vi "Maintenance4ChBK.vi"() -> ()   [LabVIEW 2020]
doc: "Maintanence VI for FLS imaging system.\n[Covers: REQ9]\n[Covers: REQ10]"
uses:
  SubVI/DigitizerConfiguration/FLImDAQ.ctl
  <instrlib>/niScope/Controls/niScope trigger source.ctl
  SubVI/LabJack/LJ Pin Setting.ctl
  <vilib>/addons/control/pid/autopid.llb/PID autotuning parameters.ctl
  LaguerreDeconLib/DeconEngineClass/LaguerreDeconEngineClass.lvclass/LaguerreDeconEngineClass.ctl
  <vilib>/Utility/error.llb/DialogType.ctl
  <vilib>/event_ctls.llb/usereventprio.ctl
  <vilib>/Utility/miscctls.llb/LVRowAndColumnTypeDef.ctl
  <vilib>/Utility/miscctls.llb/LVMinMaxIncTypeDef.ctl
  SubVI/APD/APDClass.lvclass
  SubVI/APD/GainData.ctl
  SubVI/APD/iRFData.ctl
  <vilib>/Analysis/baseanly.llb/Mean (DBL).vi
  SubVI/GlobalVariables.vi
  <vilib>/addons/control/pid/autopid.llb/PID Online Autotuning (Step Closed Loop).vi
  <vilib>/addons/control/pid/pid.llb/PID Advanced (DBL).vi
  <instrlib>/niScope/Acquire/Fetch/niScope Multi Fetch Binary 16.vi
  <vilib>/Instr/_visa.llb/VISA Configure Serial Port (Instr).vi
  <userlib>/_OpenG.lib/file/file.llb/openg_file.lvlib
  <userlib>/_OpenG.lib/time/time.llb/openg_time.lvlib
  <vilib>/Analysis/NI_AALBase.lvlib
  LaguerreDeconLib/DeconEngineClass/LaguerreDeconEngineClass.lvclass
  <vilib>/Utility/miscctls.llb/LVPointTypeDef.ctl
  <vilib>/addons/control/pid/NI_PID_autopid.lvlib
  <vilib>/addons/control/pid/NI_PID_pid.lvlib
panel:
  in  "Duty Cycle (%)":u32=25
  in  "AB Rep Rate":u16 caption="Rep Rate" max=1000 step=1 format="%.0dHz"
  in  "Current":dbl=1.0 min=1.0 max=63.0 step=1.0 format="%#.1fA"
  out "GainIndicator":dbl caption="Gain"
  out "Noise\n(std of DC)":dbl format="%0.6f"
  in  "BG flag?":bool
  out "DC":dbl format="%0.2f"
  out "Amplitude":dbl
  in  "Gain High":dbl max=4.5
  in  "Gain low":dbl=3.0
  in  "Step":dbl=0.1
  in  "Num WF to acquire":u64=18446744073709551615
  in  "Channel":enum32{"Ch1", "Ch2", "Ch3", "Ch4"}(radio)
  in  "Task":enum32{"iRFAndGain", "Alignment"}(radio)
  in  "Aiming beam toggle":bool caption="445nm 100Hz"
  in  "Laser Rep Rate":u16=120 caption="Rep Rate" min=5 max=4000 step=1 format="%.0dHz"
  in  "355nm Laser toggle":bool caption="355nm 460Hz"
  out "appended path":path
  out "Current State":string
  out "WF max value":dbl
  out "Disclamer":picture
  out "Calibration #":i8
  out "BG #":i8
  in  "TCP Connect":bool
  out "Help":string
  in  "Auto gain":bool=TRUE
  out "Run #":i8
  in  "StopButton":bool caption="Stop"
  out "System Status:":bool
  in  "StartButton":bool caption="Start"
  in  "Ctrl V":dbl=0.05 min=0.0 max=5.5 step=0.009999999776482582 format="%#.3f"
  out "System Hardware Connection Status":T1
  out "Waveform (no average)":dbl[](graph)
  in  "Tab Control":T2(tab)
  out "Ch1 Max CtrlV":dbl
  out "Ch1 iRF Graph":dbl[][](graph)
  out "Ch1 Gain":cluster{"CtrlV":dbl[], "Gain":dbl[]}(graph)
  out "Serial Number Ch1":string caption="Serial Number"
  out "DateTimeCh1":string caption="DateTime"
  out "Ch2 Gain":cluster{"CtrlV":dbl[], "Gain":dbl[]}(graph)
  out "Ch2 iRF Graph":dbl[][](graph)
  out "Ch2 Max CtrlV":dbl
  out "Serial Number Ch2":string caption="Serial Number"
  out "DateTimeCh2":string caption="DateTime"
  out "Ch3 iRF Graph":dbl[][](graph)
  out "Ch3 Gain":cluster{"CtrlV":dbl[], "Gain":dbl[]}(graph)
  out "Serial Number Ch3":string caption="Serial Number"
  out "Ch3 Max CtrlV":dbl
  out "DateTimeCh3":string caption="DateTime"
  out "Ch4 iRF Graph":dbl[][](graph)
  out "Ch4 Gain":cluster{"CtrlV":dbl[], "Gain":dbl[]}(graph)
  out "Serial Number Ch4":string caption="Serial Number"
  out "Ch4 Max CtrlV":dbl
  out "DateTimeCh4":string caption="DateTime"
  out "display loop timing(ms)":u32
  out "Aquisition loop timing(ms)":u32
  out "DisplayLoop":i32
  out "processing loop":i32
  out "processing loop timing(ms)":dbl
  out "laser EM lamp V":dbl format="%0.6f"
  out "aquisition loop Error Out":errorcluster
  out "Aq Loop?":bool
  out "processing Error Out":errorcluster
  out "Triggering:Trigger Delay":dbl
  out "Foot Pedal":bool
  out "LJ Pinout":T3={"Ch1 Bias"="DAC0", "Ch2 Bias"="DAC1", "Ch3 Bias"="DAC2", "Ch4 Bias"="DAC0", "355 PWM"="FIO0", "AimingBeam PWM"="FIO2", "Laser Ready"="FIO3", "Interlock"="FIO1", "Laser Start/Stop"="FIO1", "Red LED"="FIO1", "Green LED"="DIO3", "Foot Pedal"="DIO15"}
  out "FLImDAQ":T4={"Digitizer 1"="", "Digitizer 2"="", "Channel"=enum."Channel 0", "trigger source"="VAL_EXTERNAL", "trigger level"=0.5, "trigger delay"=1.35e-07, "min sample rate"=12500000000.0, "min record length"=2500, "vertical range"=1.0, "vertical offset"=-0.25, "Waveform to Avg"=2000} caption="FLIm DAQ Configuration" {"trigger delay" format="%^#.4e"; "trigger level" min=0.0 max=3.5 step=0.5 format="%.2f"; "vertical offset" format="%.4f"; "vertical range" format="%.2f"; "min sample rate" format="%#.2p"}
  out "Dig1 Temp":dbl
  out "Dig2 Temp":dbl
  in  "Sys Reconfig":bool
  out "Fetch Record #":i32
  out "Record Backlog":i32
  out "Fetch:Records Done":i32
  out "dt (s)":dbl format="%#_6p"
  out "Fetch:Records Done 2":i32
  in  "SaveData?":bool
  out "data Size":i32[](array[numeric])
  out "numWFInQ":i32
  in  "Clear WF Chart History":bool
  out "Waveform Chart":dbl(graph)
  in  "SaveiRFData":bool
  out "iRFDataTable":string[][](table)
  in  "SetIRFCtrlV":bool
  in  "ClearIRFData":bool
  in  "AcquireIRF":bool
  out "iRFInstSting":string="To aquire gain data, please start data aquisition! \nPlace blue (Ch1&2) or Green(Ch3) Chroma slide as close as possible to the fiber port! \nPlease remove channel 3 bandpass filter as well!"
  out "iRFSigInRange":bool caption="Signal  In Range?"
  out "Current iRF":dbl[](graph)
  out "iRFCtrlV":dbl[](array[numeric])
  in  "SaveGainData":bool
  out "GainInstSting":string="To aquire gain data, please start data aquisition! \nPlace blue (Ch1&2) or Green(Ch3) Chroma slide as close as possible to the fiber port! \nPlease remove channel 3 bandpass filter as well!"
  in  "ClearGainData":bool
  out "Gain":dbl[](array[numeric])
  in  "ComputeGain":bool
  out "Int Corr AUC":dbl[](array[numeric])
  out "AUC Std":dbl[](array[numeric])
  out "GainSigInRange":bool caption="Signal  In Range?"
  in  "AcquireGain":bool
  out "GainDataTable":string[][](table)
  out "Intensity Factor":dbl[](array[numeric])
  out "AUC":dbl[](array[numeric])
  out "Ctrl V":dbl[](array[numeric])
  out "XY Graph":cluster{"Ctrl V":dbl[], dbl[]}(graph)
  in  "Ch4 PID gains":T6={"proportional gain (Kc)"=0.5, "integral time (Ti, min)"=0.0003, "derivative time (Td, min)"=1e-05} {"derivative time (Td, min)" format="%.6f"; "integral time (Ti, min)" format="%.6f"; "proportional gain (Kc)" format="%.6f"}
  in  "Save PID":bool
  out "Targer and Max":cluster{"V target(1.0)":dbl, dbl}(graph)
  out "Completed?":bool
  out "Gain(Log10)":dbl(graph)
  in  "Gain(Log)":dbl=1.0
  in  "Ch1 PID gains":T6={"proportional gain (Kc)"=0.5, "integral time (Ti, min)"=0.0003, "derivative time (Td, min)"=1e-05} {"derivative time (Td, min)" format="%.6f"; "integral time (Ti, min)" format="%.6f"; "proportional gain (Kc)" format="%.6f"}
  in  "autotune? (F)":bool
  in  "PID dt (s)":dbl=-1.0
  out "dt out (s)":dbl format="%.3f"
  in  "V target(1.0)":dbl=1.0 format="%#_2f"
  in  "Accept?":bool
  out "tuned PID gains":T6={"proportional gain (Kc)"=1.0, "integral time (Ti, min)"=0.01, "derivative time (Td, min)"=0.0} {"derivative time (Td, min)" format="%_6f"; "integral time (Ti, min)" format="%.6f"; "proportional gain (Kc)" format="%.6f"}
  in  "autotuning parameters":T7={"type of controller"=2, "relay cycles"=100, "relay amplitude"=0.25, "control specifications"=1, "PV noise level"=0.01} {"PV noise level" format="%.5f"; "control specifications" items=["normal", "fast", "slow"]; "relay amplitude" format="%.2f"; "type of controller" items=["P", "PI", "PID"]}
  in  "Ch2 PID gains":T6={"proportional gain (Kc)"=0.5, "integral time (Ti, min)"=0.0003, "derivative time (Td, min)"=1e-05} {"derivative time (Td, min)" format="%.6f"; "integral time (Ti, min)" format="%.6f"; "proportional gain (Kc)" format="%.6f"}
  in  "Ch3 PID gains":T6={"proportional gain (Kc)"=0.5, "integral time (Ti, min)"=0.0003, "derivative time (Td, min)"=1e-05} {"derivative time (Td, min)" format="%.6f"; "integral time (Ti, min)" format="%.6f"; "proportional gain (Kc)" format="%.6f"}
  in  "gamma":dbl=1.0 format="%.2f"
  in  "alpha":dbl=nan format="%.2f"
  in  "Quit":bool
  # "440nm Laser Setting"
  # "355nm Laser Setting"
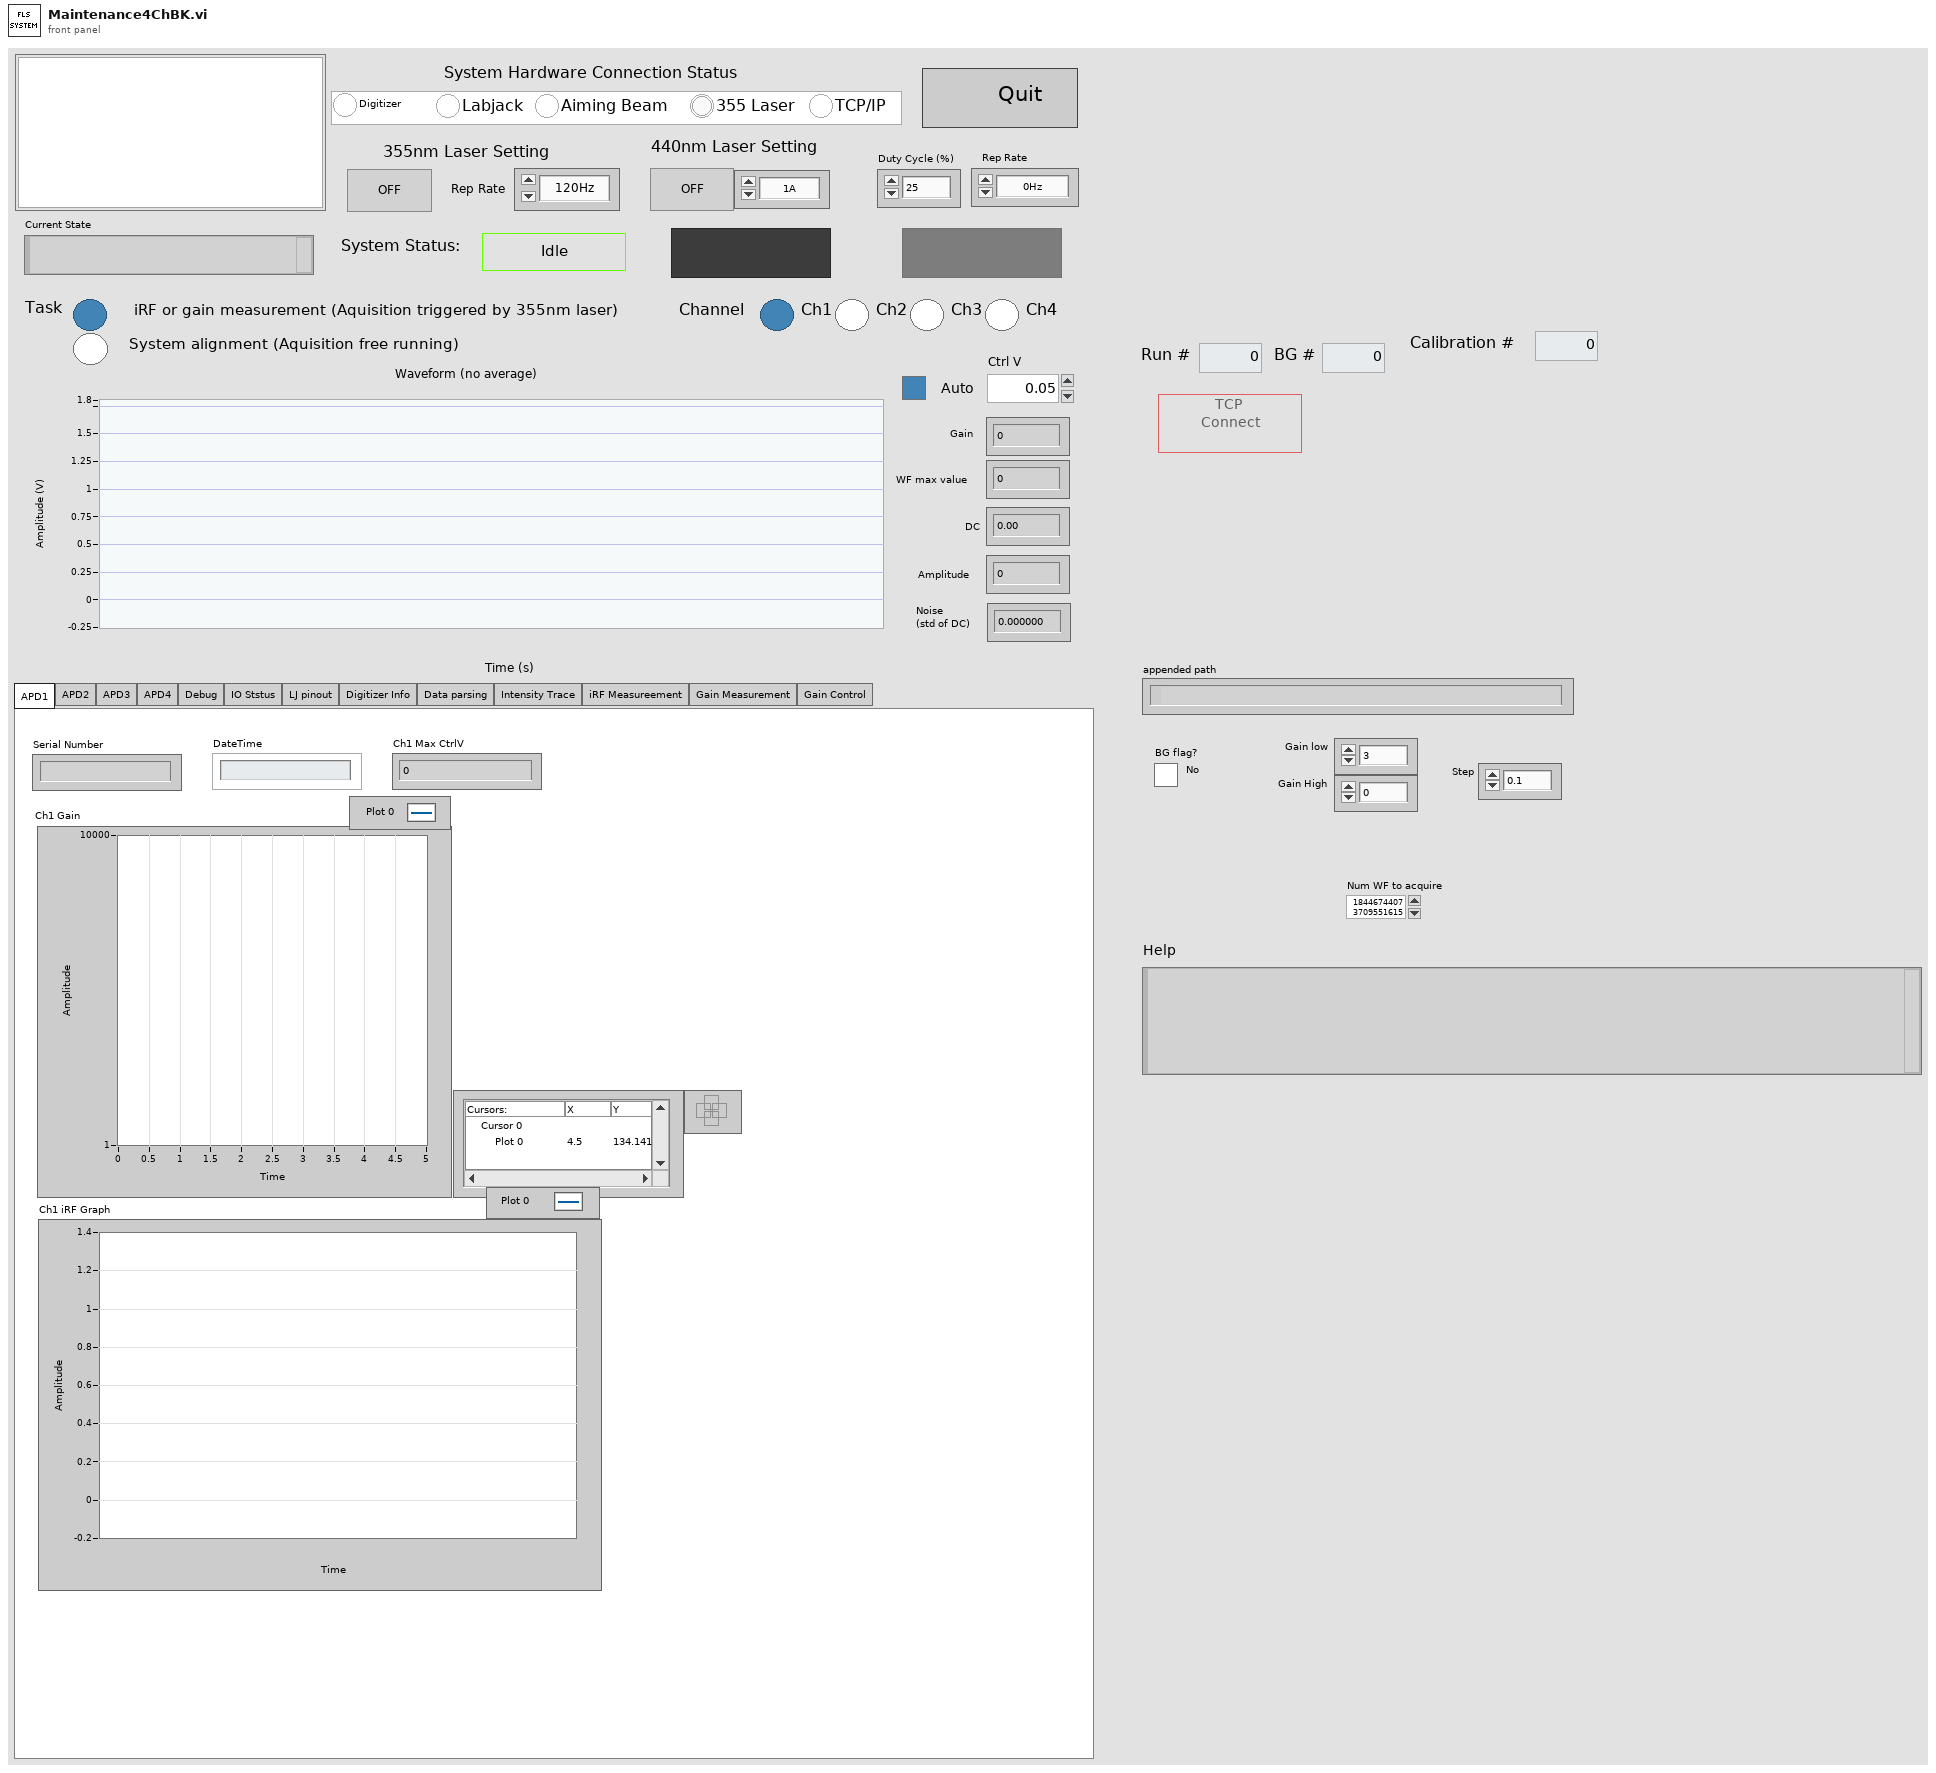
[diagram p1: front panel]
types:
  T1 = cluster{"Digitizer":bool, "Labjack":bool, "Aiming Beam":bool, "355 Laser":bool, "TCP/IP":bool}
  T2 = enum32{"APD1", "APD2", "APD3", "APD4", "Debug", "IO Ststus", "LJ pinout", "Digitizer Info", "Data parsing", "Intensity Trace", "iRF Measureement", "Gain Measurement", "Gain Control"}
  T3 = typedef "LJ Pin Setting.ctl" = cluster{"Ch1 Bias":string, "Ch2 Bias":string, "Ch3 Bias":string, "Ch4 Bias":string, "355 PWM":string, "AimingBeam PWM":string, "Laser Ready":string, "Interlock":string, "Laser Start/Stop":string, "Red LED":string, "Green LED":string, "Foot Pedal":string}
  T4 = typedef "FLImDAQ.ctl" = cluster{"Digitizer 1":refnum<k15>, "Digitizer 2":refnum<k15>, "Channel":enum16{"Channel 0", "Channel 1", "Channel 0&1"}, "trigger source":T5, "trigger level":dbl, "trigger delay":dbl, "min sample rate":dbl, "min record length":i32, "vertical range":dbl, "vertical offset":dbl, "Waveform to Avg":i16}
  T5 = typedef "niScope trigger source.ctl" = string
  T6 = cluster{"proportional gain (Kc)":dbl, "integral time (Ti, min)":dbl, "derivative time (Td, min)":dbl}
  T7 = typedef "PID autotuning parameters.ctl" = cluster{"type of controller":u16, "relay cycles":i32, "relay amplitude":dbl, "control specifications":u16, "PV noise level":dbl}
  T8 = cluster{"CtrlV":dbl, "WFs":dbl[][], "WFavg":dbl[]}
  T9 = enum16{"open", "replace", "create", "open or create", "replace or create", "replace or create with confirmation"}
  T10 = typedef "LVPointTypeDef.ctl" = cluster{"Horizontal":i16, "Vertical":i16}
  T11 = enum8{"Enabled", "Disabled", "Disabled and Grayed Out"}
  T12 = cluster{"CtrlV":dbl, "PeakV":dbl, "PeakV Std":dbl, "IntFactor":dbl, "IntCorrPeakV":dbl}
  T13 = enum16{"open", "open or create", "create or replace", "create", "open (read-only)"}
  T14 = enum32{"Invalid", "Standard", "Closed", "Hidden", "Minimized", "Maximized"}
  T15 = enum32{"invalid app kind", "Development System", "Run Time System", "Student Edition", "Embedded LabVIEW", "Evaluation", "Custom"}
  T16 = typedef "usereventprio.ctl" = enum32{"high priority", "normal priority"}
  T17 = enum32{"APD1", "APD2", "APD3", "Debug", "IO Ststus", "LJ pinout", "Digitizer Info", "Data parsing"}
  T18 = enum32{"Bad", "Idle", "Run top level", "Running"}
  T19 = typedef "LVRowAndColumnTypeDef.ctl" = cluster{"Row":i32, "Column":i32}
  T20 = typedef "LVMinMaxIncTypeDef.ctl" = cluster{"Minimum":dbl, "Maximum":dbl, "Increment":dbl}
  T21 = cluster{"Aiming Beam COM Port":refnum<visa-resource-name>, "Min Current":dbl, "Max Current":dbl, "Default Current":dbl, "Frequency(Hz)":i32}
  T22 = cluster{"Core":cluster{"Current VI Reference":refnum<vi>, "Close Panel on Exit?":bool}, "SysConfigCluster":cluster{"Ch1Enable?":bool, "Ch2Enable?":bool, "Ch3Enable?":bool, "Ch1AutoGain?":bool, "Ch2AutoGain?":bool, "Ch3AutoGain?":bool, "AimingBeamEnable?":bool}, "System Status":cluster{"Digitizer":bool, "Labjack":bool, "Aiming Beam":bool, "355 Laser":bool, "TCP/IP":bool}, "IDs":cluster{"RunID":i8, "BG ID":i8, "Cali ID":i8}, "DefaultPath":path, "Pathes":cluster{"DataPath":path, "BG Path":path, "iRFPath":path, "CaliPath":path}, "FLImDAQ":cluster{"resource name":refnum<k15>, "resource name 2":refnum<k15>, "Channel":enum16{"Channel 0", "Channel 1", "Channel 0&1"}, "trigger source":T5, "trigger level":dbl, "trigger delay":dbl, "min sample rate":dbl, "min record length":i32, "vertical range":dbl, "vertical offset":dbl, "Waveform to Avg":i32}, "SysRunning?":bool, "AB Cluster":cluster{"Aiming Beam COM Port":refnum<visa-resource-name>, "Min Current":dbl, "Max Current":dbl, "Default Current":dbl, "Frequency(Hz)":i32}, "LJ Pinout":T3, "355 PWM setting":cluster{"DIO_EF_CLOCK1_DIVISOR":i16, "DIO_EF_CLOCK1_ROLL_VALUE":i32, "DIO#_EF_INDEX":i16, "DIO#_EF_OPTIONS":i16, "DIO#_EF_CONFIG_A":i32}, "AB PWM setting":cluster{"DIO_EF_CLOCK1_DIVISOR":i16, "DIO_EF_CLOCK1_ROLL_VALUE":i32, "DIO#_EF_INDEX":i16, "DIO#_EF_OPTIONS":i16, "DIO#_EF_CONFIG_A":i32}, "Last Trigger":u32, "niTClk sessions":refnum<k20>[], "Laser start tic":u32, "TCP attempt count":i32, "iRFAllGain":dbl[][], "SlowTimer":u32, "FastTimer":u32, "TempPath":path, "LED vi reference":refnum<vi>, "APDSerials":cluster{"Ch1Serial":string, "Ch2Serial":string, "Ch3Serial":string, "Ch4Serial":string}, "LedViRefOpen":bool, "GainBGRaw":dbl[][], "GainDataTemp":cluster{"CtrlV":dbl, "AUC":dbl, "AUC Std":dbl, "IntFactor":dbl, "IntCorrAUC":dbl}, "iRFIdx":i32}
  T23 = cluster{"CtrlV":dbl, "AUC":dbl, "AUC Std":dbl, "IntFactor":dbl, "IntCorrAUC":dbl}
  T24 = cluster{"Ch1Serial":string, "Ch2Serial":string, "Ch3Serial":string, "Ch4Serial":string}
  T25 = cluster{"DataPath":path, "BG Path":path, "iRFPath":path, "CaliPath":path}
  T26 = cluster{"DIO_EF_CLOCK1_DIVISOR":i16, "DIO_EF_CLOCK1_ROLL_VALUE":i32, "DIO#_EF_INDEX":i16, "DIO#_EF_OPTIONS":i16, "DIO#_EF_CONFIG_A":i32}
  T27 = cluster{"resource name":refnum<k15>, "resource name 2":refnum<k15>, "Channel":enum16{"Channel 0", "Channel 1", "Channel 0&1"}, "trigger source":T5, "trigger level":dbl, "trigger delay":dbl, "min sample rate":dbl, "min record length":i32, "vertical range":dbl, "vertical offset":dbl, "Waveform to Avg":i32}
  T28 = cluster{"Ch1Enable?":bool, "Ch2Enable?":bool, "Ch3Enable?":bool, "Ch1AutoGain?":bool, "Ch2AutoGain?":bool, "Ch3AutoGain?":bool, "AimingBeamEnable?":bool}
  T29 = cluster{"Current VI Reference":refnum<vi>, "Close Panel on Exit?":bool}
  T30 = cluster{"iRF":dbl[], "iRF":dbl[], "iRF":dbl[], "iRF":dbl[]}
  T31 = typedef "DialogType.ctl" = u16
  T32 = typedef "LJ PWM Setting.ctl" = cluster{"DIO_EF_CLOCK1_DIVISOR":i16, "DIO_EF_CLOCK1_ROLL_VALUE":i32, "DIO#_EF_INDEX":i16, "DIO#_EF_OPTIONS":i16, "DIO#_EF_CONFIG_A":i32}
  T33 = typedef "AimingBeam.ctl" = cluster{"Aiming Beam COM Port":refnum<visa-resource-name>, "Min Current":dbl, "Max Current":dbl, "Default Current":dbl, "Frequency(Hz)":u32}
  T34 = typedef "LVBoundsTypeDef.ctl" = cluster{"Width":u32, "Height":u32}
  T35 = typedef "imagedata.ctl" = cluster{"image type":i32, "image depth":i32, "image":u8[], "mask":u8[], "colors":u32[], "Rectangle":cluster{"left":i16, "top":i16, "right":i16, "bottom":i16}}
  T36 = typedef "LVCursorListTypeDef.ctl" = cluster{"Name":string, "Color":u32, "Style":u8, "Point Style":u8, "Name Visible":bool, "Allow Drag":bool, "Cursor Mode":u32, "Plot":i32, "Index":i32, "Position":cluster{"X":dbl, "Y":dbl}, "X Scale":u32, "Y Scale":u32, "Watch Plots":i32[], "Watch All Plots":bool, "Plot Area":i32, "Label Offset":cluster{"X":dbl, "Y":dbl}}[]
  T37 = cluster{"Name":string, "Color":u32, "Style":u8, "Point Style":u8, "Name Visible":bool, "Allow Drag":bool, "Cursor Mode":u32, "Plot":i32, "Index":i32, "Position":cluster{"X":dbl, "Y":dbl}, "X Scale":u32, "Y Scale":u32, "Watch Plots":i32[], "Watch All Plots":bool, "Plot Area":i32, "Label Offset":cluster{"X":dbl, "Y":dbl}}
  T38 = cluster{"Name":string, "Color":u32, "Style":u8, "Point Style":u8, "Name Visible":bool, "Allow Drag":bool, "Cursor Mode":u32, "Plot":i32, "Index":i32, "Position":cluster{"X":dbl, "Y":dbl}, "X Scale":u32, "Y Scale":u32, "Watch Plots":i32[], "Watch All Plots":bool, "Plot Area":i32, "Label Offset":cluster{"X":dbl, "Y":dbl}}[]
  T39 = cluster{"Ch1APDSerial#":string, "Ch2APDSerial#":string, "Ch3APDSerial#":string, "Ch4APDSerial#":string}
  T40 = typedef "GainData.ctl" = cluster{"CtrlV":dbl[], "NumOfWFs":i32, "WF length":i32, "Gain":dbl[], "GainRaw":dbl[][], "GainBGRaw":dbl[][]}
  T41 = typedef "iRFData.ctl" = cluster{"dt":dbl, "NumOfWFs":i32, "WFLength":i32, "iRFCtrlV":dbl[], "iRFWFsAvg":dbl[][], "iRFRaw":dbl[][]}
  T42 = cluster{"CtrlV":dbl, "WFs":dbl[][], "WFavg":dbl[]}[]
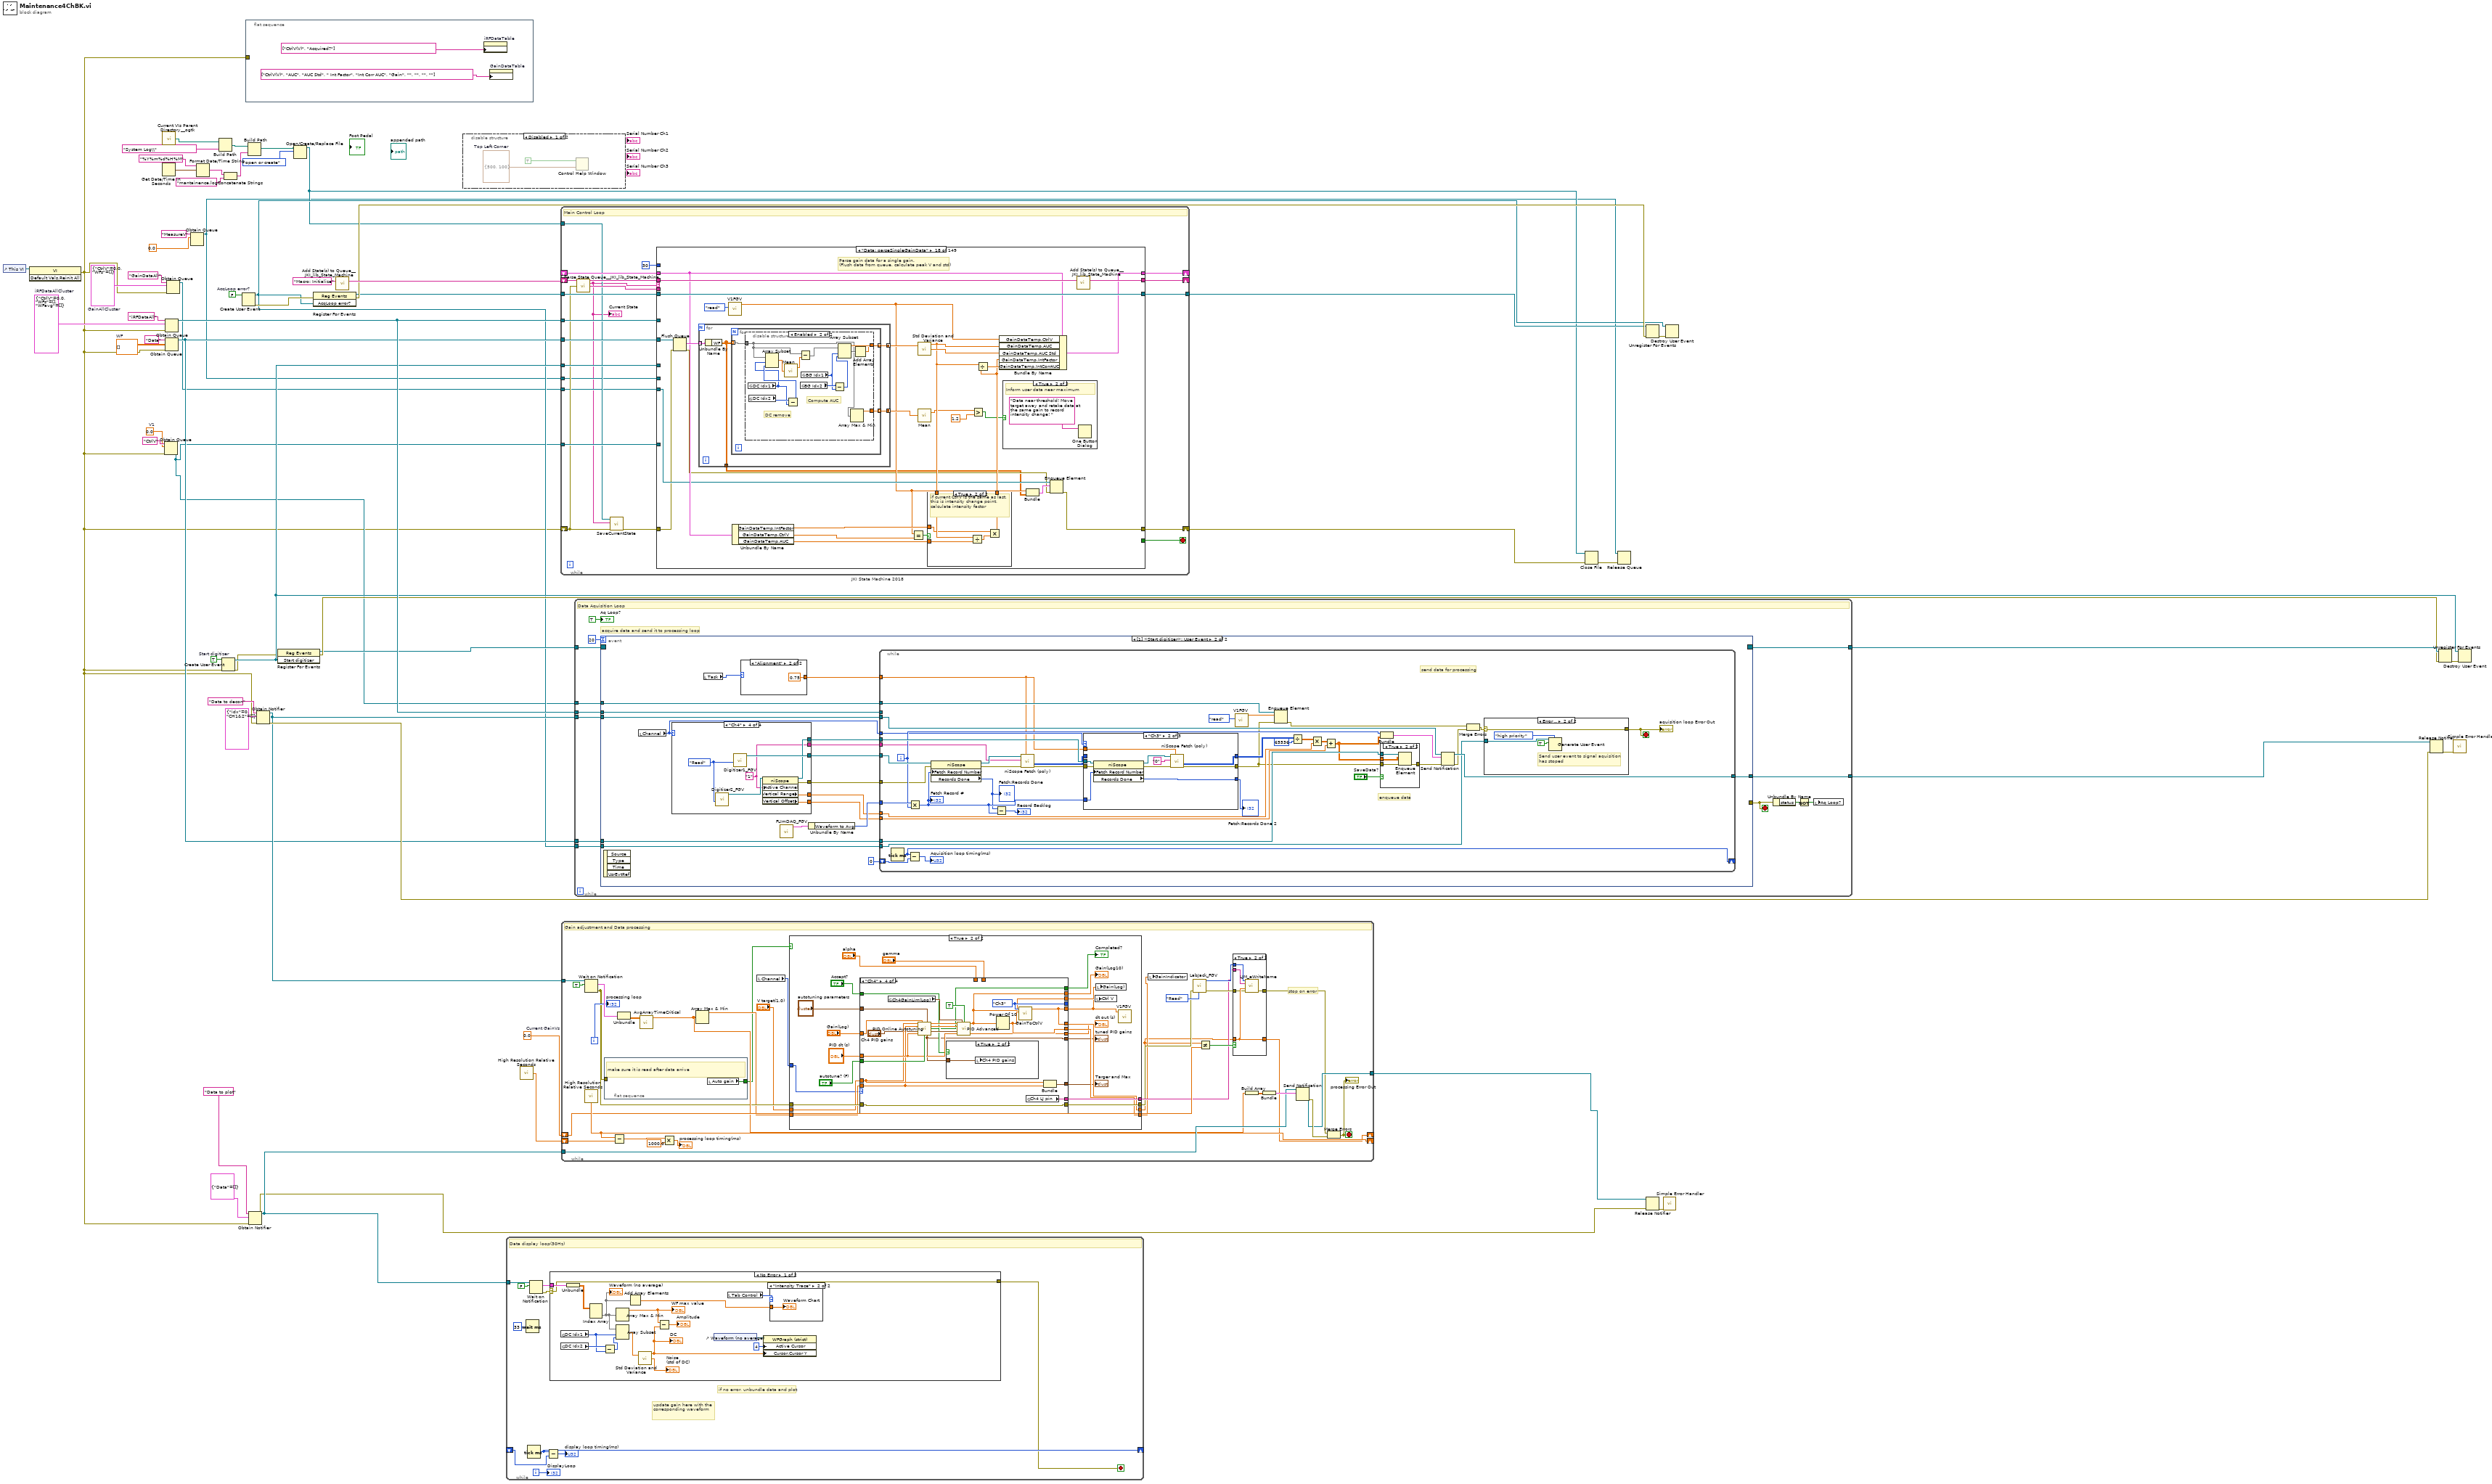
[diagram p0: block diagram]
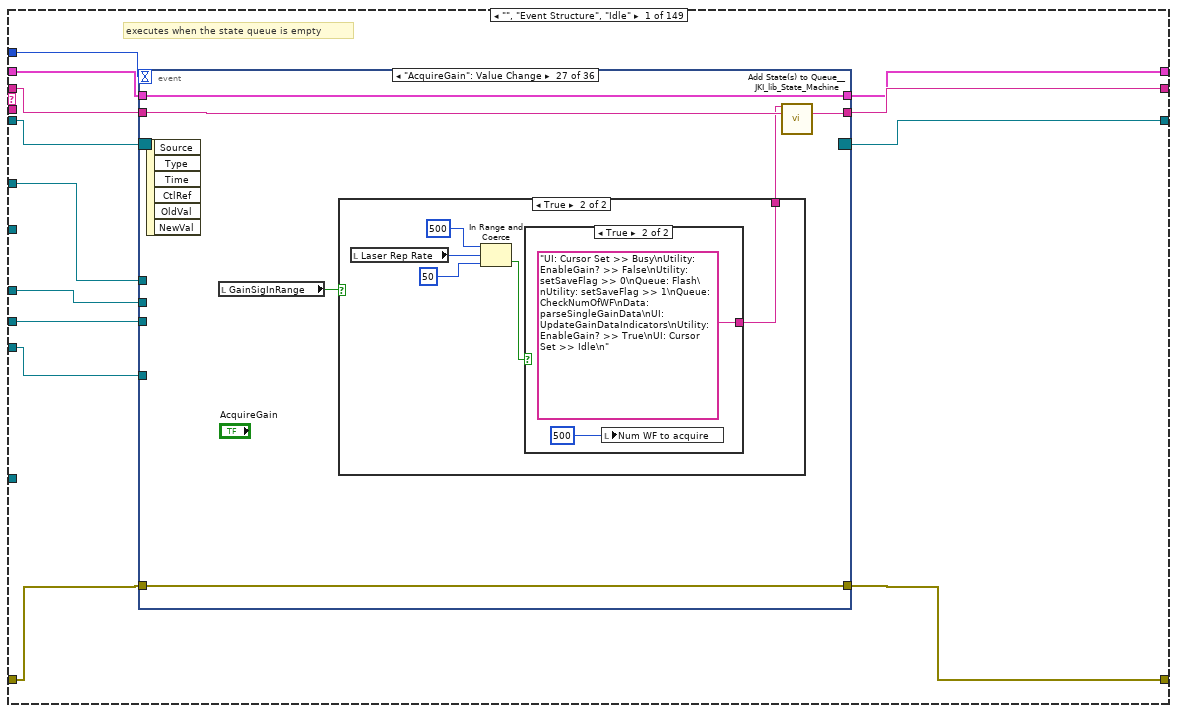
[diagram p3: hidden frame]
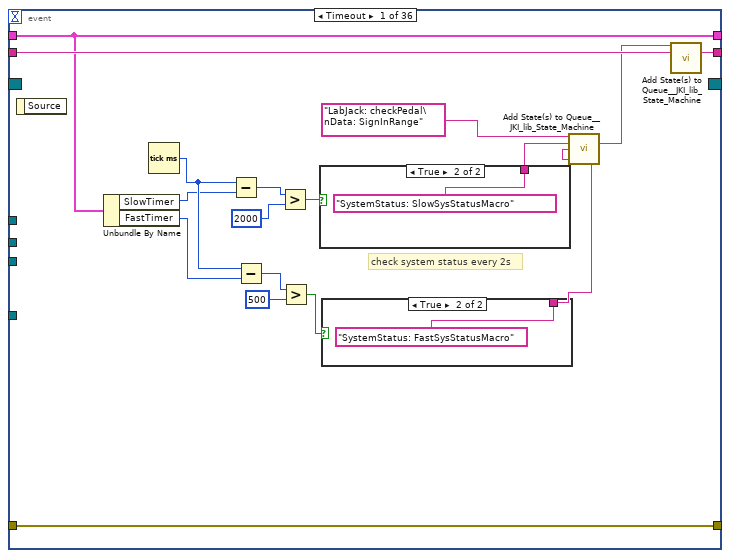
[diagram p4: hidden frame]
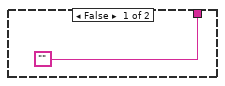
[diagram p5: hidden frame]
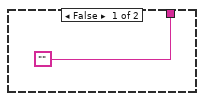
[diagram p6: hidden frame]
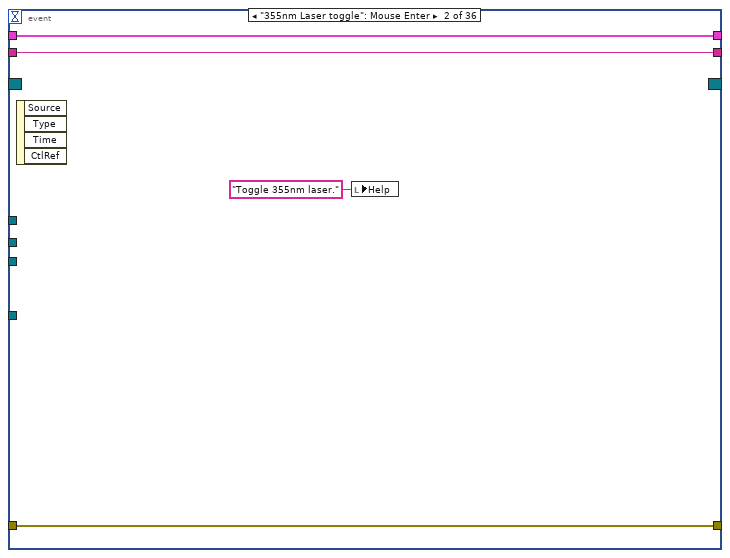
[diagram p7: hidden frame]
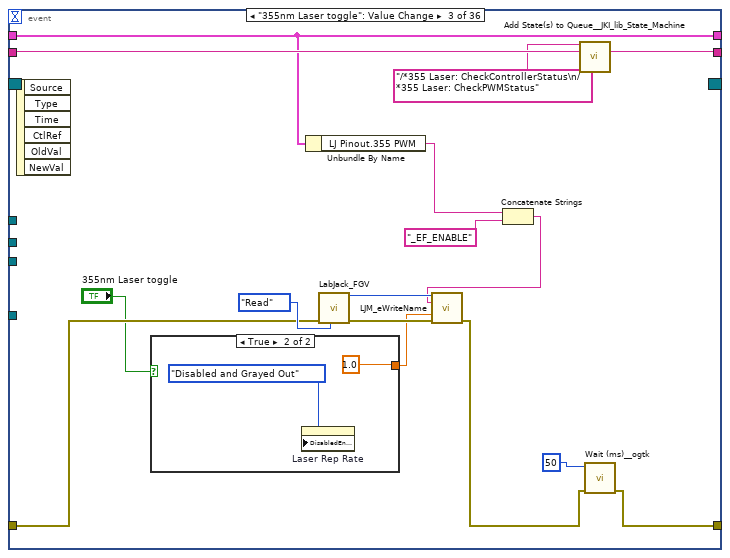
[diagram p8: hidden frame]
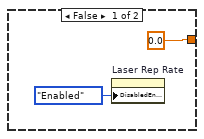
[diagram p9: hidden frame]
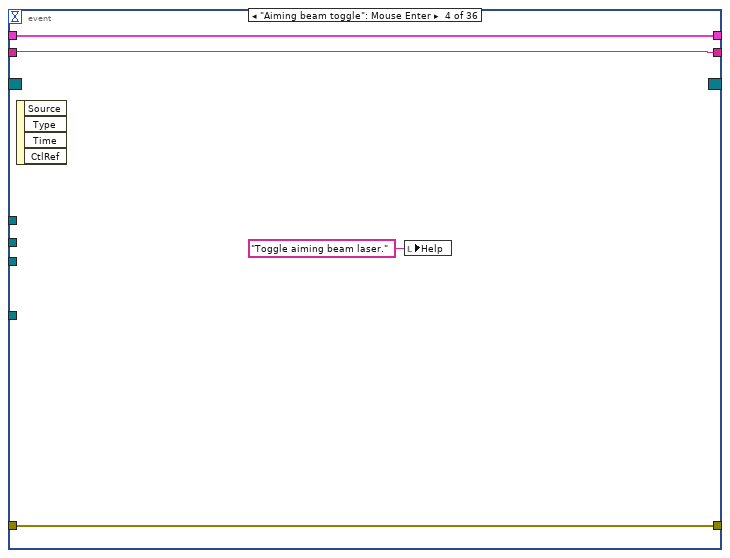
[diagram p10: hidden frame]
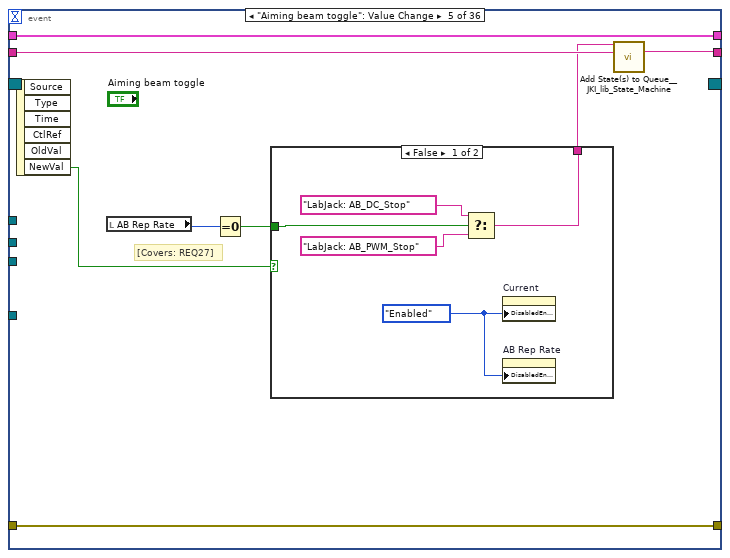
[diagram p11: hidden frame]
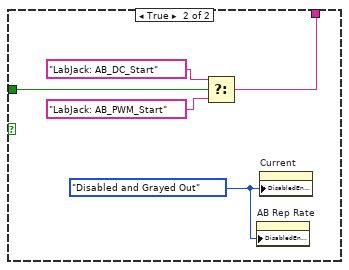
[diagram p12: hidden frame]
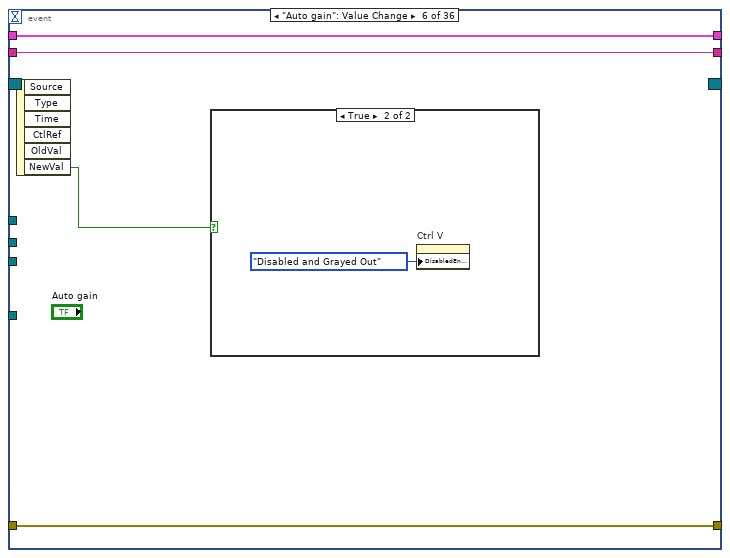
[diagram p13: hidden frame]
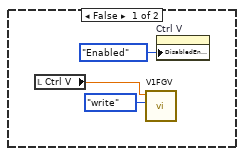
[diagram p14: hidden frame]
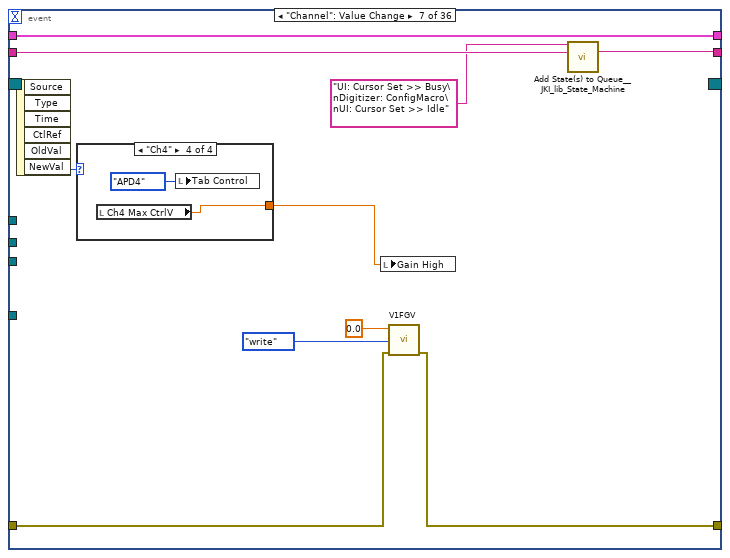
[diagram p15: hidden frame]
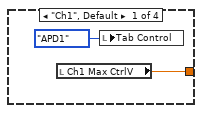
[diagram p16: hidden frame]
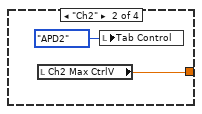
[diagram p17: hidden frame]
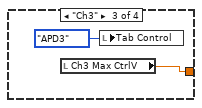
[diagram p18: hidden frame]
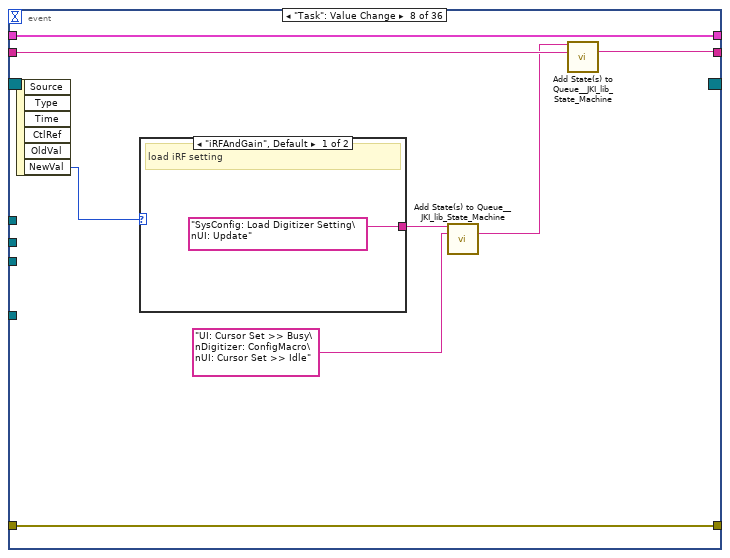
[diagram p19: hidden frame]
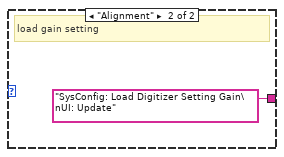
[diagram p20: hidden frame]
diagram:
  w3 = cluster{"CtrlV":dbl, "WFs":dbl[][]} {"CtrlV"=0.0, "WFs"=[]}  # GainAllCluster
  w5 = T8 {"CtrlV"=0.0, "WFs"=[], "WFavg"=[]}  # iRFDataAllCluster
  w22 = 0.0  # V1
  w26 = 0.0  # Current GainVs
  w43 = FALSE  # AcqLoop error?
  w53 = TRUE  # Start digitizer
  w56 = dbl[][] []  # WF
  n1 = control-ref of="This VI"() -> (w58:refnum<vi>)
  n2 = invoke on="Invoke Node" class="VI" method="Default Vals.Reinit All"(reference=w58) -> (error out=w1:errorcluster)  [unwired: 2 in, 2 out]
  n3 = call <userlib>:"Current VIs Parent Directory__ogtk.vi"() -> ("Parent Directory (+ Relative)"=w21:path)  [unwired: 5 in]
  n4 = Get Date/Time In Seconds() -> (seconds since 1Jan1904=w19:timestamp)
  n5 = Obtain Queue(name (unnamed)="CtrlV", element data type=w22, error in (no error)=w1) -> (queue out=w24:refnum<queue>)  [unwired: 2 in, 2 out]
  n6 = Obtain Queue(name (unnamed)="Data", element data type=w56, error in (no error)=w1) -> (queue out=w32:refnum<queue>)  [unwired: 2 in, 2 out]
  n7 = Obtain Queue(name (unnamed)="iRFDataAll", element data type=w5, error in (no error)=w1) -> (queue out=w54:refnum<queue>)  [unwired: 2 in, 2 out]
  n8 = Obtain Queue(name (unnamed)="GainDataAll", element data type=w3, error in (no error)=w1) -> (queue out=w2:refnum<queue>)  [unwired: 2 in, 2 out]
  n9 = Obtain Queue(name (unnamed)="MeasureV", element data type=0.0) -> (queue out=w6:refnum<queue>)  [unwired: 3 in, 2 out]
  n10 = Format Date/Time String(time format string (%c)="%Y%m%d%H%M", seconds (now)=w19) -> (date/time string=w16:string)  [unwired: 1 in]
  n11 = Build Path(base path=w21, name or relative path="System Log\\") -> (appended path=w12:path)
  n12 = Create User Event(user event datatype=w53, error in=w1) -> (user event=w42:refnum<user-event>, error out=w28:errorcluster)
  n13 = Concatenate Strings(w16, "mantainence.log" ("string")) -> (w14:string)
  n14 = Create User Event(user event datatype=w43) -> (user event=w27:refnum<user-event>, error out=w29:errorcluster)  [unwired: 1 in]
  n15 = flat-sequence {
    tunnel: w1 -> [_]
    frame #0 {
      n16 = property on="iRFDataTable" class="Tbl (strict)"("Column Headers[]"=string[] ["CtrlV(V)", "Acquired?"] ("Column Header Strings[]")) -> ()  [unwired: 2 in, 2 out]
      n17 = property on="GainDataTable" class="Tbl (strict)"("Column Headers[]"=string[] ["CtrlV(V)", "AUC", "AUC Std", " Int Factor", "Int Corr AUC", "Gain", "", "", "", ""] ("Column Header Strings[]")) -> ()  [unwired: 2 in, 2 out]
    }
  }
  n18 = Build Path(base path=w12, name or relative path=w14) -> (appended path=w17:path)
  n19 = Obtain Notifier(name (unnamed)="Data to plot", notification data type=cluster{"Data":dbl[][]} {"Data"=[]}, error in (no error)=w1) -> (notifier out=w36:refnum<notifier>, error out=w33:errorcluster)  [unwired: 1 in, 1 out]
  n20 = Obtain Notifier(name (unnamed)="Data to decon", notification data type=cluster{"idx":i32, "CH1&2":dbl[][]} {"idx"=0, "CH1&2"=[]}, error in (no error)=w1) -> (notifier out=w39:refnum<notifier>, error out=w47:errorcluster)  [unwired: 1 in, 1 out]
  n21 = register-events(error in=w28, w42) -> (reference out=w44:refnum<event-registration>, error out=w50:errorcluster)  [unwired: 1 in]
  n22 = Open/Create/Replace File(file path (use dialog)=w17, operation (0:open)=T9."open or create") -> (refnum out=w10:refnum<file>)  [unwired: 4 in, 2 out]
  n23 = register-events(error in=w29, w27) -> (reference out=w31:refnum<event-registration>, error out=w40:errorcluster)  [unwired: 1 in]
  n24 = call <vilib>:"Add State(s) to Queue__JKI_lib_State_Machine.vi"("State(s) in (\"\")"="Macro: Initialize") -> ("States Out"=w60:string)  [unwired: 14 in]
  n25 = disable-structure "Diagram Disable Structure" shown="Disabled" {
    frame Disabled {
      w63 = T10 {"Horizontal"=500, "Vertical"=100}  # Top Left Corner
      n26 = Control Help Window(0:w63, 1:TRUE ("Show")) -> ()
    }
    frame Enabled {
    }
  }
  n27 = while {
    tunnel: w36 -> [w74]
    shift-right: [w68] -> _
    shift-left: _ -> [w72]
    i -> [w66]
    stop <- w65 stop-if-true
    # "if no error, unbundle data and plot"
    # "update gain here with the corresponding waveform"
    # "Data display loop(30Hz)"
    n28 = Wait (ms)(milliseconds to wait=u32 33) -> ()  [unwired: 1 out]
    n29 = Tick Count (ms)() -> (millisecond timer value=w68:u32)
    n30 = Wait on Notification(notifier=w74, ignore previous (F)=FALSE) -> (notification=w69:cluster{"Data":dbl[][]}, error out=w67:errorcluster)  [unwired: 2 in, 2 out]
    n31 = Subtract(x=w68, y=w72) -> (x-y=→"display loop timing(ms)":u32)
    n32 = case shown="No Error" w67 {
      selector: w67 -> [w83 w92]
      tunnel: w69 -> [w90 _]
      tunnel: [w83 w92] -> w65
      frame No Error {
        n33 = global read "GlobalVariables.vi" "DC Idx1"() -> (w76:i32)
        n34 = global read "GlobalVariables.vi" "DC Idx2"() -> (w77:i32)
        n35 = Unbundle(w90) -> ("Data"=w87:dbl[][])
        n36 = Index Array(array=w87) -> (element=w86:dbl[])  [unwired: 2 in]
        "Waveform (no average)" <- w86
        n37 = Subtract(x=w77, y=w76) -> (x-y=w75:i32)
        n38 = Array Max & Min(array=w86) -> (max value=w89:dbl)  [unwired: 3 out]
        "WF max value" <- w89
        n39 = Array Subset(array=w86, index=w76, length=w75) -> (w82:dbl[])
        n40 = Add Array Elements(numeric array=w86) -> (sum=w85:dbl)
        n41 = call <vilib>:"Std Deviation and Variance.vi"("X"=w82) -> ("mean"=w78:dbl, "standard deviation"=→"Noise\n(std of DC)":dbl)  [unwired: 1 in, 1 out]
        "DC" <- w78
        n42 = Subtract(x=w89, y=w78) -> (x-y=→"Amplitude":dbl)
        n43 = control-ref of="Waveform (no average)"() -> (w80:refnum<vi>)
        n44 = local read "Tab Control"() -> (w84:T2)
        n45 = property class="WFGraph (strict)"(reference=w80, "Active Cursor"=u32 4, "Cursor.Cursor Y"=w78) -> ()  [unwired: 1 in, 2 out]
        n46 = case shown="\"Intensity Trace\"" w84 {
          tunnel: w85 -> [_ w91]
          frame "APD1", Default {
          }
          frame "Intensity Trace" {
            "Waveform Chart" <- w91
          }
        }
      }
      frame Error {
      }
    }
    "DisplayLoop" <- w66
  }
  n47 = call <vilib>:"High Resolution Relative Seconds.vi"() -> ("relative seconds"=w23:dbl)
  n48 = while "JKI State Machine 2018" {
    shift-right: [w109] -> _
    shift-left: _ -> [w108]
    shift-right: [w99] -> w11
    shift-left: w1 -> [w98]
    shift-right: [w110] -> _
    shift-left: w60 -> [w111]
    tunnel: w54 -> [w106]
    tunnel: w32 -> [w105]
    tunnel: w42 -> [w104]
    tunnel: w31 -> [w103]
    tunnel: [w102] -> w30
    tunnel: w24 -> [w100]
    tunnel: w10 -> [w96]
    tunnel: w6 -> [w95]
    tunnel: w2 -> [w94]
    stop <- w101 stop-if-true
    # "Main Control Loop"
    n49 = call <vilib>:"Parse State Queue__JKI_lib_State_Machine.vi"("State Queue"=w111, "Error In (no error)"=w98) -> ("Remaining States"=w113:string, "Current State"=w93:string, "Arguments"=w112:string)  [unwired: 11 in]
    "Current State" <- w93
    n50 = call "SaveCurrentState.vi"("error in (no error)"=w98, "Current State"=w93, "Byte Stream File in"=w96) -> ("error out"=w97:errorcluster)  [unwired: 8 in]
    n51 = case shown="\"Data: parseSingleGainData\"" w93 {
      selector: w93 -> [_ _ _ _ _ _ _ _ _ _ _ _ _ _ _ _ _ _ _ _ _ _ w832 _ _ _ _ _ _ _ _ _ _ _ _ _ _ _ _ _ _ _ _ _ _ _ _ _ _ _ _ _ _ _ _ _ _ _ _ _ _ _ _ _ _ _ _ _ _ _ _ _ _ _ _ _ _ _ _ _ _ _ _ _ _ _ _ _ _ _ _ _ _ _ _ _ _ _ _ _ _ _ _ _ _ _ _ _ _ _ _ _ _ _ _ _ _ _ _ _ _ _ _ _ _ _ _ _ _ _ _ _ _ _ _ _ _ _ _ _ _ _ _ _ _ _ _ _ _]
      tunnel: w113 -> [w126 w461 w470 w476 w483 w492 w503 w512 w537 w552 w583 w589 w614 w635 w652 w664 w695 w728 w783 w818 w825 w830 w836 w861 w869 w893 w898 w910 w919 w936 w944 w960 w984 w989 w999 w1024 w1052 w1075 w1119 w1171 w1202 w1225 w1250 w1282 w1305 w1354 w1369 w1385 w1390 w1401 w1412 w1428 w1466 w1483 w1497 w1531 w1542 w1548 w1559 w1571 w1602 w1634 w1647 w1660 w1674 w1688 w1693 w1705 w1717 w1730 w1743 w1759 w1787 w1802 w1807 w1816 w1854 w1867 w1875 w1883 w1897 w1902 w1908 w1925 w1942 w1959 w1979 w2004 w2012 w2017 w2025 w2033 w2038 w2047 w2086 w2126 w2131 w2154 w2167 w2185 w2191 w2202 w2215 w2233 w2240 w2252 w2317 w2328 w2341 w2366 w2389 w2395 w2401 w2416 w2461 w2469 w2475 w2480 w2486 w2494 w2503 w2513 w2519 w2525 w2530 w2536 w2549 w2583 w2592 w2604 w2630 w2656 w2678 w2684 w2709 w2734 w2759 w2784 w2801 w2864 w2922 w2941 w2951 w2974 w2979 w3001 w3010 w3019 w3024]
      tunnel: w112 -> [_ _ _ _ _ _ _ _ _ _ _ _ _ _ _ _ _ _ _ _ _ _ _ _ _ _ _ _ _ _ w943 _ _ _ _ _ _ _ _ _ _ _ _ _ _ _ _ _ _ _ _ _ _ _ _ _ _ _ _ w1569 _ _ _ _ _ _ _ _ _ _ _ _ _ _ _ _ _ _ _ _ _ _ _ _ _ _ _ _ _ _ _ _ _ _ _ _ _ w2145 _ _ _ _ _ _ w2235 w2247 _ _ _ _ w2385 _ _ _ _ _ _ _ w2481 _ w2495 w2508 _ _ _ _ _ _ _ _ _ _ _ _ _ _ _ _ _ _ _ _ _ w2965 _ _ _ _ _]
      tunnel: w108 -> [w124 w458 w466 w473 w479 w486 w500 w510 w521 w549 _ w586 w608 w626 w649 w655 w692 w722 w765 w792 w819 w827 w834 w844 w866 w891 w895 w900 w912 w921 w937 w956 w976 w986 w996 w1021 w1036 w1059 w1084 w1136 w1187 w1209 w1232 w1264 w1302 w1341 w1367 w1371 w1387 w1394 w1405 w1417 w1454 w1470 w1487 w1507 w1540 w1545 w1549 w1561 w1579 w1612 w1636 w1649 w1663 w1676 w1690 w1702 w1714 w1725 w1737 w1754 w1775 w1790 w1804 w1812 w1852 w1864 w1872 w1881 w1895 w1899 w1906 w1909 w1926 w1944 w1960 w1985 w2008 w2014 w2018 w2026 w2035 w2044 w2081 w2107 w2138 w2151 w2165 w2182 w2188 w2195 w2207 w2229 w2238 w2245 w2314 w2319 w2333 w2358 w2386 w2392 w2398 w2402 w2448 w2466 w2472 w2477 w2483 w2491 w2500 w2510 w2516 w2522 w2527 w2533 w2547 w2581 w2589 w2602 w2615 w2642 w2676 w2681 w2706 w2732 w2757 w2782 w2795 w2858 w2920 w2938 w2949 w2966 w2976 w2980 w3007 w3017 w3021]
      tunnel: [w123 w459 w468 w474 w481 w490 w501 w504 w535 w550 w581 w587 w604 w620 w650 w659 w693 w703 w771 w798 w822 w828 w838 w859 errorcluster {"status"=FALSE, "code"=0, "source"=""} ("error out") w890 w896 w905 w917 w928 w941 w955 w978 w987 w997 w1019 w1044 w1067 w1110 w1162 w1194 w1217 w1243 w1275 w1297 w1343 w1357 w1375 w1388 w1391 w1402 w1422 w1455 w1477 w1490 w1511 w1534 w1546 w1557 w1563 w1584 w1616 w1639 w1652 w1664 w1680 w1691 w1695 w1707 w1726 w1738 w1748 w1777 w1792 w1805 w1809 w1847 w1865 w1873 w1878 w1892 w1900 w1903 w1914 w1931 w1954 w1974 w1999 w2005 w2015 w2023 w2031 w2036 w2045 w2084 w2124 w2139 w2152 w2164 w2183 w2189 w2200 w2213 w2231 w2236 w2249 w2315 w2325 w2337 w2361 w2387 w2393 w2399 w2407 w2453 w2467 w2473 w2478 w2484 w2492 w2501 w2511 w2517 w2523 w2528 w2534 w2542 w2578 w2590 w2599 w2614 w2641 w2662 w2682 w2696 w2710 w2736 w2760 w2796 w2860 w2914 w2939 w2945 w2968 w2977 w2981 w3008 w3015 w3022] -> w99
      tunnel: w97 -> [w122 w459 w468 w474 w481 w490 w501 w504 w535 w550 w581 w587 w609 w630 w650 w661 w693 w702 w770 w807 w823 w828 w837 w859 w862 w890 w896 w906 w916 w927 w940 w957 w977 w987 w997 w1018 w1046 w1069 w1113 w1165 w1196 w1219 w1244 w1276 w1296 w1342 w1358 w1377 w1388 w1397 w1408 w1421 w1456 w1478 w1495 w1515 w1533 w1546 w1555 w1566 w1583 w1604 w1638 w1651 w1668 w1679 w1691 w1694 w1706 w1727 w1740 w1755 w1776 w1793 w1805 w1808 w1845 w1865 w1873 w1876 w1886 w1900 w1903 w1920 w1937 w1953 w1973 w1998 w2006 w2015 w2023 w2031 w2036 w2045 w2084 w2124 w2139 w2152 w2164 w2183 w2189 w2200 w2213 w2231 w2237 w2250 w2315 w2325 w2335 w2364 w2387 w2393 w2399 w2411 w2452 w2467 w2473 w2478 w2484 w2492 w2501 w2511 w2517 w2523 w2528 w2534 w2540 w2577 w2590 w2595 w2611 w2638 w2660 w2682 w2685 w2711 w2735 w2776 w2798 w2859 w2916 w2939 w2944 w2969 w2977 w2982 w3008 w3014 w3022]
      tunnel: [w125 w460 w469 w475 w482 w491 w502 w511 w536 w551 w582 w588 w613 w634 w651 w663 w694 w727 w782 w817 w824 w829 w835 w860 w868 w892 w897 w909 w918 w935 w944 w959 w983 w988 w998 w1023 w1051 w1074 w1118 w1170 w1201 w1224 w1249 w1281 w1304 w1353 w1368 w1384 w1389 w1400 w1411 w1427 w1465 w1482 w1496 w1530 w1541 w1547 w1558 w1570 w1601 w1633 w1646 w1659 w1673 w1687 w1692 w1704 w1716 w1729 w1742 w1758 w1786 w1801 w1806 w1815 w1853 w1866 w1874 w1882 w1896 w1901 w1907 w1924 w1941 w1958 w1978 w2003 w2011 w2016 w2024 w2032 w2037 w2046 w2085 w2125 w2140 w2153 w2166 w2184 w2190 w2201 w2214 w2232 w2239 w2251 w2316 w2327 w2340 w2365 w2388 w2394 w2400 w2415 w2460 w2468 w2474 w2479 w2485 w2493 w2502 w2512 w2518 w2524 w2529 w2535 w2548 w2582 w2591 w2603 w2629 w2655 w2677 w2683 w2708 w2733 w2758 w2783 w2800 w2863 w2921 w2940 w2950 w2973 w2978 w3000 w3009 w3018 w3023] -> w110
      tunnel: [_ _ _ _ _ _ _ _ _ _ _ _ _ _ _ _ _ _ _ _ _ _ _ _ _ TRUE _ _ _ _ _ _ _ _ _ _ _ _ _ _ _ _ _ _ _ _ _ _ _ _ _ _ _ _ _ _ _ _ _ _ _ _ _ _ _ _ _ _ _ _ _ _ _ _ _ _ _ _ _ _ _ _ _ _ _ _ _ _ _ _ _ _ _ _ _ _ _ _ _ _ _ _ _ _ _ _ _ _ _ _ _ _ _ _ _ _ _ _ _ _ _ _ _ _ _ _ _ _ _ _ _ _ _ _ _ _ _ _ _ _ _ _ _ _ _ _ _ _ _] -> w101
      tunnel: [w121 w458 w466 w473 w479 w486 w500 w510 w521 w549 w559 w586 w608 w626 w649 w656 w692 w721 w766 w792 w819 w827 w834 w843 w866 w891 w895 w901 w911 w921 w937 w956 w976 w986 w996 w1021 w1035 w1058 w1083 w1135 w1186 w1208 w1237 w1269 w1302 w1341 w1367 w1370 w1387 w1394 w1405 w1418 w1454 w1470 w1488 w1507 w1540 w1545 w1550 w1561 w1579 w1612 w1636 w1649 w1663 w1676 w1690 w1702 w1714 w1723 w1737 w1754 w1775 w1790 w1804 w1812 w1852 w1864 w1872 w1881 w1895 w1899 w1906 w1910 w1927 w1945 w1961 w1986 w2009 w2014 w2019 w2027 w2035 w2044 w2081 w2107 w2138 w2151 w2165 w2182 w2188 w2196 w2208 w2229 w2238 w2245 w2314 w2319 w2334 w2359 w2386 w2392 w2398 w2403 w2448 w2466 w2472 w2477 w2483 w2491 w2500 w2510 w2516 w2522 w2527 w2533 w2547 w2581 w2589 w2602 w2616 w2643 w2676 w2681 w2706 w2732 w2757 w2782 w2795 w2858 w2920 w2938 w2949 w2966 w2976 w2980 w3007 w3017 w3021] -> w109
      tunnel: 30 ("Timeout") -> [w120 _ _ _ _ _ _ _ _ _ _ _ _ _ _ _ _ _ _ _ _ _ _ _ _ _ _ _ _ _ _ _ _ _ _ _ _ _ _ _ _ _ _ _ _ _ _ _ _ _ _ _ _ _ _ _ _ _ _ _ _ _ _ _ _ _ _ _ _ _ _ _ _ _ _ _ _ _ _ _ _ _ _ _ _ _ _ _ _ _ _ _ _ _ _ _ _ _ _ _ _ _ _ _ _ _ _ _ _ _ _ _ _ _ _ _ _ _ _ _ _ _ _ _ _ _ _ _ _ _ _ _ _ _ _ _ _ _ _ _ _ _ _ _ _ _ _ _ _]
      tunnel: w106 -> [w114 _ _ _ _ _ _ _ _ _ _ _ _ w623 _ _ _ _ w774 _ _ _ _ _ _ _ _ _ _ _ _ _ _ _ _ _ _ _ _ _ _ _ _ _ _ _ _ _ _ _ _ _ _ _ _ _ _ _ _ _ _ _ _ _ _ _ _ _ _ _ _ _ _ _ _ _ w1848 _ _ _ w1891 _ _ _ _ _ _ _ _ _ _ _ _ _ _ _ _ _ _ _ _ _ _ _ _ _ _ _ _ _ _ _ _ _ _ _ _ _ _ _ _ _ _ _ _ _ _ _ _ _ _ _ _ _ _ _ _ _ _ w2861 _ _ _ _ _ _ _ _ _]
      tunnel: w105 -> [_ _ _ _ _ _ _ _ _ _ _ _ w611 w632 _ _ _ w724 w780 _ _ _ _ _ _ _ _ _ _ _ _ _ _ _ _ _ _ _ _ _ _ _ _ _ _ _ _ _ _ _ _ _ _ _ _ _ _ _ _ _ _ _ _ _ _ _ _ _ _ _ _ _ _ _ _ _ _ w1859 _ w1879 w1890 _ _ _ _ _ _ _ _ _ _ _ _ _ _ _ _ _ _ _ _ _ _ _ _ _ _ _ _ _ _ _ _ _ _ _ _ _ _ _ _ _ _ _ _ _ _ _ _ _ _ _ _ _ _ _ _ _ _ _ _ _ _ _ _ _ _ _ _]
      tunnel: w104 -> [w119 _ _ _ _ _ _ _ _ _ _ _ _ _ _ _ _ _ _ _ _ _ _ _ _ _ _ _ _ _ _ _ _ _ _ _ _ _ _ _ _ _ _ _ w1299 _ _ _ _ _ _ _ _ _ _ _ _ _ _ _ _ _ _ _ _ _ _ _ _ _ _ _ _ _ _ _ _ _ _ _ _ _ _ _ _ _ _ _ _ _ _ _ _ _ _ _ _ _ _ _ _ _ _ _ _ _ _ _ _ _ _ _ _ _ _ _ _ _ _ _ _ _ _ _ _ _ _ _ _ _ _ _ _ _ _ _ _ _ _ _ _ _ _ _ _ _ _ _ _]
      tunnel: w103 -> [w118 w457 w467 w472 w480 w489 w499 w509 w530 w548 w569 w585 w612 w633 w648 w662 w691 w726 w781 w816 w821 w826 w831 w848 w865 w889 w894 w902 w914 w926 w939 w958 w982 w985 w995 w1014 w1042 w1065 w1090 w1142 w1192 w1215 w1241 w1273 w1303 w1352 w1366 w1372 w1386 w1399 w1410 w1426 w1464 w1481 w1489 w1529 w1532 w1544 w1553 w1562 w1580 w1613 w1637 w1650 w1667 w1678 w1689 w1703 w1715 w1728 w1741 w1757 w1785 w1791 w1803 w1814 w1851 w1863 w1871 w1880 w1889 w1898 w1905 w1912 w1929 w1948 w1964 w1990 w2010 w2013 w2021 w2029 w2034 w2043 w2083 w2123 w2137 w2150 w2163 w2181 w2187 w2199 w2211 w2230 w2234 w2246 w2313 w2326 w2338 w2362 w2382 w2390 w2396 w2410 w2459 w2464 w2470 w2476 w2482 w2490 w2499 w2509 w2515 w2521 w2526 w2532 w2546 w2580 w2588 w2601 w2628 w2654 w2675 w2680 w2707 w2731 w2756 w2781 w2799 w2862 w2919 w2937 w2948 w2972 w2975 w2999 w3006 w3016 w3020]
      tunnel: [w116 w457 w467 w472 w480 w489 w499 w509 w530 w548 w569 w585 w612 w633 w648 w662 w691 w726 w781 w816 w821 w826 w831 w848 w865 w889 w894 w902 w914 w926 w939 w958 w982 w985 w995 w1014 w1042 w1065 w1090 w1142 w1192 w1215 w1241 w1273 w1303 w1352 w1366 w1372 w1386 w1399 w1410 w1426 w1464 w1481 w1489 w1529 w1532 w1544 w1553 w1562 w1580 w1613 w1637 w1650 w1667 w1678 w1689 w1703 w1715 w1728 w1741 w1757 w1785 w1791 w1803 w1814 w1851 w1863 w1871 w1880 w1889 w1898 w1905 w1912 w1929 w1948 w1964 w1990 w2010 w2013 w2021 w2029 w2034 w2043 w2083 w2123 w2137 w2150 w2163 w2181 w2187 w2199 w2211 w2230 w2234 w2246 w2313 w2326 w2338 w2362 w2382 w2390 w2396 w2410 w2459 w2464 w2470 w2476 w2482 w2490 w2499 w2509 w2515 w2521 w2526 w2532 w2546 w2580 w2588 w2601 w2628 w2654 w2675 w2680 w2707 w2731 w2756 w2781 w2799 w2862 w2919 w2937 w2948 w2972 w2975 w2999 w3006 w3016 w3020] -> w102
      tunnel: w100 -> [_ _ _ _ _ _ _ _ _ _ _ _ _ _ _ _ _ _ _ _ _ _ _ _ _ _ _ _ _ _ _ _ _ _ _ _ _ _ _ _ _ _ _ _ _ _ _ _ _ _ _ _ _ _ _ _ _ _ _ _ _ _ _ _ _ _ _ _ _ _ _ _ _ _ _ _ _ _ _ _ w1888 _ _ _ _ _ _ _ _ _ _ _ _ _ _ _ _ _ _ _ _ _ _ _ _ _ _ _ _ _ _ _ _ _ _ _ _ _ _ _ _ _ _ _ _ _ _ _ _ _ _ _ _ _ _ _ _ _ _ _ _ _ _ _ _ _ _ _ _]
      tunnel: w95 -> [w117 _ _ _ _ _ _ _ _ _ _ _ _ _ _ _ _ _ _ _ _ _ _ _ _ _ _ _ _ _ _ _ _ _ _ _ _ _ _ _ _ _ _ _ _ _ _ _ _ _ _ _ _ _ _ _ _ _ _ _ _ _ _ _ _ _ _ _ _ _ _ _ _ _ _ w1813 w1850 _ _ _ _ _ _ _ _ _ _ _ _ _ _ _ _ _ _ _ _ _ _ _ _ _ _ _ _ _ _ _ _ _ _ _ _ _ _ _ _ _ _ _ _ _ _ _ _ _ _ _ _ _ _ _ _ _ _ _ _ _ _ _ _ _ w2946 _ _ _ _ _ _]
      tunnel: w94 -> [w115 _ _ _ _ _ _ _ _ _ _ _ w601 _ _ w660 _ w707 _ _ _ _ _ _ _ _ _ _ _ _ _ _ _ _ _ _ _ _ _ _ _ _ _ _ _ _ _ _ _ _ _ _ _ _ _ _ _ _ _ _ _ _ _ _ _ _ _ _ _ _ _ _ _ _ _ _ w1844 _ _ _ w1885 _ _ _ _ _ _ _ _ _ _ _ _ _ _ _ _ _ _ _ _ _ _ _ _ _ _ _ _ _ _ _ _ _ _ _ _ _ _ _ _ _ _ _ _ _ _ _ _ _ _ _ _ _ _ _ _ _ w2797 _ _ _ _ _ _ _ _ _ _]
      frame "", "Event Structure", "Idle" {
        # "executes when the state queue is empty"
        n52 = event shown="[26] \"AcquireGain\": Value Change" {
          selector: w118 -> [_ _ _ _ _ _ _ _ _ _ _ _ _ _ _ _ _ _ _ _ _ _ _ _ _ _ _ _ _ _ _ _ _ _ _ _]
          dyn-events: [_ _ _ _ _ _ _ _ _ _ _ _ _ _ _ _ _ _ _ _ _ _ _ _ _ _ _ _ _ _ _ _ _ _ _ _] -> w116
          timeout: w120 -> [_ _ _ _ _ _ _ _ _ _ _ _ _ _ _ _ _ _ _ _ _ _ _ _ _ _ _ _ _ _ _ _ _ _ _ _]
          tunnel: w126 -> [w142 w151 w160 w172 w180 w197 w210 w227 w234 w241 w254 w265 w270 w276 w292 w296 w300 w305 w309 w314 w327 w333 w338 w342 w346 w357 w364 w382 w399 w404 w411 w416 w424 w433 w447 w456]
          tunnel: [w143 w151 w159 w172 w179 w197 w209 w226 w234 w240 w254 w265 w269 w277 w291 w296 w301 w305 w310 w314 w328 w332 w338 w342 w345 w358 w363 w381 w399 w405 w410 w415 w424 w433 w447 w455] -> w125
          tunnel: w124 -> [w129 w149 w153 w174 w182 w196 w211 w225 w233 w237 w253 w264 w266 w278 w290 w294 w298 w303 w307 w312 w316 w334 w336 w340 w347 w356 w366 w383 w397 w406 w412 w417 w419 w428 w445 w453]
          tunnel: [w131 w150 w156 w175 w183 w195 w202 w224 w230 w243 w250 w260 w268 w271 w286 w295 w299 w304 w308 w313 w324 w335 w337 w341 w348 w359 w367 w384 w398 w401 w413 w418 w423 w426 w446 w454] -> w123
          tunnel: w122 -> [w131 w150 w161 w175 w183 w195 w203 w224 w231 w242 w249 w259 w268 w272 w287 w295 w299 w304 w308 w313 w326 w335 w337 w341 w348 w359 w367 w384 w398 w400 w413 w418 w423 w425 w446 w454]
          tunnel: [w129 w149 w153 w174 w182 w196 w211 w225 w233 w236 w253 w264 w266 w278 w290 w294 w298 w303 w307 w312 w315 w334 w336 w340 w347 w356 w366 w383 w397 w407 w412 w417 w419 w429 w445 w453] -> w121
          tunnel: w119 -> [_ _ _ _ _ _ _ _ _ _ _ _ _ _ _ _ _ _ _ _ _ _ _ _ _ _ _ _ _ _ _ _ _ _ _ _]
          tunnel: w117 -> [_ _ _ _ _ _ _ _ _ _ _ _ _ _ _ _ _ _ _ _ _ _ _ _ _ _ _ _ _ _ _ _ _ _ _ _]
          tunnel: w115 -> [_ _ _ _ _ _ _ _ _ _ _ _ _ _ _ _ _ _ _ _ _ _ _ _ _ _ _ _ _ _ _ _ _ w427 _ _]
          tunnel: w114 -> [_ _ _ _ _ _ _ _ _ _ _ _ _ _ _ _ _ _ _ _ _ _ _ _ _ _ _ _ _ w402 _ _ _ _ _ _]
          event Timeout {
            # "check system status every 2s"
            n53 = event-data() -> ()  [unwired: 1 in, 1 out]
            n54 = Unbundle By Name(w129) -> ("SlowTimer"=w127:u32, "FastTimer"=w128:u32)
            n55 = Tick Count (ms)() -> (millisecond timer value=w132:u32)
            n56 = Subtract(x=w132, y=w127) -> (x-y=w137:u32)
            n57 = Subtract(x=w132, y=w128) -> (x-y=w133:u32)
            n58 = Greater?(x=w137, y=u32 2000) -> (0:w138:bool)
            n59 = Greater?(x=w133, y=u32 500) -> (0:w135:bool)
            n60 = case shown="True" w138 {
              tunnel: ["" ("Empty String Constant") "SystemStatus: SlowSysStatusMacro" ("State(s) in Front (\"\")")] -> w139
              frame False {
              }
              frame True {
              }
            }
            n61 = case shown="True" w135 {
              tunnel: ["" ("Empty String Constant") "SystemStatus: FastSysStatusMacro" ("State(s) in Front (\"\")")] -> w134
              frame False {
              }
              frame True {
              }
            }
            n62 = call <vilib>:"Add State(s) to Queue__JKI_lib_State_Machine.vi"("State(s) in Front (\"\")"="LabJack: checkPedal\nData: SignInRange" ("State(s) in Front (\"\")"), "State(s) in (\"\")"=w139, "State(s) at Back (\"\")"=w134) -> ("States Out"=w130:string)  [unwired: 12 in]
            n63 = call <vilib>:"Add State(s) to Queue__JKI_lib_State_Machine.vi"("State(s) in Front (\"\")"=w130, "State(s) in (\"\")"=w142) -> ("States Out"=w143:string)  [unwired: 13 in]
          }
          event "355nm Laser toggle": Mouse Enter {
            n64 = event-data() -> ()  [unwired: 1 in, 4 out]
            n65 = local write "Help"("Toggle 355nm laser." ("Help")) -> ()
          }
          event "355nm Laser toggle": Value Change {
            n66 = event-data() -> ()  [unwired: 1 in, 6 out]
            n67 = case shown="True" "355nm Laser toggle" {
              tunnel: [0.0 ("Value") 1.0 ("Value")] -> w163
              frame False {
                n68 = property on="Laser Rep Rate" class="DigNum (strict)"("DisabledEnum"=T11."Enabled" ("Disabled")) -> ()  [unwired: 2 in, 2 out]
              }
              frame True {
                n69 = property on="Laser Rep Rate" class="DigNum (strict)"("DisabledEnum"=T11."Disabled and Grayed Out" ("Disabled")) -> ()  [unwired: 2 in, 2 out]
              }
            }
            n70 = Unbundle By Name(w153) -> ("LJ Pinout.355 PWM"=w152:string)
            n71 = call "LabJack_FGV.vi"("Operation(Read)"=enum16{"Write", "Read"}."Read" ("Operation"), "error in (no error)"=w161) -> ("error out"=w165:errorcluster, "Read data"=w166:i32)  [unwired: 8 in]
            n72 = Concatenate Strings(w152, "_EF_ENABLE" ("string")) -> (w162:string)
            n73 = call "LJM_eWriteName.vi"("Handle In"=w166, "Name"=w162, "Value"=w163, "error in"=w165) -> ("error out"=w157:errorcluster)  [unwired: 10 in, 1 out]
            n74 = call <vilib>:"Add State(s) to Queue__JKI_lib_State_Machine.vi"("State(s) in Front (\"\")"="/*355 Laser: CheckControllerStatus\n/*355 Laser: CheckPWMStatus" ("State(s) in Front (\"\")"), "State(s) in (\"\")"=w160) -> ("States Out"=w159:string)  [unwired: 13 in]
            n75 = call <userlib>:"Wait (ms)__ogtk.vi"("error in (no error)"=w157, "milliseconds to wait"=u32 50) -> ("error out"=w156:errorcluster)  [unwired: 8 in, 1 out]
          }
          event "Aiming beam toggle": Mouse Enter {
            n76 = event-data() -> ()  [unwired: 1 in, 4 out]
            n77 = local write "Help"("Toggle aiming beam laser." ("Help")) -> ()
          }
          event "Aiming beam toggle": Value Change {
            # "[Covers: REQ27]"
            n78 = event-data() -> ("NewVal"=w181:bool)  [unwired: 1 in, 5 out]
            n79 = local read "AB Rep Rate"() -> (w177:u16)
            n80 = Equal To 0?(x=w177) -> (x = 0?=w176:bool)
            n81 = case shown="False" w181 {
              tunnel: [w184 w191] -> w178
              tunnel: w176 -> [w187 w189]
              frame False {
                w188 = T11."Enabled" ("Disabled")
                n82 = Select(t="LabJack: AB_DC_Stop" ("State(s) in Front (\"\")"), s=w187, f="LabJack: AB_PWM_Stop" ("State(s) in Front (\"\")")) -> (s? t:f=w184:string)
                n83 = property on="Current" class="DigNum (strict)"("DisabledEnum"=w188) -> ()  [unwired: 2 in, 2 out]
                n84 = property on="AB Rep Rate" class="DigNum (strict)"("DisabledEnum"=w188) -> ()  [unwired: 2 in, 2 out]
              }
              frame True {
                w193 = T11."Disabled and Grayed Out" ("Disabled")
                n85 = Select(t="LabJack: AB_DC_Start" ("State(s) in Front (\"\")"), s=w189, f="LabJack: AB_PWM_Start" ("State(s) in Front (\"\")")) -> (s? t:f=w191:string)
                n86 = property on="AB Rep Rate" class="DigNum (strict)"("DisabledEnum"=w193) -> ()  [unwired: 2 in, 2 out]
                n87 = property on="Current" class="DigNum (strict)"("DisabledEnum"=w193) -> ()  [unwired: 2 in, 2 out]
              }
            }
            n88 = call <vilib>:"Add State(s) to Queue__JKI_lib_State_Machine.vi"("State(s) in Front (\"\")"=w178, "State(s) in (\"\")"=w180) -> ("States Out"=w179:string)  [unwired: 13 in]
          }
          event "Auto gain": Value Change {
            n89 = event-data() -> ("NewVal"=w194:bool)  [unwired: 1 in, 5 out]
            n90 = case shown="True" w194 {
              frame False {
                n91 = local read "Ctrl V"() -> (w198:dbl)
                n92 = call "V1FGV.vi"("action (write)"=enum16{"write", "read"}."write" ("action"), "V1 in"=w198) -> ()  [unwired: 8 in, 2 out]
                n93 = property on="Ctrl V" class="DigNum (strict)"("DisabledEnum"=T11."Enabled" ("Disabled")) -> ()  [unwired: 2 in, 2 out]
              }
              frame True {
                n94 = property on="Ctrl V" class="DigNum (strict)"("DisabledEnum"=T11."Disabled and Grayed Out" ("Disabled")) -> ()  [unwired: 2 in, 2 out]
              }
            }
          }
          event "Channel": Value Change {
            n95 = event-data() -> ("NewVal"=w207:enum32{"Ch1", "Ch2", "Ch3", "Ch4"})  [unwired: 1 in, 5 out]
            n96 = case shown="\"Ch4\"" w207 {
              tunnel: [w213 w215 w217 w218] -> w206
              frame "Ch1", Default {
                n97 = local read "Ch1 Max CtrlV"() -> (w213:dbl)
                n98 = local write "Tab Control"(T2."APD1" ("Tab Control")) -> ()
              }
              frame "Ch2" {
                n99 = local read "Ch2 Max CtrlV"() -> (w215:dbl)
                n100 = local write "Tab Control"(T2."APD2" ("Tab Control")) -> ()
              }
              frame "Ch3" {
                n101 = local read "Ch3 Max CtrlV"() -> (w217:dbl)
                n102 = local write "Tab Control"(T2."APD3" ("Tab Control")) -> ()
              }
              frame "Ch4" {
                n103 = local read "Ch4 Max CtrlV"() -> (w218:dbl)
                n104 = local write "Tab Control"(T2."APD4" ("Tab Control")) -> ()
              }
            }
            n105 = local write "Gain High"(w206) -> ()
            n106 = call "V1FGV.vi"("Error In"=w203, "action (write)"=enum16{"write", "read"}."write" ("action"), "V1 in"=0.0) -> ("Error Out"=w202:errorcluster)  [unwired: 7 in, 1 out]
            n107 = call <vilib>:"Add State(s) to Queue__JKI_lib_State_Machine.vi"("State(s) in Front (\"\")"="UI: Cursor Set >> Busy\nDigitizer: ConfigMacro\nUI: Cursor Set >> Idle" ("State(s) in Front (\"\")"), "State(s) in (\"\")"=w210) -> ("States Out"=w209:string)  [unwired: 13 in]
          }
          event "Task": Value Change {
            n108 = event-data() -> ("NewVal"=w223:enum32{"iRFAndGain", "Alignment"})  [unwired: 1 in, 5 out]
            n109 = case shown="\"iRFAndGain\", Default" w223 {
              tunnel: ["SysConfig: Load Digitizer Setting\nUI: Update" ("State(s) in Front (\"\")") "SysConfig: Load Digitizer Setting Gain\nUI: Update" ("State(s) in Front (\"\")")] -> w222
              frame "iRFAndGain", Default {
                # "load iRF setting"
              }
              frame "Alignment" {
                # "load gain setting"
              }
            }
            n110 = call <vilib>:"Add State(s) to Queue__JKI_lib_State_Machine.vi"("State(s) in Front (\"\")"=w222, "State(s) in (\"\")"="UI: Cursor Set >> Busy\nDigitizer: ConfigMacro\nUI: Cursor Set >> Idle" ("State(s) in Front (\"\")")) -> ("States Out"=w220:string)  [unwired: 13 in]
            n111 = call <vilib>:"Add State(s) to Queue__JKI_lib_State_Machine.vi"("State(s) in Front (\"\")"=w220, "State(s) in (\"\")"=w227) -> ("States Out"=w226:string)  [unwired: 13 in]
          }
          event "Waveform (no average)": Cursor Move {
            n112 = event-data() -> ()  [unwired: 1 in, 9 out]
            n113 = control-ref of="Waveform (no average)"() -> (w232:refnum<vi>)
            n114 = call "UpdateCurserIdx(SubVI).vi"("error in (no error)"=w231, "WaveformGraph in"=w232) -> ("error out"=w230:errorcluster)  [unwired: 9 in]
          }
          event "Current": Value Change {
            n115 = event-data() -> ()  [unwired: 1 in, 6 out]
            n116 = Unbundle By Name(w237) -> ("AB Cluster"=w238:T21)
            n117 = Bundle By Name(cluster=w238, "Default Current"="Current") -> (w235:T21)
            n118 = Bundle By Name(cluster=w237, "AB Cluster"=w235) -> (w236:T22)
            n119 = call "writeAimingBeamSetting.vi"("error in"=w242, "Aiming Beam Cluster"=w235) -> ("error out"=w243:errorcluster)  [unwired: 9 in]
            n120 = call <vilib>:"Add State(s) to Queue__JKI_lib_State_Machine.vi"("State(s) in Front (\"\")"="SysConfig: Load AB setting\nAimingBeam: Set Current" ("State(s) in Front (\"\")"), "State(s) in (\"\")"=w241) -> ("States Out"=w240:string)  [unwired: 13 in]
          }
          event "Ctrl V": Value Change; "Ctrl V": Key Down {
            n121 = event-data() -> ()  [unwired: 1 in, 4 out]
            n122 = local read "Channel"() -> (w251:enum32{"Ch1", "Ch2", "Ch3", "Ch4"})
            n123 = case shown="\"Ch4\"" w251 {
              tunnel: [enum16{"Ch1", "Ch2", "Ch3", "Ch4"}."Ch1" ("Channel") enum16{"Ch1", "Ch2", "Ch3", "Ch4"}."Ch2" ("Channel") enum16{"Ch1", "Ch2", "Ch3", "Ch4"}."Ch3" ("Channel") enum16{"Ch1", "Ch2", "Ch3", "Ch4"}."Ch4" ("Channel")] -> w245
              frame "Ch1", Default {
              }
              frame "Ch2" {
              }
              frame "Ch3" {
              }
              frame "Ch4" {
              }
            }
            n124 = call "CtrlVtoGain.vi"("error in (no error)"=w249, "CtrlV(V)"="Ctrl V", "Channel"=w245) -> ("error out"=w250:errorcluster, "Gain"=→"GainIndicator":dbl)  [unwired: 7 in]
            n125 = formula code="float32 y=0.05;\nif (x>0&&x<3.8)\ny=0.1;\nif (x>=3.8&&x<4.4)\ny=0.02;\nif (x>=4.4)\ny=0.01;"("x"="Ctrl V") -> ("y"=w246:sgl)
            n126 = call "V1FGV.vi"("action (write)"=enum16{"write", "read"}."write" ("action"), "V1 in"="Ctrl V") -> ()  [unwired: 8 in, 2 out]
            n127 = property on="Ctrl V" class="DigNum (strict)"("Increment"=w246) -> ()  [unwired: 2 in, 2 out]
          }
          event "Save PID": Value Change {
            n128 = event-data() -> ()  [unwired: 1 in, 6 out]
            n129 = local read "Ch1 PID gains"() -> (w263:T6)
            n130 = local read "Ch2 PID gains"() -> (w262:T6)
            n131 = local read "Ch3 PID gains"() -> (w261:T6)
            n132 = call "writePIDSetting.vi"("Error In"=w259, "Ch3 PID gains"=w261, "Ch2 PID gains"=w262, "Ch1 PID gains"=w263) -> ("Error Out"=w260:errorcluster)  [unwired: 7 in]
          }
          event "Quit": Value Change {
            # "Exit Button Value Change (pressed) Event\n(when pressed.  quite)"
            n133 = event-data() -> ()  [unwired: 1 in, 1 out]
            n134 = call <vilib>:"Add State(s) to Queue__JKI_lib_State_Machine.vi"("State(s) in Front (\"\")"="LED: Off\nMacro: Exit", "State(s) in (\"\")"=w270) -> ("States Out"=w269:string)  [unwired: 13 in]
          }
          event "Laser Rep Rate": Value Change {
            n135 = event-data() -> ()  [unwired: 1 in, 6 out]
            n136 = call "LJ_calculate_PWM_parameters.vi"("Error In"=w272, "Laser Rep Rate (Hz)"="Laser Rep Rate", "Laser"=enum16{"355nm", "AimingBeam"}."355nm") -> ("Error Out"=w271:errorcluster)  [unwired: 7 in, 1 out]
            n137 = call <vilib>:"Add State(s) to Queue__JKI_lib_State_Machine.vi"("State(s) in Front (\"\")"="SysConfig: Load 355 PWM\nLabJack: 355_PWM_Config" ("State(s) in Front (\"\")"), "State(s) in (\"\")"=w276) -> ("States Out"=w277:string)  [unwired: 13 in]
          }
          event "AB Rep Rate", "Duty Cycle (%)": Value Change {
            n138 = event-data() -> ()  [unwired: 1 in, 6 out]
            n139 = Unbundle By Name(w290) -> ("AB Cluster"=w289:T21)
            n140 = Bundle By Name(cluster=w289, "Frequency(Hz)"="AB Rep Rate") -> (w288:T21)
            n141 = call "writeAimingBeamSetting.vi"("error in"=w287, "Aiming Beam Cluster"=w288) -> ("error out"=w286:errorcluster)  [unwired: 9 in]
            n142 = Equal To 0?(x="AB Rep Rate") -> (x = 0?=w284:bool)
            n143 = Select(t="", s=w284, f="AimingBeam: ComputePWM\nSysConfig: Load AB PWM\nLabJack: AB_PWM_Config" ("State(s) in Front (\"\")")) -> (s? t:f=w280:string)
            n144 = call <vilib>:"Add State(s) to Queue__JKI_lib_State_Machine.vi"("State(s) in Front (\"\")"="SysConfig: Load AB setting" ("State(s) in Front (\"\")"), "State(s) in (\"\")"=w280) -> ("States Out"=w279:string)  [unwired: 13 in]
            n145 = call <vilib>:"Add State(s) to Queue__JKI_lib_State_Machine.vi"("State(s) in Front (\"\")"=w279, "State(s) in (\"\")"=w292) -> ("States Out"=w291:string)  [unwired: 13 in]
          }
          event "StartButton": Mouse Enter {
            n146 = event-data() -> ()  [unwired: 1 in, 4 out]
            n147 = local write "Help"("Press to start aquisition." ("Help")) -> ()
          }
          event "StartButton": Value Change {
            # "Initialize both digitizer aquisition and\n send user event to trigger aquisition loop"
            n148 = event-data() -> ()  [unwired: 1 in, 6 out]
            n149 = call <vilib>:"Add State(s) to Queue__JKI_lib_State_Machine.vi"("State(s) in Front (\"\")"="Macro: StartRun" ("State(s) in Front (\"\")"), "State(s) in (\"\")"=w300) -> ("States Out"=w301:string)  [unwired: 13 in]
          }
          event "StopButton": Mouse Enter {
            n150 = event-data() -> ()  [unwired: 1 in, 4 out]
            n151 = local write "Help"("Press to stop data aquisition." ("Help")) -> ()
          }
          event "StopButton": Value Change {
            n152 = event-data() -> ()  [unwired: 1 in, 6 out]
            n153 = call <vilib>:"Add State(s) to Queue__JKI_lib_State_Machine.vi"("State(s) in Front (\"\")"="Macro: StopRun" ("State(s) in Front (\"\")"), "State(s) in (\"\")"=w309) -> ("States Out"=w310:string)  [unwired: 13 in]
          }
          event "Sys Reconfig": Mouse Enter {
            n154 = event-data() -> ()  [unwired: 1 in, 4 out]
            n155 = local write "Help"("Click to reconfig digitizer settings." ("Help")) -> ()
          }
          event "Sys Reconfig": Value Change {
            # "everytime the user change data aquisition setting, need to reinitilize decon engine and realign iRF.\ncheck whether data length has changed, if changed, reinitialize Decon engine\nreset BG ready, need a new BG"
            # "update DAQ FGV"
            n156 = event-data() -> ()  [unwired: 1 in, 6 out]
            n157 = call "SystemConfigEditorV6.vi"("error in"=w326) -> ("error out"=w325:errorcluster, "FLImDAQ out"=w322:T4)  [unwired: 1 in]
            n158 = Unbundle By Name(w316) -> ("FLImDAQ.min record length"=w317:i32)
            n159 = Unbundle By Name(w322) -> ("min record length"=w323:i32)
            n160 = call "FLImDAQ_FGV.vi"("error in (no error)"=w325, "Operation (Read)"=enum16{"Write", "Read"}."Write" ("Operation"), "Write data"=w322) -> ("error out"=w324:errorcluster, "Read data"=w321:T4)  [unwired: 7 in]
            n161 = Equal?(x=w317, y=w323) -> (x = y?=w320:bool)
            n162 = case shown="False" w320 {
              tunnel: ["UI: Cursor Set >> Busy\nDigitizer: ConfigMacro\n/*UI: CaliAndiRFNotReady\n/*UI iRF not ready\nUI: Update\nUI: Cursor Set >> Idle" "UI: Cursor Set >> Busy\nDigitizer: ConfigCh3iRF\nUI: Update\nUI: Cursor Set >> Idle"] -> w319
              frame False {
              }
              frame True {
              }
            }
            n163 = Bundle By Name(cluster=w316, "FLImDAQ"=w321) -> (w315:T22)
            n164 = call <vilib>:"Add State(s) to Queue__JKI_lib_State_Machine.vi"("State(s) in Front (\"\")"=w319, "State(s) in (\"\")"=w327) -> ("States Out"=w328:string)  [unwired: 13 in]
          }
          event "Clear WF Chart History": Value Change {
            n165 = event-data() -> ()  [unwired: 1 in, 6 out]
            n166 = call <vilib>:"Add State(s) to Queue__JKI_lib_State_Machine.vi"("State(s) in Front (\"\")"="Graph: ClearHistory" ("State(s) in Front (\"\")"), "State(s) in (\"\")"=w333) -> ("States Out"=w332:string)  [unwired: 13 in]
          }
          event "System Hardware Connection Status", "StartButton", "StopButton", "355nm Laser toggle", "Aiming beam toggle", "Sys Reconfig": Mouse Leave {
            n167 = event-data() -> ()  [unwired: 1 in, 4 out]
            n168 = invoke on="Help" class="Str" method="Reinit To Default"() -> ()  [unwired: 3 in, 3 out]
          }
          event "System Hardware Connection Status.Digitizer": Mouse Enter {
            n169 = event-data() -> ()  [unwired: 1 in, 4 out]
            n170 = local write "Help"("Status of hardware connections. TCP/IP is optional." ("Help")) -> ()
          }
          event "TCP Connect": Value Change {
            n171 = event-data() -> ("NewVal"=w343:bool)  [unwired: 1 in, 5 out]
            n172 = case shown="False" w343 {
              tunnel: ["UI: Update" ("State(s) in Front (\"\")") "UI: Update" ("State(s) in Front (\"\")")] -> w344
              frame False {
              }
              frame True {
              }
            }
            n173 = call <vilib>:"Add State(s) to Queue__JKI_lib_State_Machine.vi"("State(s) in Front (\"\")"=w344, "State(s) in (\"\")"=w346) -> ("States Out"=w345:string)  [unwired: 13 in]
          }
          event User Event {
            # "if aquisition loop is error out. Stop digitizer, flash queue, update front panel indicator, stop both laser and parse and save data"
            n174 = event-data() -> ()  [unwired: 1 in, 5 out]
            n175 = case shown="True" FALSE {
              tunnel: ["" ("Empty String Constant") "Data: parseRunDataMacro" ("State(s) in Front (\"\")")] -> w354
              frame False {
                # "if flag is 0, do not save data"
              }
              frame True {
                # "if save data flag is true enqueue data"
              }
            }
            n176 = call <vilib>:"Add State(s) to Queue__JKI_lib_State_Machine.vi"("State(s) in Front (\"\")"="Digitizer: Abort\nLabJack: ZeroV" ("State(s) in Front (\"\")"), "State(s) in (\"\")"=w354, "State(s) at Back (\"\")"="LED: BreathOff\nMacro: SysReadyForAqui\nUI: Update" ("State(s) in Front (\"\")")) -> ("States Out"=w355:string)  [unwired: 12 in]
            n177 = call <vilib>:"Add State(s) to Queue__JKI_lib_State_Machine.vi"("State(s) in Front (\"\")"=w355, "State(s) in (\"\")"=w357) -> ("States Out"=w358:string)  [unwired: 13 in]
          }
          event "AcquireGain": Value Change {
            n178 = event-data() -> ()  [unwired: 1 in, 6 out]
            n179 = local read "GainSigInRange"() -> (w365:bool)
            n180 = case shown="True" w365 {
              tunnel: ["" ("State(s) in Front (\"\")") w370] -> w362
              frame False {
                n181 = One Button Dialog(message="Please make sure peak voltage is with in 0.3V to 1.4V and try again!") -> ()  [unwired: 1 in, 1 out]
              }
              frame True {
                n182 = local read "Laser Rep Rate"() -> (w374:u16)
                n183 = In Range and Coerce(upper limit=u16 500, x=w374, lower limit=u16 50) -> (In Range?=w371:bool)  [unwired: 1 out]
                n184 = case shown="True" w371 {
                  tunnel: ["" ("State(s) in Front (\"\")") "UI: Cursor Set >> Busy\nUtility: EnableGain? >> False\nUtility: setSaveFlag >> 0\nQueue: Flash\nUtility: setSaveFlag >> 1\nQueue: CheckNumOfWF\nData: parseSingleGainData\nUI: UpdateGainDataIndicators\nUtility: EnableGain? >> True\nUI: Cursor Set >> Idle\n" ("State(s) in Front (\"\")")] -> w370
                  frame False {
                    n185 = One Button Dialog(message="Please set 355nm laser rep rate between 20 and 250Hz ") -> ()  [unwired: 1 in, 1 out]
                  }
                  frame True {
                    n186 = local write "Num WF to acquire"(500) -> ()
                  }
                }
              }
            }
            n187 = call <vilib>:"Add State(s) to Queue__JKI_lib_State_Machine.vi"("State(s) in Front (\"\")"=w362, "State(s) in (\"\")"=w364) -> ("States Out"=w363:string)  [unwired: 13 in]
          }
          event "AcquireIRF": Value Change {
            n188 = event-data() -> ()  [unwired: 1 in, 6 out]
            n189 = local read "iRFSigInRange"() -> (w379:bool)
            n190 = case shown="True" w379 {
              tunnel: ["" ("State(s) in Front (\"\")") w387] -> w380
              frame False {
                n191 = One Button Dialog(message="Please make sure peak voltage is with in 0.5V to 1.4V and try again!") -> ()  [unwired: 1 in, 1 out]
              }
              frame True {
                n192 = local read "Laser Rep Rate"() -> (w391:u16)
                n193 = In Range and Coerce(upper limit=u16 500, x=w391, lower limit=u16 20) -> (In Range?=w388:bool)  [unwired: 1 out]
                n194 = case shown="True" w388 {
                  tunnel: ["" ("State(s) in Front (\"\")") "UI: Cursor Set >> Busy\nUtility: EnableGain? >> False\nUtility: setSaveFlag >> 0\nQueue: Flash\nUtility: setSaveFlag >> 1\nQueue: CheckNumOfWF\nData: parseIRFSingleIRFData\nUI: UpdateIRFDataTable\nUtility: EnableGain? >> True\nUI: Cursor Set >> Idle\n" ("State(s) in Front (\"\")")] -> w387
                  frame False {
                    n195 = One Button Dialog(message="Please set 355nm laser rep rate between 20 and 200Hz ") -> ()  [unwired: 1 in, 1 out]
                  }
                  frame True {
                    n196 = local write "Num WF to acquire"(500) -> ()
                  }
                }
              }
            }
            n197 = call <vilib>:"Add State(s) to Queue__JKI_lib_State_Machine.vi"("State(s) in Front (\"\")"=w380, "State(s) in (\"\")"=w382) -> ("States Out"=w381:string)  [unwired: 13 in]
          }
          event "Tab Control": Value Change {
            n198 = event-data() -> ()  [unwired: 1 in, 6 out]
            n199 = case shown="\"Data parsing\"" "Tab Control" {
              frame "APD1", Default {
              }
              frame "APD2" {
              }
              frame "APD3" {
              }
              frame "Debug" {
              }
              frame "IO Ststus" {
              }
              frame "LJ pinout" {
              }
              frame "Digitizer Info" {
              }
              frame "Data parsing" {
              }
              frame "Intensity Trace" {
              }
              frame "iRF Measureement" {
              }
              frame "Gain Measurement" {
              }
            }
          }
          event "ClearIRFData": Value Change {
            n200 = event-data() -> ()  [unwired: 1 in, 6 out]
            n201 = Bundle By Name(cluster=w406, "iRFIdx"=0) -> (w407:T22)
            n202 = Flush Queue(queue=w402, error in (no error)=w400) -> (error out=w401:errorcluster)  [unwired: 2 out]
            n203 = call <vilib>:"Add State(s) to Queue__JKI_lib_State_Machine.vi"("State(s) in Front (\"\")"="UI: InitIRFDataTable" ("State(s) in Front (\"\")"), "State(s) in (\"\")"=w404) -> ("States Out"=w405:string)  [unwired: 13 in]
          }
          event "SaveGainData": Value Change {
            n204 = event-data() -> ()  [unwired: 1 in, 6 out]
            n205 = call <vilib>:"Add State(s) to Queue__JKI_lib_State_Machine.vi"("State(s) in Front (\"\")"="UI: Cursor Set >> Busy\nAPD: LoadFromSerial\nAPD: writeGain\nFile: BackupOld\nAPD: SaveNew\nAPD: LoadFromSerialNoRawData\nUI: Cursor Set >> Idle" ("State(s) in Front (\"\")"), "State(s) in (\"\")"=w411) -> ("States Out"=w410:string)  [unwired: 13 in]
          }
          event "SaveiRFData": Value Change {
            n206 = event-data() -> ()  [unwired: 1 in, 6 out]
            n207 = call <vilib>:"Add State(s) to Queue__JKI_lib_State_Machine.vi"("State(s) in Front (\"\")"="UI: Cursor Set >> Busy\nAPD: LoadFromSerial\nAPD: writeiRF\nFile: BackupOld\nAPD: SaveNew\nAPD: LoadFromSerialNoRawData\nUI: Cursor Set >> Idle" ("State(s) in Front (\"\")"), "State(s) in (\"\")"=w416) -> ("States Out"=w415:string)  [unwired: 13 in]
          }
          event "SetIRFCtrlV": Value Change {
            # "set iRF V"
            n208 = event-data() -> ()  [unwired: 1 in, 6 out]
            n209 = local read "iRFCtrlV"() -> (w422:dbl[])
            n210 = Unbundle By Name(w419) -> ("iRFIdx"=w420:i32)
            n211 = Index Array(array=w422, index=w420) -> (element=w421:dbl)
            n212 = property on="Ctrl V" class="DigNum (strict)"("Val(Sgnl)"=w421) -> ()  [unwired: 2 in, 2 out]
          }
          event "ClearGainData": Value Change {
            w432 = dbl[] [] ("Gain")
            n213 = event-data() -> ()  [unwired: 1 in, 6 out]
            n214 = Flush Queue(queue=w427, error in (no error)=w425) -> (error out=w426:errorcluster)  [unwired: 2 out]
            n215 = local write "GainDataTable"(string[][] [] ("Table Control")) -> ()
            n216 = Bundle By Name(cluster=w428, "GainDataTemp"=T12 {"CtrlV"=-1.0, "PeakV"=0.0, "PeakV Std"=0.0, "IntFactor"=1.0, "IntCorrPeakV"=0.0}) -> (w429:T22)
            n217 = local write "Gain"(w432) -> ()
            n218 = local write "Ctrl V"(w432) -> ()
            n219 = local write "Intensity Factor"(w432) -> ()
            n220 = local write "AUC Std"(w432) -> ()
            n221 = local write "AUC"(w432) -> ()
            n222 = local write "Int Corr AUC"(w432) -> ()
          }
          event "ComputeGain": Value Change {
            # "Devide Int corrected Peak V by the 1st element"
            n223 = event-data() -> ()  [unwired: 1 in, 6 out]
            n224 = local read "Int Corr AUC"() -> (w444:dbl[])
            n225 = local read "Ctrl V"() -> (w436:dbl[])
            n226 = Reverse 1D Array(array=w444) -> (reversed array=w443:dbl[])
            n227 = Index Array(array=w443, index=0) -> (element=w441:dbl)
            n228 = local read "GainDataTable"() -> (w440:string[][])
            n229 = Divide(x=w444, y=w441) -> (x/y=w435:dbl[])
            "Gain" <- w435
            n230 = Bundle("Ctrl V"=w436, w435) -> (→"XY Graph":cluster{"Ctrl V":dbl[], dbl[]})  [unwired: 1 in]
            n231 = for {
              tunnel: w435 -> [w450] mode=indexing
              tunnel: [w448] -> w438 mode=indexing
              n232 = Number To Fractional String(number=w450, precision (6)=i16 3) -> (F-format string=w448:string)  [unwired: 2 in]
            }
            n233 = Insert Into Array(array=w440, index (col)=5 ("disabled index (col)"), new element=w438) -> (w437:string[][])  [unwired: 1 in]
            n234 = local write "GainDataTable"(w437) -> ()
          }
          event Panel Close? {
            # "Discard the event because we'll close the front panel ourselves in Macro: Exit"
            # "Close Panel button (pressed) Event\n(this executes Macro: Exit to terminate the VI)"
            n235 = event-data() -> ()  [unwired: 1 in, 1 out]
            n236 = event-data ("Event Filter Node")("Discard?"=TRUE) -> ()  [unwired: 1 in, 1 out]
            n237 = call <vilib>:"Add State(s) to Queue__JKI_lib_State_Machine.vi"("State(s) in Front (\"\")"="Macro: Exit", "State(s) in (\"\")"=w456) -> ("States Out"=w455:string)  [unwired: 13 in]
          }
        }
      }
      frame "---------- Macro ----------" {
        # "Do not put any code in this frame.\n(It is a separator no-op. You can make a copy of this frame to create a new Macro frame)"
        n238 = call <vilib>:"Add State(s) to Queue__JKI_lib_State_Machine.vi"("State(s) in (\"\")"=w461) -> ("States Out"=w460:string)  [unwired: 14 in]
      }
      frame "Macro: Initialize" {
        # "load Labjack setting 1st as it contaisn laser pin infortmation"
        # "start laser 1st, need 7.5s for laser to get ready"
        # "Initialization Macro\n(This is called once, when the VI starts)"
        n239 = call <vilib>:"Add State(s) to Queue__JKI_lib_State_Machine.vi"("State(s) in Front (\"\")"="UI: showDisclaimer\nUI: Cursor Set >> Busy\nGraph: AddCursors\nData: Initialize\nInitialize Core Data\nUI: Initialize\nUI: Front Panel State >> Open\nUI: Update\nAPD: Initialize\nMacro: LoadSysConfig\nLabJack: Open\nLabJack: SetDefaultSub\nLED: OpenVIRef\nLED: BreathOrange\nUI: Update\n355 Laser: CheckControllerStatus\n355 Laser: Laser enable\n355 Laser: Dewelling>>5000\n355 Laser: CheckControllerStatus\nUI: Update\nLabJack: 355_PWM_Config\nLabJack: AB_PWM_Config\nUI: Update", "State(s) in (\"\")"="Digitizer: Initialize\nDigitizer: ConfigMacro\nUI: Update\nAimingBeam: Initialize\nAimingBeam: Set Status>>Enable\nAimingBeam: Set Current\nUI: Update\nUI: Update\n355 Laser: Check Dewelling\nUtility: SetDefaultMaxV\nUI: InitIRFDataTable\nPID: loadPID\nUI: Cursor Set >> Idle\nLED: BreathOff\nMacro: SysReadyForAqui") -> ("States Out"=w462:string)  [unwired: 13 in]
        n240 = call <vilib>:"Add State(s) to Queue__JKI_lib_State_Machine.vi"("State(s) in Front (\"\")"=w462, "State(s) in (\"\")"=w470) -> ("States Out"=w469:string)  [unwired: 13 in]
        "Help" <- "Hover over controls to see help!" ("Help")
      }
      frame "Macro: LoadSysConfig" {
        # "System configuration Macro\n(Load configurations for different component of the system)"
        n241 = call <vilib>:"Add State(s) to Queue__JKI_lib_State_Machine.vi"("State(s) in Front (\"\")"="SysConfig: Load Digitizer Setting\nSysConfig: Load AB setting\nSysConfig: Load LJ Pinout\nSysConfig: Load 355 PWM\nSysConfig: Load APD Info", "State(s) in (\"\")"=w476) -> ("States Out"=w475:string)  [unwired: 13 in]
      }
      frame "Macro: StartRun" {
        # "start PWM before acquisition"
        # "Start Run Macro\n(Macro to start a aquisition run)"
        n242 = local read "Task"() -> (w478:enum32{"iRFAndGain", "Alignment"})
        n243 = case shown="\"iRFAndGain\", Default" w478 {
          tunnel: ["UI: Update\nLabJack: 355_PWM_Start\nLabJack: SetV\nDigitizer: Start\nUI: DuringAquisition\nLED: BreathGreen\nUI: Update" "UI: Update\nLabJack: SetV\nUtility: Dewelling >>250\nDigitizer: Start\nUI: DuringAquisition\nLED: BreathGreen\nUI: Update"] -> w477
          frame "iRFAndGain", Default {
          }
          frame "Alignment" {
          }
        }
        n244 = call <vilib>:"Add State(s) to Queue__JKI_lib_State_Machine.vi"("State(s) in Front (\"\")"=w477, "State(s) in (\"\")"=w483) -> ("States Out"=w482:string)  [unwired: 13 in]
      }
      frame "Macro: StopRun" {
        # "if system is running, send stop command, if not do nothing."
        # "stop aquisition\nupdate UI"
        # "Do not put any code in this frame.\n(It is a separator no-op. You can make a copy of this frame to create a new Macro frame)"
        n245 = Unbundle By Name(w486) -> ("SysRunning?"=w487:bool)
        n246 = case shown="True" w487 {
          tunnel: ["" ("Empty String Constant") w494] -> w488
          frame False {
          }
          frame True {
            n247 = local read "Task"() -> (w495:enum32{"iRFAndGain", "Alignment"})
            n248 = case shown="\"Alignment\"" w495 {
              tunnel: ["LabJack: 355_PWM_Stop" ("State(s) in Front (\"\")") "Digitizer: Abort" ("State(s) in Front (\"\")")] -> w494
              frame "iRFAndGain", Default {
                # "stop laser if taken iRF"
              }
              frame "Alignment" {
                # "do nothing if take gain"
              }
            }
          }
        }
        n249 = call <vilib>:"Add State(s) to Queue__JKI_lib_State_Machine.vi"("State(s) in Front (\"\")"=w488, "State(s) in (\"\")"=w492) -> ("States Out"=w491:string)  [unwired: 13 in]
      }
      frame "Macro: SysReadyForAqui" {
        # "System ready for aquisition macro.\n(Set UI and LED)"
        n250 = call <vilib>:"Add State(s) to Queue__JKI_lib_State_Machine.vi"("State(s) in Front (\"\")"="UI: ReadyForAquisition\nLED: Green" ("State(s) in Front (\"\")"), "State(s) in (\"\")"=w503) -> ("States Out"=w502:string)  [unwired: 13 in]
      }
      frame "Macro: AskOverWrite" {
        # "Ask user whther to over write existing APD data\n(It is a separator no-op. You can make a copy of this frame to create a new Data frame)"
        n251 = Two Button Dialog(message="Do you want to save new data? old file will be renamed as backup.", 2:"Save" ("T button name (\"OK\")")) -> (T button?=w506:bool)  [unwired: 1 in]
        n252 = case shown="True" w506 {
          tunnel: ["" ("Empty String Constant") "File: BackupOld\nAPD: SaveNew" ("State(s) in Front (\"\")")] -> w505
          frame False {
          }
          frame True {
            # "backup old file and save new file"
          }
        }
        n253 = call <vilib>:"Add State(s) to Queue__JKI_lib_State_Machine.vi"("State(s) in Front (\"\")"=w505, "State(s) in (\"\")"=w512) -> ("States Out"=w511:string)  [unwired: 13 in]
      }
      frame "Macro: Exit" {
        # "close LJ last"
        # "check whether hardware is initilized, if so close, if not do nothing"
        # "Exit Macro, close all hardware\n(This is called once, when the VI exits)"
        n254 = Unbundle By Name(w521) -> ("System Status.TCP/IP"=w520:bool, "System Status.Digitizer"=w519:bool, "System Status.Aiming Beam"=w518:bool, "System Status.355 Laser"=w517:bool, "System Status.Labjack"=w516:bool, "Core.Close Panel on Exit?"=w515:bool)
        n255 = case shown="True" w520 {
          tunnel: ["" ("Empty String Constant") ""] -> w528
          frame False {
          }
          frame True {
          }
        }
        n256 = case shown="True" w519 {
          tunnel: ["" ("Empty String Constant") "Digitizer: Close"] -> w529
          frame False {
          }
          frame True {
          }
        }
        n257 = case shown="True" w516 {
          tunnel: ["" ("Empty String Constant") "LabJack: SetDefaultAndClose"] -> w522
          frame False {
          }
          frame True {
          }
        }
        n258 = case shown="True" w518 {
          tunnel: ["" ("Empty String Constant") w543] -> w524
          frame False {
          }
          frame True {
            w543 = "AimingBeam: Set Status >> Disable\nAimingBeam: Close"  # AimingBeam: Set Status >> Disable AimingBeam: Close
          }
        }
        n259 = case shown="True" w517 {
          tunnel: ["" ("Empty String Constant") "355 Laser: Close\n355 Laser: CheckControllerStatus"] -> w523
          frame False {
          }
          frame True {
          }
        }
        n260 = Select(t="UI: Front Panel State >> Close", s=w515, f="" ("Empty String Constant")) -> (s? t:f=w525:string)
        n261 = call <vilib>:"Add State(s) to Queue__JKI_lib_State_Machine.vi"("State(s) in Front (\"\")"=w528, "State(s) in (\"\")"=w529, "State(s) at Back (\"\")"=w524) -> ("States Out"=w531:string)  [unwired: 12 in]
        n262 = call <vilib>:"Add State(s) to Queue__JKI_lib_State_Machine.vi"("State(s) in Front (\"\")"=w531, "State(s) in (\"\")"=w523, "State(s) at Back (\"\")"=w522) -> ("States Out"=w527:string)  [unwired: 12 in]
        n263 = call <vilib>:"Add State(s) to Queue__JKI_lib_State_Machine.vi"("State(s) in Front (\"\")"=w527, "State(s) in (\"\")"="UI: Update\nLED: CloseVIRef\nQueue: Destory\nData: Cleanup\nExit", "State(s) at Back (\"\")"=w525) -> ("States Out"=w532:string)  [unwired: 12 in]
        n264 = call <vilib>:"Add State(s) to Queue__JKI_lib_State_Machine.vi"("State(s) in Front (\"\")"=w532, "State(s) in (\"\")"=w537) -> ("States Out"=w536:string)  [unwired: 13 in]
      }
      frame "---------- Data ----------" {
        # "Template Separator\n(You can make a copy of, or modify, this frame)"
        n265 = call <vilib>:"Add State(s) to Queue__JKI_lib_State_Machine.vi"("State(s) in (\"\")"=w552) -> ("States Out"=w551:string)  [unwired: 14 in]
      }
      frame "Data: Initialize" {
        w555 = 0  # iRFIdx
        w557 = T23 {"CtrlV"=-1.0, "AUC"=0.0, "AUC Std"=0.0, "IntFactor"=1.0, "IntCorrAUC"=0.0}  # GainDataTemp
        w558 = dbl[][] []  # GainBGRaw
        w560 = FALSE  # LedViRefOpen
        w556 = T24 {"Ch1Serial"="", "Ch2Serial"="", "Ch3Serial"="", "Ch4Serial"=""}  # APDSerials
        w561 = cluster{"RunID":i8, "BG ID":i8, "Cali ID":i8} {"RunID"=1, "BG ID"=1, "Cali ID"=1}  # IDs
        w562 = refnum<vi> refnum  # LED vi reference
        w563 = path ""  # TempPath
        w564 = T25 {"DataPath"=path "", "BG Path"=path "", "iRFPath"=path "", "CaliPath"=path ""}  # Pathes
        w565 = u32 0  # FastTimer
        w566 = u32 0  # SlowTimer
        w567 = dbl[][] []  # iRFAllGain
        w570 = T1 {"Digitizer"=FALSE, "Labjack"=FALSE, "Aiming Beam"=FALSE, "355 Laser"=FALSE, "TCP/IP"=FALSE}  # System Status
        w554 = T26 {"DIO_EF_CLOCK1_DIVISOR"=16, "DIO_EF_CLOCK1_ROLL_VALUE"=25000, "DIO#_EF_INDEX"=0, "DIO#_EF_OPTIONS"=1, "DIO#_EF_CONFIG_A"=6250}  # AB PWM setting
        w571 = T3 {"Ch1 Bias"="TDA11", "Ch2 Bias"="DAC10", "Ch3 Bias"="DAC0", "Ch4 Bias"="DAC0", "355 PWM"="FIO0", "AimingBeam PWM"="FIO2", "Laser Ready"="FIO3", "Interlock"="FIO1", "Laser Start/Stop"="FIO1", "Red LED"="FIO1", "Green LED"="FIO1", "Foot Pedal"="DIO15"}  # LJ Pinout
        w572 = 0  # TCP attempt count
        w553 = u32 0  # Laser start tic
        w573 = refnum<k20>[] []  # niTClk sessions
        w574 = u32 0  # Last Trigger
        w575 = T26 {"DIO_EF_CLOCK1_DIVISOR"=16, "DIO_EF_CLOCK1_ROLL_VALUE"=25000, "DIO#_EF_INDEX"=0, "DIO#_EF_OPTIONS"=1, "DIO#_EF_CONFIG_A"=6250}  # 355 PWM setting
        w576 = T21 {"Aiming Beam COM Port"="COM3", "Min Current"=0.0, "Max Current"=63.0, "Default Current"=20.0, "Frequency(Hz)"=0}  # AB Cluster
        w577 = T27 {"resource name"="", "resource name 2"="", "Channel"=enum."Channel 0", "trigger source"="VAL_EXTERNAL", "trigger level"=0.5, "trigger delay"=1.35e-07, "min sample rate"=12500000000.0, "min record length"=2500, "vertical range"=1.0, "vertical offset"=-0.25, "Waveform to Avg"=2000}  # FLImDAQ
        w578 = FALSE  # SysRunning?
        w568 = path ""  # DefaultPath
        w579 = T28 {"Ch1Enable?"=FALSE, "Ch2Enable?"=FALSE, "Ch3Enable?"=FALSE, "Ch1AutoGain?"=FALSE, "Ch2AutoGain?"=FALSE, "Ch3AutoGain?"=FALSE, "AimingBeamEnable?"=FALSE}  # SysConfigCluster
        w580 = T29 {"Current VI Reference"=refnum, "Close Panel on Exit?"=FALSE}  # Core
        # "Initialize the shift-register data, here.\n(data names are defined by what you wire into the bundle function)"
        n266 = call <vilib>:"Add State(s) to Queue__JKI_lib_State_Machine.vi"("State(s) in (\"\")"=w583) -> ("States Out"=w582:string)  [unwired: 14 in]
        n267 = Bundle("Core"=w580, "SysConfigCluster"=w579, "System Status"=w570, "IDs"=w561, "DefaultPath"=w568, "Pathes"=w564, "FLImDAQ"=w577, "SysRunning?"=w578, "AB Cluster"=w576, "LJ Pinout"=w571, "355 PWM setting"=w575, "AB PWM setting"=w554, "Last Trigger"=w574, "niTClk sessions"=w573, "Laser start tic"=w553, "TCP attempt count"=w572, "iRFAllGain"=w567, "SlowTimer"=w566, "FastTimer"=w565, "TempPath"=w563, "LED vi reference"=w562, "APDSerials"=w556, "LedViRefOpen"=w560, "GainBGRaw"=w558, "GainDataTemp"=w557, "iRFIdx"=w555) -> (w559:T22)  [unwired: 1 in]
      }
      frame "Data: SignInRange" {
        # "Check Whether Signal is in Range.\n(It is a separator no-op. You can make a copy of this frame to create a new Data frame)"
        n268 = local read "Task"() -> (w584:enum32{"iRFAndGain", "Alignment"})
        n269 = case shown="\"iRFAndGain\", Default" w584 {
          frame "iRFAndGain", Default {
            n270 = local read "Tab Control"() -> (w592:T2)
            n271 = case shown="\"iRF Measureement\"" w592 {
              tunnel: 1.4 ("upper limit") -> [_ w594 w598]
              tunnel: 0.1 ("lower limit") -> [_ w593 w597]
              frame "APD1", Default {
              }
              frame "Gain Measurement" {
                n272 = local read "WF max value"() -> (w596:dbl)
                n273 = In Range and Coerce(upper limit=w594, x=w596, lower limit=w593) -> (In Range?=→"GainSigInRange":bool)  [unwired: 1 out]
              }
              frame "iRF Measureement" {
                n274 = local read "WF max value"() -> (w600:dbl)
                n275 = In Range and Coerce(upper limit=w598, x=w600, lower limit=w597) -> (In Range?=→"iRFSigInRange":bool)  [unwired: 1 out]
              }
            }
          }
          frame "Alignment" {
          }
        }
        n276 = call <vilib>:"Add State(s) to Queue__JKI_lib_State_Machine.vi"("State(s) in (\"\")"=w589) -> ("States Out"=w588:string)  [unwired: 14 in]
      }
      frame "Data: parseRunDataGain" {
        w603 = cluster{"CtrlV":dbl, "WFs":dbl[][]} {"CtrlV"=0.0, "WFs"=[]}  # GainAllCluster
        # "data individual gian"
        # "Flash data from queue and save it in structure\n()"
        n277 = Flush Queue(queue=w611, error in (no error)=w609) -> (remaining elements=w610:cluster{"WF":dbl[][]}[], error out=w605:errorcluster)  [unwired: 1 out]
        n278 = for {
          tunnel: w610 -> [w616] mode=indexing
          tunnel: [w615] -> w602 mode=concatenating
          n279 = Unbundle By Name(w616) -> ("WF"=w615:dbl[][])
        }
        n280 = local read "Ctrl V"() -> (w607:dbl)
        n281 = Bundle By Name(cluster=w603, "CtrlV"=w607, "WFs"=w602) -> (w606:cluster{"CtrlV":dbl, "WFs":dbl[][]})
        n282 = Enqueue Element(queue=w601, element=w606, error in (no error)=w605) -> (error out=w604:errorcluster)  [unwired: 1 in, 2 out]
        n283 = call <vilib>:"Add State(s) to Queue__JKI_lib_State_Machine.vi"("State(s) in (\"\")"=w614) -> ("States Out"=w613:string)  [unwired: 14 in]
      }
      frame "Data: parseRunDataiRF" {
        w618 = T8 {"CtrlV"=0.0, "WFs"=[], "WFavg"=[]}  # DataAllCluster
        # "add remove dc and normalize"
        # "update graph"
        # "data individual gian"
        # "Flash data from queue and save it in structure\n()"
        n284 = Flush Queue(queue=w632, error in (no error)=w630) -> (remaining elements=w631:cluster{"WF":dbl[][]}[], error out=w621:errorcluster)  [unwired: 1 out]
        n285 = for {
          tunnel: w631 -> [w642] mode=indexing
          tunnel: [w641] -> w625 mode=concatenating
          n286 = Unbundle By Name(w642) -> ("WF"=w641:dbl[][])
        }
        n287 = Array Size(array=w625) -> (size(s)=→"data Size":i32[])
        n288 = Transpose 2D Array(2D array=w625) -> (transposed array=w628:dbl[][])
        n289 = for {
          tunnel: w628 -> [w640] mode=indexing
          tunnel: [w639] -> w619 mode=indexing
          n290 = call-poly <vilib>:"Mean.vi"("X"=w640) -> ("mean"=w639:dbl)  [unwired: 1 out]
        }
        n291 = local read "Ctrl V"() -> (w624:dbl)
        n292 = local read "Channel"() -> (w617:enum32{"Ch1", "Ch2", "Ch3", "Ch4"})
        n293 = Bundle By Name(cluster=w618, "CtrlV"=w624, "WFs"=w625, "WFavg"=w619) -> (w622:T8)
        n294 = Build Array(w619) -> (w627:dbl[][])
        n295 = Enqueue Element(queue=w623, element=w622, error in (no error)=w621) -> (error out=w620:errorcluster)  [unwired: 1 in, 2 out]
        n296 = case shown="\"Ch3\"" w617 {
          tunnel: w627 -> [w636 w637 w638]
          frame "Ch1", Default {
            n297 = local write "Ch1 iRF Graph"(w636) -> ()
          }
          frame "Ch2" {
            n298 = local write "Ch2 iRF Graph"(w637) -> ()
          }
          frame "Ch3" {
            n299 = local write "Ch3 iRF Graph"(w638) -> ()
          }
        }
        n300 = call <vilib>:"Add State(s) to Queue__JKI_lib_State_Machine.vi"("State(s) in (\"\")"=w635) -> ("States Out"=w634:string)  [unwired: 14 in]
      }
      frame "Data: parseRunDataMacro" {
        # "Sometimes it takes some time to parse run data"
        # "Parse data macro.\n(Set curse busy, parse data, then set cursor idle)"
        n301 = local read "Task"() -> (w647:enum32{"iRFAndGain", "Alignment"})
        n302 = case shown="\"Alignment\"" w647 {
          tunnel: ["Data: parseRunDataiRF" ("State(s) in Front (\"\")") "Data: parseRunDataGain" ("State(s) in Front (\"\")")] -> w646
          frame "iRFAndGain", Default {
          }
          frame "Alignment" {
          }
        }
        n303 = call <vilib>:"Add State(s) to Queue__JKI_lib_State_Machine.vi"("State(s) in Front (\"\")"="UI: Cursor Set >> Busy" ("State(s) in Front (\"\")"), "State(s) in (\"\")"=w646, "State(s) at Back (\"\")"="UI: Cursor Set>>Idle" ("State(s) in Front (\"\")")) -> ("States Out"=w645:string)  [unwired: 12 in]
        n304 = call <vilib>:"Add State(s) to Queue__JKI_lib_State_Machine.vi"("State(s) in Front (\"\")"=w645, "State(s) in (\"\")"=w652) -> ("States Out"=w651:string)  [unwired: 13 in]
      }
      frame "Data: parseGainBGAllGain" {
        # "Parse all data for all gain\n(parse data all gain)"
        n305 = Unbundle By Name(w655) -> ("SysRunning?"=w658:bool)
        n306 = case shown="False" w658 {
          tunnel: w661 -> [w675 w687]
          tunnel: w660 -> [w674 _]
          tunnel: [w670 w687] -> w659
          tunnel: ["" ("State(s) in Front (\"\")") "Idle\nData: parseGainBGAllGain" ("State(s) in Front (\"\")")] -> w657
          tunnel: w655 -> [w672 w686]
          tunnel: [w669 w686] -> w656
          frame False {
            # "save gain BG to temp"
            n307 = Flush Queue(queue=w674, error in (no error)=w675) -> (remaining elements=w676:cluster{"CtrlV":dbl, "WFs":dbl[][]}[], error out=w670:errorcluster)  [unwired: 1 out]
            n308 = for {
              tunnel: w676 -> [w684] mode=indexing
              tunnel: [w681] -> w671 mode=indexing
              tunnel: [w682] -> w668 mode=indexing
              tunnel: [w680] -> w667 mode=indexing
              n309 = Unbundle By Name(w684) -> ("CtrlV"=w682:dbl, "WFs"=w683:dbl[][])
              n310 = for {
                tunnel: w683 -> [w685] mode=indexing
                tunnel: [w685] -> w681 mode=concatenating
              }
              n311 = call-poly <vilib>:"Mean.vi"("X"=w681) -> ("mean"=w680:dbl)  [unwired: 1 out]
            }
            n312 = local read "Channel"() -> (w666:enum32{"Ch1", "Ch2", "Ch3", "Ch4"})
            n313 = Bundle(w668, w667) -> (w665:cluster{dbl[], dbl[]})  [unwired: 1 in]
            n314 = case shown="\"Ch3\"" w666 {
              tunnel: w665 -> [w677 w678 w679]
              frame "Ch1", Default {
                n315 = local write "Ch1 Gain"(w677) -> ()
              }
              frame "Ch2" {
                n316 = local write "Ch2 Gain"(w678) -> ()
              }
              frame "Ch3" {
                n317 = local write "Ch3 Gain"(w679) -> ()
              }
            }
            n318 = Bundle By Name(cluster=w672, "GainBGRaw"=w671) -> (w669:T22)
          }
          frame True {
            # "repeat if system is running"
          }
        }
        n319 = call <vilib>:"Add State(s) to Queue__JKI_lib_State_Machine.vi"("State(s) in Front (\"\")"=w657, "State(s) in (\"\")"=w664) -> ("States Out"=w663:string)  [unwired: 13 in]
      }
      frame "Data: parseDataAllGainMacro" {
        # "Do not put any code in this frame.\n(It is a separator no-op. You can make a copy of this frame to create a new Data frame)"
        n320 = local read "Task"() -> (w690:enum32{"iRFAndGain", "Alignment"})
        n321 = case shown="\"Alignment\"" w690 {
          tunnel: ["APD: writeiRF" ("State(s) in Front (\"\")") w698] -> w689
          frame "iRFAndGain", Default {
          }
          frame "Alignment" {
            n322 = case shown="True" "BG flag?" {
              tunnel: ["APD: writeGain" ("State(s) in Front (\"\")") "Data: parseGainBGAllGain" ("State(s) in Front (\"\")")] -> w698
              frame False {
              }
              frame True {
              }
            }
          }
        }
        n323 = call <vilib>:"Add State(s) to Queue__JKI_lib_State_Machine.vi"("State(s) in Front (\"\")"=w689, "State(s) in (\"\")"=w695) -> ("States Out"=w694:string)  [unwired: 13 in]
      }
      frame "Data: parseSingleGainData" {
        # "Parse gain data for a single gain.\n(Flush data from queue, calculate peak V and std)"
        n324 = Flush Queue(queue=w724, error in (no error)=w702) -> (remaining elements=w725:cluster{"WF":dbl[][]}[], error out=w704:errorcluster)  [unwired: 1 out]
        n325 = for {
          tunnel: w725 -> [w739] mode=indexing
          tunnel: [w738] -> w723 mode=concatenating
          tunnel: [w737] -> w709 mode=concatenating
          tunnel: [w736] -> w701 mode=concatenating
          n326 = Unbundle By Name(w739) -> ("WF"=w736:dbl[][])
          n327 = for {
            tunnel: w736 -> [w742] mode=indexing
            tunnel: [w741] -> w738 mode=indexing
            tunnel: [w740] -> w737 mode=indexing
            n328 = disable-structure shown="Enabled" {
              disable-tunnel: w742 -> [w745 w751]
              disable-tunnel: [w750 w763] -> w741
              disable-tunnel: [_ w752] -> w740
              frame Disabled {
                n329 = global read "GlobalVariables.vi" "DC Idx1"() -> (w748:i32)
                n330 = global read "GlobalVariables.vi" "DC Idx2"() -> (w749:i32)
                n331 = Subtract(x=w749, y=w748) -> (x-y=w747:i32)
                n332 = Array Subset(array=w745, index=w748, length=w747) -> (w746:dbl[])
                n333 = call-poly <vilib>:"Mean.vi"("X"=w746) -> ("mean"=w744:dbl)  [unwired: 1 out]
                n334 = Subtract(x=w745, y=w744) -> (x-y=w743:dbl[])
                n335 = Array Max & Min(array=w743) -> (max value=w750:dbl)  [unwired: 3 out]
              }
              frame Enabled {
                # "Compute AUC"
                # "DC remove"
                n336 = global read "GlobalVariables.vi" "DC Idx1"() -> (w758:i32)
                n337 = global read "GlobalVariables.vi" "DC Idx2"() -> (w760:i32)
                n338 = Subtract(x=w760, y=w758) -> (x-y=w759:i32)
                n339 = Array Subset(array=w751, index=w758, length=w759) -> (w757:dbl[])
                n340 = call-poly <vilib>:"Mean.vi"("X"=w757) -> ("mean"=w756:dbl)  [unwired: 1 out]
                n341 = Subtract(x=w751, y=w756) -> (x-y=w755:dbl[])
                n342 = global read "GlobalVariables.vi" "BG Idx2"() -> (w762:i32)
                n343 = global read "GlobalVariables.vi" "BG Idx1"() -> (w761:i32)
                n344 = Subtract(x=w762, y=w761) -> (x-y=w754:i32)
                n345 = Array Subset(array=w755, index=w761, length=w754) -> (w753:dbl[])
                n346 = Array Max & Min(array=w751) -> (max value=w752:dbl)  [unwired: 3 out]
                n347 = Add Array Elements(numeric array=w753) -> (sum=w763:dbl)
              }
            }
          }
        }
        n348 = call "V1FGV.vi"("action (write)"=enum16{"write", "read"}."read") -> ("V1 out"=w706:dbl)  [unwired: 9 in, 1 out]
        n349 = Unbundle By Name(w722) -> ("GainDataTemp.IntFactor"=w712:dbl, "GainDataTemp.CtrlV"=w717:dbl, "GainDataTemp.AUC"=w714:dbl)
        n350 = Equal?(x=w706, y=w717) -> (x = y?=w716:bool)
        n351 = call <vilib>:"Std Deviation and Variance.vi"("X"=w723) -> ("mean"=w715:dbl, "standard deviation"=w719:dbl)  [unwired: 1 in, 1 out]
        n352 = call-poly <vilib>:"Mean.vi"("X"=w709) -> ("mean"=w708:dbl)  [unwired: 1 out]
        n353 = case shown="True" w716 {
          tunnel: w715 -> [_ w735]
          tunnel: w714 -> [_ w734]
          tunnel: [w730 w731] -> w713
          tunnel: w712 -> [w730 w733]
          frame False {
            # "if new Ctrl V, use old int factor"
          }
          frame True {
            # "if current CtrlV is the same as last, this is intensity change point, calculate intensity factor"
            n354 = Divide(x=w735, y=w734) -> (x/y=w732:dbl)
            n355 = Multiply(x=w733, y=w732) -> (x*y=w731:dbl)
          }
        }
        n356 = Greater?(x=w708, y=1.2) -> (0:w710:bool)
        n357 = Divide(x=w715, y=w713) -> (x/y=w718:dbl)
        n358 = Bundle By Name(cluster=w722, "GainDataTemp.CtrlV"=w706, "GainDataTemp.AUC"=w715, "GainDataTemp.AUC Std"=w719, "GainDataTemp.IntFactor"=w713, "GainDataTemp.IntCorrAUC"=w718) -> (w721:T22)
        n359 = case shown="True" w710 {
          frame False {
          }
          frame True {
            # "Inform user data near maximum"
            n360 = One Button Dialog(message="Data near threshold! Move target away and retake data at the same gain to record intensity change! ") -> ()  [unwired: 1 in, 1 out]
          }
        }
        n361 = Bundle("V1 out"=w706, "WF"=w701) -> (w705:cluster{"V1 out":dbl, "WF":dbl[][]})  [unwired: 1 in]
        n362 = Enqueue Element(queue=w707, element=w705, error in (no error)=w704) -> (error out=w703:errorcluster)  [unwired: 1 in, 2 out]
        n363 = call <vilib>:"Add State(s) to Queue__JKI_lib_State_Machine.vi"("State(s) in (\"\")"=w728) -> ("States Out"=w727:string)  [unwired: 14 in]
      }
      frame "Data: parseIRFSingleIRFData" {
        w773 = T8 {"CtrlV"=0.0, "WFs"=[], "WFavg"=[]}  # iRFDataAllCluster
        # "Parse iRF data from a single gain\n(It is a separator no-op. You can make a copy of this frame to create a new Data frame)"
        n364 = Flush Queue(queue=w780, error in (no error)=w770) -> (remaining elements=w779:cluster{"WF":dbl[][]}[], error out=w772:errorcluster)  [unwired: 1 out]
        n365 = for {
          tunnel: w779 -> [w787] mode=indexing
          tunnel: [w786] -> w775 mode=concatenating
          n366 = Unbundle By Name(w787) -> ("WF"=w786:dbl[][])
        }
        n367 = Transpose 2D Array(2D array=w775) -> (transposed array=w777:dbl[][])
        n368 = for {
          tunnel: w777 -> [w785] mode=indexing
          tunnel: [w784] -> w769 mode=indexing
          # "Average WF"
          n369 = call-poly <vilib>:"Mean.vi"("X"=w785) -> ("mean"=w784:dbl)  [unwired: 1 out]
        }
        "Current iRF" <- w769
        n370 = call "V1FGV.vi"("action (write)"=enum16{"write", "read"}."read") -> ("V1 out"=w776:dbl)  [unwired: 9 in, 1 out]
        n371 = Bundle By Name(cluster=w773, "CtrlV"=w776, "WFs"=w775, "WFavg"=w769) -> (w764:T8)
        n372 = Enqueue Element(queue=w774, element=w764, error in (no error)=w772) -> (error out=w771:errorcluster)  [unwired: 1 in, 2 out]
        n373 = Unbundle By Name(w765) -> ("iRFIdx"=w768:i32)
        n374 = Increment(x=w768) -> (x+1=w767:i32)
        n375 = Bundle By Name(cluster=w765, "iRFIdx"=w767) -> (w766:T22)
        n376 = call <vilib>:"Add State(s) to Queue__JKI_lib_State_Machine.vi"("State(s) in (\"\")"=w783) -> ("States Out"=w782:string)  [unwired: 14 in]
      }
      frame "Data: saveiRF" {
        w791 = enum16{"write", "read"}."read" ("action")
        # "Get iRF from decon stracture and save it on disk.\n(It is a separator no-op. You can make a copy of this frame to create a new Data frame)"
        n377 = Unbundle By Name(w792) -> ("TempPath"=w793:path)
        n378 = call "Ch1DeconEngineFGV.vi"("action(read)"=w791) -> ("Error Out"=w814:errorcluster, "Ch1DeconEngine out"=w815:refnum<class "LaguerreDeconEngineClass.lvclass">)  [unwired: 9 in]
        n379 = call "Ch2DeconEngineFGV.vi"("action(read)"=w791) -> ("Error Out"=w812:errorcluster, "Ch2DeconEngine out"=w813:refnum<class "LaguerreDeconEngineClass.lvclass">)  [unwired: 9 in]
        n380 = call "Ch3DeconEngineFGV.vi"("action(read)"=w791) -> ("Error Out"=w810:errorcluster, "Ch3DeconEngine out"=w811:refnum<class "LaguerreDeconEngineClass.lvclass">)  [unwired: 9 in]
        n381 = call "Ch4DeconEngineFGV.vi"("action(read)"=w791) -> ("Error Out"=w789:errorcluster, "Ch3DeconEngine out"=w790:refnum<class "LaguerreDeconEngineClass.lvclass">)  [unwired: 9 in]
        n382 = Build Path(base path=w793, name or relative path="iRF" ("default name")) -> (appended path=w808:path)
        n383 = call "getIRF.vi"("error in (no error)"=w789, "LaguerreDeconEngineClass in"=w790) -> ("iRF"=w788:dbl[])  [unwired: 7 in, 2 out]
        n384 = call "getIRF.vi"("error in (no error)"=w814, "LaguerreDeconEngineClass in"=w815) -> ("iRF"=w797:dbl[])  [unwired: 7 in, 2 out]
        n385 = call "getIRF.vi"("error in (no error)"=w812, "LaguerreDeconEngineClass in"=w813) -> ("iRF"=w796:dbl[])  [unwired: 7 in, 2 out]
        n386 = call "getIRF.vi"("error in (no error)"=w810, "LaguerreDeconEngineClass in"=w811) -> ("iRF"=w795:dbl[])  [unwired: 7 in, 2 out]
        n387 = TDMS Open(8:w807, 10:T13."create or replace" ("operation (0:open)"), 11:w808) -> (0:w804:errorcluster, 3:w805:refnum<k34>)  [unwired: 4 in]
        n388 = Build Array(w797, w796, w795, w788) -> (w803:dbl[][])
        n389 = Bundle("iRF"=w797, "iRF"=w796, "iRF"=w795, "iRF"=w788) -> (w794:T30)  [unwired: 1 in]
        n390 = global write "GlobalVariables.vi" "LastUseiRF"(w794) -> ()
        n391 = TDMS Write(0:w805, 5:"iRF" ("group name in (Untitled)"), 7:string[] ["Ch1", "Ch2", "Ch3", "Ch4"] ("channel name(s) in (Untitled)"), 9:w803, 11:w804) -> (4:w800:refnum<k34>, 15:w799:errorcluster)  [unwired: 1 in, 2 out]
        n392 = TDMS Close(8:w799, 11:w800) -> (0:w798:errorcluster)  [unwired: 1 out]
        n393 = call <vilib>:"Add State(s) to Queue__JKI_lib_State_Machine.vi"("State(s) in (\"\")"=w818) -> ("States Out"=w817:string)  [unwired: 14 in]
      }
      frame "Data: Cleanup" {
        # "Cleanup any data and references, here.\n(this is called automatically, by the Macro: Exit)"
        n394 = Unbundle By Name(w819) -> ("Core.Current VI Reference"=w820:refnum<vi>)
        n395 = Close Reference(reference=w820, error in (no error)=w823) -> (error out=w822:errorcluster)
        n396 = call <vilib>:"Add State(s) to Queue__JKI_lib_State_Machine.vi"("State(s) in (\"\")"=w825) -> ("States Out"=w824:string)  [unwired: 14 in]
      }
      frame "---------- Core ----------" {
        # "Do not put any code in this frame.\n(it is a separator no-op)"
        n397 = call <vilib>:"Add State(s) to Queue__JKI_lib_State_Machine.vi"("State(s) in (\"\")"=w830) -> ("States Out"=w829:string)  [unwired: 14 in]
      }
      frame Default {
        w841 = 42 items=["No error", "Argument error", "Memory is full", "Out of zone", "End of file", "File already open", "Generic file I/O error", "File not found", "File permission error", "Disk is full", "Duplicate path", "Too many files open", "System feature not enabled", "Resource file not found", "Cannot add resource", "Resource not found", "Image not found", "Image memory error", "Pen does not exist", "Config type invalid", "Config token not found", "Config parse error", "Config memory error", "Bad external code format", "Bad external code offset", "External code not present", "Null window", "Destroy window error", "Null menu", "Print aborted", "Bad print record", "Print driver error", "Windows error during printing", "Memory error during printing", "Print dialog error", "Generic print error", "Invalid device refnum", "Device not found", "Device parameter error", "Device unit error", "Cannot open device", "Device call aborted", "Generic error", "Cancelled by user", "Object ID too low", "Object ID too high", "Object not in heap", "Unknown heap", "Unknown object (invalid DefProc)", "Unknown object (DefProc not in table)", "Message out of range", "Invalid (null) method", "Unknown message", "Manager call not supported", "Bad address", "Network operation in progress", "Network operation timed out", "Connection is busy", "Network attribute not supported", "Network error", "Address in use", "System out of memory", "Connection aborted", "Connection refused", "Not connected", "Already connected", "Connection closed", "Initialization error (interapplication manager)", "Bad occurrence", "Wait on unbound occurrence handler", "Occurrence queue overflow", "Datalog type conflict", "Unused", "Unrecognized type (interapplication manager)", "Memory corrupt", "Failed to make temporary DLL", "Old CIN version", "Drag socket not found", "Failed to load drop-object", "Failed to register OLE object", "Failed to release OLE object", "Format specifier type mismatch", "Unknown format specifier", "Too few format specifiers", "Too many format specifiers", "Scan failed", "Newer CIN version", "Error converting to variant", "Runtime menu error", "Password tampered", "Variant attribute not found", "Incompatible variant data type", "Event data is not available", "Event Store is not present", "Occurrence is not found", "Event Queue is not created", "Event info is not available", "Refnum passed is NULL", "Error retrieving Class GUID", "Error retrieving CoClass GUID", "Error retrieving TypeLib GUID.", "Bad built application magic bytes.", "Specific driver is different from the specific driver associated with the Logical Name.", "There is no session opened to the class driver.", "Max Error", "MAX - Error with config objects", "MAX - Error loading configuration", "MAX - Group not supported"]
        # "Current State"
        # "Do not delete, rename, or modify this frame.\n(this is used to capture unhandled states and typos)"
        # "Handle mistyped state name (developer tool)"
        n398 = Format Into String(format string="Software Exception: Unhandled State \"%s\"." ("message"), error in=w837, w832) -> (resulting string=w840:string, error out=w839:errorcluster)  [unwired: 1 in]
        n399 = call <vilib>:"Error Cluster From Error Code.vi"("show call chain? (False)"=TRUE, "error in (no error)"=w839, "error message (\"\")"=w840, "error code (0)"=w841) -> ("error out"=w838:errorcluster)  [unwired: 5 in]
        n400 = call <vilib>:"Add State(s) to Queue__JKI_lib_State_Machine.vi"("State(s) in (\"\")"=w836) -> ("States Out"=w835:string)  [unwired: 14 in]
      }
      frame "Initialize Core Data" {
        # "Build default path based on the location of project"
        # "Do not delete, rename, or modify this frame.\n(this is used to determine panel behavior on exit)"
        # "originally closed?"
        # "exe?"
        # "If panel starts closed or is an EXE, then close it when we exit"
        n401 = call <vilib>:"Application Directory.vi"() -> ("Application Directory"=w845:path)
        n402 = property on="Property Node" class="App"() -> ("App.Kind"=w858:T15)  [unwired: 2 in, 2 out]
        n403 = property on="Property Node" class="VI"() -> ("FP.State"=w853:T14)  [unwired: 2 in, 2 out]
        n404 = control-ref of="Current VI Reference"() -> (w854:refnum<vi>)
        n405 = Equal?(x=w853, y=T14."Closed" ("Front Panel Window:State")) -> (x = y?=w851:bool)
        n406 = Equal?(x=w858, y=T15."Run Time System" ("Application:Kind")) -> (x = y?=w856:bool)
        n407 = Build Path(base path=w845, name or relative path="Data") -> (appended path=w849:path)
        n408 = Build Path(base path=w845, name or relative path="SystemTemp") -> (appended path=w846:path)
        n409 = Or(x=w851, y=w856) -> (x .or. y?=w855:bool)
        n410 = Bundle By Name(cluster=w844, "Core.Current VI Reference"=w854, "Core.Close Panel on Exit?"=w855, "DefaultPath"=w849, "TempPath"=w846) -> (w843:T22)
        n411 = call <vilib>:"Add State(s) to Queue__JKI_lib_State_Machine.vi"("State(s) in (\"\")"=w861) -> ("States Out"=w860:string)  [unwired: 14 in]
      }
      frame "Error Handler" {
        # "Unhandled Error -- Display it"
        # "Handle any errors here.\nYou can also output any states to clean-up after errors occur"
        # "Clear error"
        n412 = Unbundle By Name(w862) -> ("code"=w864:i32)
        n413 = case shown="5005" w864 {
          tunnel: ["Macro: Exit" w874 w880 ""] -> w863
          tunnel: w862 -> [w870 _ _ _]
          frame Default {
            w872 = T31 1 items=["no dialog", "OK message", "continue or stop message", "OK message + warnings", "continue/stop + warnings"] ("type of dialog (OK msg:1)")
            n414 = call <vilib>:"General Error Handler.vi"("type of dialog (OK msg:1)"=w872, "error in (no error)"=w870) -> ()  [unwired: 9 in, 5 out]
          }
          frame 5002 {
            n415 = Two Button Dialog(message="Laser interlock open! Please close interlock and try again! ", 1:"Safely Shutdown" ("F button name (\"Cancel\")"), 2:"OK" ("T button name (\"OK\")")) -> (T button?=w875:bool)
            n416 = case shown="True" w875 {
              tunnel: ["Macro: Exit" "355 Laser: CheckControllerStatus"] -> w874
              frame False {
              }
              frame True {
              }
            }
          }
          frame 5001 {
            n417 = Two Button Dialog(message="Unable to connect to imaging computer, do you want to run data aquisiton along? ", 1:"No" ("F button name (\"Cancel\")"), 2:"Yes" ("T button name (\"OK\")")) -> (T button?=w881:bool)
            n418 = case shown="True" w881 {
              tunnel: ["Macro: Exit" "" ("Empty String Constant")] -> w880
              frame False {
              }
              frame True {
              }
            }
          }
          frame 5005 {
          }
        }
        n419 = call <vilib>:"Add State(s) to Queue__JKI_lib_State_Machine.vi"("State(s) in Front (\"\")"=w863, "State(s) in (\"\")"=w869) -> ("States Out"=w868:string)  [unwired: 13 in]
      }
      frame "Exit" {
        # "Do not put any code in this frame.\n(No errors that occur here will be handled.)"
        n420 = call <vilib>:"Add State(s) to Queue__JKI_lib_State_Machine.vi"("State(s) in (\"\")"=w893) -> ("States Out"=w892:string)  [unwired: 14 in]
      }
      frame "---------- AimingBeam ----------" {
        # "Template Separator\n(You can make a copy of, or modify, this frame)"
        n421 = call <vilib>:"Add State(s) to Queue__JKI_lib_State_Machine.vi"("State(s) in (\"\")"=w898) -> ("States Out"=w897:string)  [unwired: 14 in]
      }
      frame "AimingBeam: Initialize" {
        # "set aiming beam button color"
        # "Open COM port for Aiming Beam\n(Require USB connection)"
        n422 = Unbundle By Name(w900) -> ("AB Cluster.Aiming Beam COM Port"=w899:refnum<visa-resource-name>)
        n423 = call-poly "VISA Configure Serial Port"("VISA resource name"=w899, "Enable Termination\nChar (T)"=TRUE ("Enable Termination\nChar (T)"), "baud rate (9600)"=u32 9600, "error in (no error)"=w906) -> ("error out"=w905:errorcluster)  [unwired: 10 in, 1 out]
        n424 = Unbundle By Name(w905) -> ("status"=w904:bool)
        n425 = Not(x=w904) -> (.not. x?=w903:bool)
        n426 = Bundle By Name(cluster=w900, "System Status.Aiming Beam"=w903) -> (w901:T22)
        n427 = call <vilib>:"Add State(s) to Queue__JKI_lib_State_Machine.vi"("State(s) in (\"\")"=w910) -> ("States Out"=w909:string)  [unwired: 14 in]
      }
      frame "AimingBeam: Close" {
        # "Close Aiming Beam COM port\n(Require USB connection to Aiming Beam Laser)"
        n428 = Unbundle By Name(w912) -> ("AB Cluster.Aiming Beam COM Port"=w913:refnum<visa-resource-name>)
        n429 = VISA Close(VISA resource name=w913, error in (no error)=w916) -> (error out=w917:errorcluster)
        n430 = Bundle By Name(cluster=w912, "System Status.Aiming Beam"=FALSE) -> (w911:T22)
        n431 = call <vilib>:"Add State(s) to Queue__JKI_lib_State_Machine.vi"("State(s) in (\"\")"=w919) -> ("States Out"=w918:string)  [unwired: 14 in]
      }
      frame "AimingBeam: Set Current" {
        # "Set Aiming Beam Current\n(You can make a copy of, or modify, this frame)"
        n432 = Unbundle By Name(w921) -> ("AB Cluster.Aiming Beam COM Port"=w920:refnum<visa-resource-name>, "AB Cluster.Max Current"=w925:dbl, "AB Cluster.Default Current"=w924:dbl, "AB Cluster.Min Current"=w923:dbl)
        n433 = In Range and Coerce(upper limit=w925, x=w924, lower limit=w923) -> (coerced(x)=w922:dbl)  [unwired: 1 out]
        n434 = local write "Current"(w922) -> ()
        n435 = Number To Fractional String(number=w922, precision (6)=i16 2) -> (F-format string=w929:string)  [unwired: 2 in]
        n436 = Concatenate Strings("slc:", w929, "\r" ("Carriage Return Constant"), "\n" ("Line Feed Constant")) -> (w932:string)
        n437 = VISA Write(VISA resource name=w920, write buffer=w932, error in (no error)=w927) -> (error out=w928:errorcluster)  [unwired: 2 out]
        n438 = call <vilib>:"Add State(s) to Queue__JKI_lib_State_Machine.vi"("State(s) in (\"\")"=w936) -> ("States Out"=w935:string)  [unwired: 14 in]
      }
      frame "AimingBeam: Set Status" {
        # "Enable Aiming Beam\n(Usage: \"AimingBeam: Set >> Enable|Disable\")"
        n439 = Unbundle By Name(w937) -> ("AB Cluster.Aiming Beam COM Port"=w938:refnum<visa-resource-name>)
        n440 = case shown="\"Enable\"" w943 {
          tunnel: [w945 w949] -> w942
          frame "Disable", Default {
            n441 = Concatenate Strings("cof", "\r" ("Carriage Return Constant"), "\n" ("Line Feed Constant")) -> (w945:string)
          }
          frame "Enable" {
            n442 = Concatenate Strings("con", "\r" ("Carriage Return Constant"), "\n" ("Line Feed Constant")) -> (w949:string)
          }
        }
        n443 = VISA Write(VISA resource name=w938, write buffer=w942, error in (no error)=w940) -> (error out=w941:errorcluster)  [unwired: 2 out]
      }
      frame "AimingBeam: GetPWMStatus" {
        # "Get aiming beam PWM status\n()"
        n444 = local read "AB Rep Rate"() -> (w954:u16)
        n445 = Greater Than 0?(x=w954) -> (x > 0?=w953:bool)
        n446 = case shown="True" w953 {
          tunnel: w957 -> [w961 w966]
          tunnel: w956 -> [_ w965]
          tunnel: [w961 w964] -> w955
          frame False {
          }
          frame True {
            n447 = Unbundle By Name(w965) -> ("LJ Pinout.AimingBeam PWM"=w962:string)
            n448 = call "LabJack_FGV.vi"("Operation(Read)"=enum16{"Write", "Read"}."Read" ("Operation"), "error in (no error)"=w966) -> ("error out"=w969:errorcluster, "Read data"=w970:i32)  [unwired: 8 in]
            n449 = Concatenate Strings(w962, "_EF_ENABLE" ("string")) -> (w968:string)
            n450 = call "LJM_eReadName.vi"("Handle In"=w970, "Name"=w968, "error in"=w969) -> ("Value"=w967:dbl, "error out"=w964:errorcluster)  [unwired: 10 in, 1 out]
            n451 = Greater Than 0?(x=w967) -> (x > 0?=w963:bool)
            n452 = case shown="True" w963 {
              frame False {
                # "PWM is off\nset color to gray"
                n453 = local write "Aiming beam toggle"(FALSE ("Aimging beam")) -> ()
              }
              frame True {
                # "PWM is on\nset color to light green"
                n454 = local write "Aiming beam toggle"(TRUE ("Aimging beam")) -> ()
              }
            }
          }
        }
        n455 = call <vilib>:"Add State(s) to Queue__JKI_lib_State_Machine.vi"("State(s) in (\"\")"=w960) -> ("States Out"=w959:string)  [unwired: 14 in]
      }
      frame "AimingBeam: ComputePWM" {
        # "Compute PWM parameter based on AB frequency\n(You can make a copy of, or modify, this frame)"
        n456 = Unbundle By Name(w976) -> ("AB Cluster.Frequency(Hz)"=w975:i32)
        n457 = call "LJ_calculate_PWM_parameters.vi"("Duty Cycle (%)"="Duty Cycle (%)", "Error In"=w977, "Show Confirmation"=FALSE, "Laser Rep Rate (Hz)"=w975, "Laser"=enum16{"355nm", "AimingBeam"}."AimingBeam") -> ("Error Out"=w978:errorcluster)  [unwired: 5 in, 1 out]
        n458 = call <vilib>:"Add State(s) to Queue__JKI_lib_State_Machine.vi"("State(s) in (\"\")"=w984) -> ("States Out"=w983:string)  [unwired: 14 in]
      }
      frame "---------- Digitizer ----------" {
        # "Template Separator\n(You can make a copy of, or modify, this frame)"
        n459 = call <vilib>:"Add State(s) to Queue__JKI_lib_State_Machine.vi"("State(s) in (\"\")"=w989) -> ("States Out"=w988:string)  [unwired: 14 in]
      }
      frame "Digitizer: ConfigMacro" {
        # "Digitizer Configuration Macro\n(Decide how to config digitizer)"
        n460 = case shown="\"iRFAndGain\", Default" "Task" {
          tunnel: "Channel" -> [w1001 w1007]
          tunnel: [w1000 w1006] -> w992
          frame "iRFAndGain", Default {
            n461 = case shown="\"Ch4\"" w1001 {
              tunnel: ["Digitizer: ConfigCh1iRF" ("State(s) at Back (\"\")") "Digitizer: ConfigCh2iRF" ("State(s) at Back (\"\")") "Digitizer: ConfigCh3iRF" ("State(s) at Back (\"\")") "Digitizer: ConfigCh4iRF" ("State(s) at Back (\"\")")] -> w1000
              frame "Ch1", Default {
              }
              frame "Ch2" {
              }
              frame "Ch3" {
              }
              frame "Ch4" {
              }
            }
          }
          frame "Alignment" {
            n462 = case shown="\"Ch4\"" w1007 {
              tunnel: ["Digitizer: ConfigCh1Align" ("State(s) at Back (\"\")") "Digitizer: ConfigCh2Align" ("State(s) at Back (\"\")") "Digitizer: ConfigCh3Align" ("State(s) at Back (\"\")") "Digitizer: ConfigCh4Align" ("State(s) at Back (\"\")")] -> w1006
              frame "Ch1", Default {
              }
              frame "Ch2" {
              }
              frame "Ch3" {
              }
              frame "Ch4" {
              }
            }
          }
        }
        n463 = call <vilib>:"Add State(s) to Queue__JKI_lib_State_Machine.vi"("State(s) in Front (\"\")"=w992, "State(s) in (\"\")"="Graph: SetXScale\nGraph: ClearHistory\nMacro: SysReadyForAqui" ("State(s) in (\"\")")) -> ("States Out"=w990:string)  [unwired: 13 in]
        n464 = call <vilib>:"Add State(s) to Queue__JKI_lib_State_Machine.vi"("State(s) in Front (\"\")"=w990, "State(s) in (\"\")"=w999) -> ("States Out"=w998:string)  [unwired: 13 in]
      }
      frame "Digitizer: Initialize" {
        # "Initialize digitizer.\nInitialize both digitizer and update status."
        n465 = call "FLImDAQ_FGV.vi"("error in (no error)"=w1018) -> ("error out"=w1012:errorcluster, "Read data"=w1017:T4)  [unwired: 9 in]
        n466 = property on="Digitizer" class="Bool (strict)"("Blinking"=TRUE) -> ()  [unwired: 2 in, 2 out]
        n467 = Unbundle By Name(w1017) -> ("Digitizer 1"=w1016:refnum<k15>, "Digitizer 2"=w1015:refnum<k15>)
        n468 = case shown="No Error" w1012 {
          selector: w1012 -> [w1025 w1029]
          tunnel: [w1028 w1029] -> w1020
          tunnel: w1015 -> [w1027 _]
          frame No Error {
            n469 = call <instrlib>:"niScope Initialize.vi"("resource name"=w1027, "reset device"=FALSE, "error in"=w1025) -> ("error out"=w1028:errorcluster)  [unwired: 11 in, 1 out]
          }
          frame Error {
          }
        }
        n470 = case shown="No Error" w1012 {
          selector: w1012 -> [w1031 w1034]
          tunnel: w1016 -> [w1033 _]
          tunnel: [w1030 w1034] -> w1013
          frame No Error {
            n471 = call <instrlib>:"niScope Initialize.vi"("resource name"=w1033, "reset device"=FALSE, "error in"=w1031) -> ("error out"=w1030:errorcluster)  [unwired: 11 in, 1 out]
          }
          frame Error {
          }
        }
        n472 = Merge Errors(w1013, w1020) -> (w1019:errorcluster)
        n473 = call <vilib>:"Add State(s) to Queue__JKI_lib_State_Machine.vi"("State(s) in (\"\")"=w1024) -> ("States Out"=w1023:string)  [unwired: 14 in]
      }
      frame "Digitizer: ConfigCh1iRF" {
        # "Synchronize is taking time ~3s."
        # "Config  digitizer\nCall subVi to config digitizer"
        n474 = Unbundle By Name(w1036) -> ("FLImDAQ"=w1037:T27)
        n475 = call "FLImDAQ_FGV.vi"() -> ("Read data"=w1043:T4)  [unwired: 10 in, 1 out]
        n476 = property on="Digitizer" class="Bool (strict)"(error in=w1046, "Blinking"=TRUE) -> (error out=w1041:errorcluster)  [unwired: 1 in, 1 out]
        n477 = Unbundle By Name(w1043) -> ("Digitizer 1"=w1045:refnum<k15>)
        n478 = Bundle By Name(cluster=w1037, "Channel"=enum16{"Channel 0", "Channel 1", "Channel 0&1"}."Channel 0") -> (w1039:T27)
        n479 = case shown="No Error" w1041 {
          selector: w1041 -> [w1054 w1057]
          tunnel: w1039 -> [w1053 _]
          tunnel: [w1056 w1057] -> w1040
          tunnel: w1045 -> [w1055 _]
          frame No Error {
            n480 = call "DigitizerConfig.vi"("error in (no error)"=w1054, "FLImDAQ"=w1053, "IVI Refnum in"=w1055) -> ("error out"=w1056:errorcluster)  [unwired: 7 in, 1 out]
          }
          frame Error {
          }
        }
        n481 = Unbundle By Name(w1040) -> ("status"=w1049:bool)
        n482 = property on="Digitizer" class="Bool (strict)"(error in=w1040, "Blinking"=FALSE) -> (error out=w1044:errorcluster)  [unwired: 1 in, 1 out]
        n483 = Not(x=w1049) -> (.not. x?=w1048:bool)
        n484 = Bundle By Name(cluster=w1036, "System Status.Digitizer"=w1048) -> (w1035:T22)
        n485 = call <vilib>:"Add State(s) to Queue__JKI_lib_State_Machine.vi"("State(s) in (\"\")"=w1052) -> ("States Out"=w1051:string)  [unwired: 14 in]
      }
      frame "Digitizer: ConfigCh2iRF" {
        # "Synchronize is taking time ~3s."
        # "Config  digitizer\nCall subVi to config digitizer"
        n486 = Unbundle By Name(w1059) -> ("FLImDAQ"=w1060:T27)
        n487 = call "FLImDAQ_FGV.vi"() -> ("Read data"=w1066:T4)  [unwired: 10 in, 1 out]
        n488 = property on="Digitizer" class="Bool (strict)"(error in=w1069, "Blinking"=TRUE) -> (error out=w1064:errorcluster)  [unwired: 1 in, 1 out]
        n489 = Unbundle By Name(w1066) -> ("Digitizer 1"=w1068:refnum<k15>)
        n490 = Bundle By Name(cluster=w1060, "Channel"=enum16{"Channel 0", "Channel 1", "Channel 0&1"}."Channel 1") -> (w1062:T27)
        n491 = case shown="No Error" w1064 {
          selector: w1064 -> [w1077 w1080]
          tunnel: w1062 -> [w1076 _]
          tunnel: [w1079 w1080] -> w1063
          tunnel: w1068 -> [w1078 _]
          frame No Error {
            n492 = call "DigitizerConfig.vi"("error in (no error)"=w1077, "FLImDAQ"=w1076, "IVI Refnum in"=w1078) -> ("error out"=w1079:errorcluster)  [unwired: 7 in, 1 out]
          }
          frame Error {
          }
        }
        n493 = Unbundle By Name(w1063) -> ("status"=w1072:bool)
        n494 = property on="Digitizer" class="Bool (strict)"(error in=w1063, "Blinking"=FALSE) -> (error out=w1067:errorcluster)  [unwired: 1 in, 1 out]
        n495 = Not(x=w1072) -> (.not. x?=w1071:bool)
        n496 = Bundle By Name(cluster=w1059, "System Status.Digitizer"=w1071) -> (w1058:T22)
        n497 = call <vilib>:"Add State(s) to Queue__JKI_lib_State_Machine.vi"("State(s) in (\"\")"=w1075) -> ("States Out"=w1074:string)  [unwired: 14 in]
      }
      frame "Digitizer: ConfigCh3iRF" {
        # "Hardcode channel to 0, which is Ch1 and Ch3."
        # "Synchronize is taking time ~3s."
        # "Config  digitizer\nCall subVi to config digitizer"
        n498 = Unbundle By Name(w1084) -> ("FLImDAQ"=w1085:T27)
        n499 = call "FLImDAQ_FGV.vi"() -> ("Read data"=w1109:T4)  [unwired: 10 in, 1 out]
        n500 = Bundle By Name(cluster=w1085, "Channel"=enum16{"Channel 0", "Channel 1", "Channel 0&1"}."Channel 0") -> (w1086:T27)
        n501 = Unbundle By Name(w1109) -> ("Digitizer 1"=w1112:refnum<k15>, "Digitizer 2"=w1111:refnum<k15>)
        n502 = property on="Digitizer" class="Bool (strict)"(error in=w1113, "Blinking"=TRUE) -> (error out=w1089:errorcluster)  [unwired: 1 in, 1 out]
        n503 = case shown="No Error" w1089 {
          selector: w1089 -> [w1129 w1132]
          tunnel: w1086 -> [w1128 _]
          tunnel: [w1131 w1132] -> w1088
          tunnel: w1112 -> [w1130 _]
          frame No Error {
            n504 = call "DigitizerConfig.vi"("error in (no error)"=w1129, "FLImDAQ"=w1128, "IVI Refnum in"=w1130) -> ("error out"=w1131:errorcluster)  [unwired: 7 in, 1 out]
          }
          frame Error {
          }
        }
        n505 = case shown="No Error" w1088 {
          selector: w1088 -> [w1122 w1127]
          tunnel: w1086 -> [w1121 _]
          tunnel: [w1125 w1127] -> w1095
          tunnel: w1111 -> [w1123 w1126]
          tunnel: [w1120 w1126] -> w1082
          frame No Error {
            n506 = call "DigitizerConfig.vi"("Config Trigger? (T)"=FALSE ("Config Trigge(T)r:"), "error in (no error)"=w1122, "FLImDAQ"=w1121, "IVI Refnum in"=w1123) -> ("error out"=w1125:errorcluster, "IVI Refnum out"=w1120:refnum<k15>)  [unwired: 6 in]
          }
          frame Error {
          }
        }
        n507 = call "Digitizer1_FGV.vi"("error in (no error)"=w1095, "Operation (Read)"=enum16{"Write", "Read"}."Read" ("Operation")) -> ("error out"=w1106:errorcluster, "Read data"=w1107:refnum<k15>)  [unwired: 8 in]
        n508 = call <instrlib>:"niScope Get Session Reference.vi"("instrument handle"=w1107, "error in"=w1106) -> ("session reference"=w1099:refnum<k20>, "error out"=w1097:errorcluster)  [unwired: 11 in, 1 out]
        n509 = call "Digitizer2_FGV.vi"("error in (no error)"=w1097, "Operation (Read)"=enum16{"Write", "Read"}."Read" ("Operation")) -> ("error out"=w1103:errorcluster, "Read data"=w1104:refnum<k15>)  [unwired: 8 in]
        n510 = call <instrlib>:"niScope Get Session Reference.vi"("instrument handle"=w1104, "error in"=w1103) -> ("session reference"=w1098:refnum<k20>, "error out"=w1096:errorcluster)  [unwired: 11 in, 1 out]
        n511 = Build Array(w1099, w1098) -> (w1102:refnum<k20>[])
        n512 = property class="niScope"(reference=w1082) -> ("Trigger Delay"=→"Triggering:Trigger Delay":dbl)  [unwired: 1 in, 2 out]
        n513 = call <instrlib>:"niTClk Configure For Homogeneous Triggers.vi"("error in (no error)"=w1096, "sessions"=w1102) -> ("error out"=w1101:errorcluster, "sessions out"=w1100:refnum<k20>[])  [unwired: 8 in]
        n514 = call <instrlib>:"niTClk Synchronize.vi"("error in (no error)"=w1101, "sessions"=w1100) -> ("error out"=w1094:errorcluster, "sessions out"=w1091:refnum<k20>[])  [unwired: 8 in]
        n515 = call <userlib>:"Wait (ms)__ogtk.vi"("error in (no error)"=w1094, "milliseconds to wait"=u32 1500) -> ("error out"=w1093:errorcluster)  [unwired: 8 in, 1 out]
        n516 = Unbundle By Name(w1093) -> ("status"=w1116:bool)
        n517 = Not(x=w1116) -> (.not. x?=w1115:bool)
        n518 = Bundle By Name(cluster=w1084, "System Status.Digitizer"=w1115, "niTClk sessions"=w1091) -> (w1083:T22)
        n519 = property on="Digitizer" class="Bool (strict)"(error in=w1093, "Blinking"=FALSE) -> (error out=w1110:errorcluster)  [unwired: 1 in, 1 out]
        n520 = call <vilib>:"Add State(s) to Queue__JKI_lib_State_Machine.vi"("State(s) in (\"\")"=w1119) -> ("States Out"=w1118:string)  [unwired: 14 in]
      }
      frame "Digitizer: ConfigCh4iRF" {
        # "Hardcode channel to 0, which is Ch2 and Ch4."
        # "Synchronize is taking time ~3s."
        # "Config  digitizer\nCall subVi to config digitizer"
        n521 = Unbundle By Name(w1136) -> ("FLImDAQ"=w1137:T27)
        n522 = call "FLImDAQ_FGV.vi"() -> ("Read data"=w1161:T4)  [unwired: 10 in, 1 out]
        n523 = Bundle By Name(cluster=w1137, "Channel"=enum16{"Channel 0", "Channel 1", "Channel 0&1"}."Channel 1") -> (w1138:T27)
        n524 = Unbundle By Name(w1161) -> ("Digitizer 1"=w1164:refnum<k15>, "Digitizer 2"=w1163:refnum<k15>)
        n525 = property on="Digitizer" class="Bool (strict)"(error in=w1165, "Blinking"=TRUE) -> (error out=w1141:errorcluster)  [unwired: 1 in, 1 out]
        n526 = case shown="No Error" w1141 {
          selector: w1141 -> [w1181 w1184]
          tunnel: w1138 -> [w1180 _]
          tunnel: [w1183 w1184] -> w1140
          tunnel: w1164 -> [w1182 _]
          frame No Error {
            n527 = call "DigitizerConfig.vi"("error in (no error)"=w1181, "FLImDAQ"=w1180, "IVI Refnum in"=w1182) -> ("error out"=w1183:errorcluster)  [unwired: 7 in, 1 out]
          }
          frame Error {
          }
        }
        n528 = case shown="No Error" w1140 {
          selector: w1140 -> [w1174 w1179]
          tunnel: w1138 -> [w1173 _]
          tunnel: [w1177 w1179] -> w1147
          tunnel: w1163 -> [w1175 w1178]
          tunnel: [w1172 w1178] -> w1134
          frame No Error {
            n529 = call "DigitizerConfig.vi"("Config Trigger? (T)"=FALSE ("Config Trigge(T)r:"), "error in (no error)"=w1174, "FLImDAQ"=w1173, "IVI Refnum in"=w1175) -> ("error out"=w1177:errorcluster, "IVI Refnum out"=w1172:refnum<k15>)  [unwired: 6 in]
          }
          frame Error {
          }
        }
        n530 = call "Digitizer1_FGV.vi"("error in (no error)"=w1147, "Operation (Read)"=enum16{"Write", "Read"}."Read" ("Operation")) -> ("error out"=w1158:errorcluster, "Read data"=w1159:refnum<k15>)  [unwired: 8 in]
        n531 = call <instrlib>:"niScope Get Session Reference.vi"("instrument handle"=w1159, "error in"=w1158) -> ("session reference"=w1151:refnum<k20>, "error out"=w1149:errorcluster)  [unwired: 11 in, 1 out]
        n532 = call "Digitizer2_FGV.vi"("error in (no error)"=w1149, "Operation (Read)"=enum16{"Write", "Read"}."Read" ("Operation")) -> ("error out"=w1155:errorcluster, "Read data"=w1156:refnum<k15>)  [unwired: 8 in]
        n533 = call <instrlib>:"niScope Get Session Reference.vi"("instrument handle"=w1156, "error in"=w1155) -> ("session reference"=w1150:refnum<k20>, "error out"=w1148:errorcluster)  [unwired: 11 in, 1 out]
        n534 = Build Array(w1151, w1150) -> (w1154:refnum<k20>[])
        n535 = property class="niScope"(reference=w1134) -> ("Trigger Delay"=w1133:dbl)  [unwired: 1 in, 2 out]
        n536 = call <instrlib>:"niTClk Configure For Homogeneous Triggers.vi"("error in (no error)"=w1148, "sessions"=w1154) -> ("error out"=w1153:errorcluster, "sessions out"=w1152:refnum<k20>[])  [unwired: 8 in]
        n537 = call <instrlib>:"niTClk Synchronize.vi"("error in (no error)"=w1153, "sessions"=w1152) -> ("error out"=w1146:errorcluster, "sessions out"=w1143:refnum<k20>[])  [unwired: 8 in]
        n538 = call <userlib>:"Wait (ms)__ogtk.vi"("error in (no error)"=w1146, "milliseconds to wait"=u32 1500) -> ("error out"=w1145:errorcluster)  [unwired: 8 in, 1 out]
        n539 = Unbundle By Name(w1145) -> ("status"=w1168:bool)
        n540 = Not(x=w1168) -> (.not. x?=w1167:bool)
        n541 = Bundle By Name(cluster=w1136, "System Status.Digitizer"=w1167, "niTClk sessions"=w1143) -> (w1135:T22)
        n542 = property on="Digitizer" class="Bool (strict)"(error in=w1145, "Blinking"=FALSE) -> (error out=w1162:errorcluster)  [unwired: 1 in, 1 out]
        n543 = local write "Triggering:Trigger Delay"(w1133) -> ()
        n544 = call <vilib>:"Add State(s) to Queue__JKI_lib_State_Machine.vi"("State(s) in (\"\")"=w1171) -> ("States Out"=w1170:string)  [unwired: 14 in]
      }
      frame "Digitizer: ConfigCh1Align" {
        # "Synchronize is taking time ~3s."
        # "Config  digitizer\nCall subVi to config digitizer"
        n545 = Unbundle By Name(w1187) -> ("FLImDAQ"=w1188:T27)
        n546 = call "FLImDAQ_FGV.vi"() -> ("Read data"=w1193:T4)  [unwired: 10 in, 1 out]
        n547 = property on="Digitizer" class="Bool (strict)"(error in=w1196, "Blinking"=TRUE) -> (error out=w1191:errorcluster)  [unwired: 1 in, 1 out]
        n548 = Unbundle By Name(w1193) -> ("Digitizer 1"=w1195:refnum<k15>)
        n549 = Bundle By Name(cluster=w1188, "Channel"=enum16{"Channel 0", "Channel 1", "Channel 0&1"}."Channel 0") -> (w1185:T27)
        n550 = case shown="No Error" w1191 {
          selector: w1191 -> [w1204 w1207]
          tunnel: w1185 -> [w1203 _]
          tunnel: [w1206 w1207] -> w1190
          tunnel: w1195 -> [w1205 _]
          frame No Error {
            n551 = call "DigitizerConfigGain.vi"("error in (no error)"=w1204, "FLImDAQ"=w1203, "IVI Refnum in"=w1205) -> ("error out"=w1206:errorcluster)  [unwired: 7 in, 1 out]
          }
          frame Error {
          }
        }
        n552 = Unbundle By Name(w1190) -> ("status"=w1199:bool)
        n553 = property on="Digitizer" class="Bool (strict)"(error in=w1190, "Blinking"=FALSE) -> (error out=w1194:errorcluster)  [unwired: 1 in, 1 out]
        n554 = Not(x=w1199) -> (.not. x?=w1198:bool)
        n555 = Bundle By Name(cluster=w1187, "System Status.Digitizer"=w1198) -> (w1186:T22)
        n556 = call <vilib>:"Add State(s) to Queue__JKI_lib_State_Machine.vi"("State(s) in (\"\")"=w1202) -> ("States Out"=w1201:string)  [unwired: 14 in]
      }
      frame "Digitizer: ConfigCh2Align" {
        # "Synchronize is taking time ~3s."
        # "Config  digitizer\nCall subVi to config digitizer"
        n557 = call "FLImDAQ_FGV.vi"() -> ("Read data"=w1216:T4)  [unwired: 10 in, 1 out]
        n558 = Unbundle By Name(w1209) -> ("FLImDAQ"=w1210:T27)
        n559 = Unbundle By Name(w1216) -> ("Digitizer 1"=w1218:refnum<k15>)
        n560 = Bundle By Name(cluster=w1210, "Channel"=enum16{"Channel 0", "Channel 1", "Channel 0&1"}."Channel 1") -> (w1212:T27)
        n561 = property on="Digitizer" class="Bool (strict)"(error in=w1219, "Blinking"=TRUE) -> (error out=w1214:errorcluster)  [unwired: 1 in, 1 out]
        n562 = case shown="No Error" w1214 {
          selector: w1214 -> [w1227 w1230]
          tunnel: w1212 -> [w1226 _]
          tunnel: [w1229 w1230] -> w1213
          tunnel: w1218 -> [w1228 _]
          frame No Error {
            n563 = call "DigitizerConfigGain.vi"("error in (no error)"=w1227, "FLImDAQ"=w1226, "IVI Refnum in"=w1228) -> ("error out"=w1229:errorcluster)  [unwired: 7 in, 1 out]
          }
          frame Error {
          }
        }
        n564 = Unbundle By Name(w1213) -> ("status"=w1222:bool)
        n565 = property on="Digitizer" class="Bool (strict)"(error in=w1213, "Blinking"=FALSE) -> (error out=w1217:errorcluster)  [unwired: 1 in, 1 out]
        n566 = Not(x=w1222) -> (.not. x?=w1221:bool)
        n567 = Bundle By Name(cluster=w1209, "System Status.Digitizer"=w1221) -> (w1208:T22)
        n568 = call <vilib>:"Add State(s) to Queue__JKI_lib_State_Machine.vi"("State(s) in (\"\")"=w1225) -> ("States Out"=w1224:string)  [unwired: 14 in]
      }
      frame "Digitizer: ConfigCh3Align" {
        # "Synchronize is taking time ~3s."
        # "Config  digitizer\nCall subVi to config digitizer"
        n569 = call "FLImDAQ_FGV.vi"() -> ("Read data"=w1242:T4)  [unwired: 10 in, 1 out]
        n570 = Unbundle By Name(w1232) -> ("FLImDAQ"=w1238:T27)
        n571 = Unbundle By Name(w1242) -> ("Digitizer 1"=w1236:refnum<k15>, "Digitizer 2"=w1231:refnum<k15>)
        n572 = Bundle By Name(cluster=w1238, "Channel"=enum16{"Channel 0", "Channel 1", "Channel 0&1"}."Channel 0") -> (w1235:T27)
        n573 = property on="Digitizer" class="Bool (strict)"(error in=w1244, "Blinking"=TRUE) -> (error out=w1234:errorcluster)  [unwired: 1 in, 1 out]
        n574 = Unbundle By Name(w1232) -> ()  [unwired: 1 out]
        n575 = case shown="No Error" w1234 {
          selector: w1234 -> [w1253 w1255]
          tunnel: w1235 -> [w1252 _]
          tunnel: w1236 -> [w1254 _]
          tunnel: [w1251 w1255] -> w1233
          frame No Error {
            n576 = call "DigitizerConfigGain.vi"("error in (no error)"=w1253, "FLImDAQ"=w1252, "IVI Refnum in"=w1254) -> ("error out"=w1251:errorcluster)  [unwired: 7 in, 1 out]
          }
          frame Error {
          }
        }
        n577 = case shown="No Error" w1233 {
          selector: w1233 -> [w1257 w1262]
          tunnel: w1235 -> [w1260 _]
          tunnel: [w1261 w1262] -> w1240
          tunnel: w1231 -> [w1259 _]
          frame No Error {
            n578 = call <instrlib>:"niScope Reset.vi"("instrument handle"=w1259, "error in"=w1257) -> ("instrument handle out"=w1258:refnum<k15>, "error out"=w1256:errorcluster)  [unwired: 12 in]
            n579 = call "DigitizerConfigGain.vi"("error in (no error)"=w1256, "FLImDAQ"=w1260, "IVI Refnum in"=w1258) -> ("error out"=w1261:errorcluster)  [unwired: 7 in, 1 out]
          }
          frame Error {
          }
        }
        n580 = Unbundle By Name(w1240) -> ("status"=w1247:bool)
        n581 = property on="Digitizer" class="Bool (strict)"(error in=w1240, "Blinking"=FALSE) -> (error out=w1243:errorcluster)  [unwired: 1 in, 1 out]
        n582 = Not(x=w1247) -> (.not. x?=w1246:bool)
        n583 = Bundle By Name(cluster=w1232, "System Status.Digitizer"=w1246) -> (w1237:T22)
        n584 = call <vilib>:"Add State(s) to Queue__JKI_lib_State_Machine.vi"("State(s) in (\"\")"=w1250) -> ("States Out"=w1249:string)  [unwired: 14 in]
      }
      frame "Digitizer: ConfigCh4Align" {
        # "Synchronize is taking time ~3s."
        # "Config  digitizer\nCall subVi to config digitizer"
        n585 = call "FLImDAQ_FGV.vi"() -> ("Read data"=w1274:T4)  [unwired: 10 in, 1 out]
        n586 = Unbundle By Name(w1264) -> ("FLImDAQ"=w1270:T27)
        n587 = Unbundle By Name(w1274) -> ("Digitizer 1"=w1268:refnum<k15>, "Digitizer 2"=w1263:refnum<k15>)
        n588 = Bundle By Name(cluster=w1270, "Channel"=enum16{"Channel 0", "Channel 1", "Channel 0&1"}."Channel 1") -> (w1267:T27)
        n589 = property on="Digitizer" class="Bool (strict)"(error in=w1276, "Blinking"=TRUE) -> (error out=w1266:errorcluster)  [unwired: 1 in, 1 out]
        n590 = Unbundle By Name(w1264) -> ()  [unwired: 1 out]
        n591 = case shown="No Error" w1266 {
          selector: w1266 -> [w1285 w1287]
          tunnel: w1267 -> [w1284 _]
          tunnel: w1268 -> [w1286 _]
          tunnel: [w1283 w1287] -> w1265
          frame No Error {
            n592 = call "DigitizerConfigGain.vi"("error in (no error)"=w1285, "FLImDAQ"=w1284, "IVI Refnum in"=w1286) -> ("error out"=w1283:errorcluster)  [unwired: 7 in, 1 out]
          }
          frame Error {
          }
        }
        n593 = case shown="No Error" w1265 {
          selector: w1265 -> [w1289 w1294]
          tunnel: w1267 -> [w1292 _]
          tunnel: [w1293 w1294] -> w1272
          tunnel: w1263 -> [w1291 _]
          frame No Error {
            n594 = call <instrlib>:"niScope Reset.vi"("instrument handle"=w1291, "error in"=w1289) -> ("instrument handle out"=w1290:refnum<k15>, "error out"=w1288:errorcluster)  [unwired: 12 in]
            n595 = call "DigitizerConfigGain.vi"("error in (no error)"=w1288, "FLImDAQ"=w1292, "IVI Refnum in"=w1290) -> ("error out"=w1293:errorcluster)  [unwired: 7 in, 1 out]
          }
          frame Error {
          }
        }
        n596 = Unbundle By Name(w1272) -> ("status"=w1279:bool)
        n597 = property on="Digitizer" class="Bool (strict)"(error in=w1272, "Blinking"=FALSE) -> (error out=w1275:errorcluster)  [unwired: 1 in, 1 out]
        n598 = Not(x=w1279) -> (.not. x?=w1278:bool)
        n599 = Bundle By Name(cluster=w1264, "System Status.Digitizer"=w1278) -> (w1269:T22)
        n600 = call <vilib>:"Add State(s) to Queue__JKI_lib_State_Machine.vi"("State(s) in (\"\")"=w1282) -> ("States Out"=w1281:string)  [unwired: 14 in]
      }
      frame "Digitizer: Start" {
        # "send trigger to start acquisition loop"
        # "initilize aquisition"
        # "Template Separator\n(You can make a copy of, or modify, this frame)"
        n601 = local read "Channel"() -> (w1295:enum32{"Ch1", "Ch2", "Ch3", "Ch4"})
        n602 = case shown="\"Ch3\"" w1295 {
          tunnel: w1302 -> [_ w1312 w1327]
          tunnel: [w1306 w1314 w1329] -> w1298
          tunnel: w1296 -> [w1309 w1313 w1328]
          frame "Ch1", "Ch2", Default {
            n603 = call "Digitizer1_FGV.vi"("error in (no error)"=w1309, "Operation (Read)"=enum16{"Write", "Read"}."Read" ("Operation")) -> ("error out"=w1308:errorcluster, "Read data"=w1307:refnum<k15>)  [unwired: 8 in]
            n604 = call <instrlib>:"niScope Initiate Acquisition.vi"("instrument handle"=w1307, "error in"=w1308) -> ("error out"=w1306:errorcluster)  [unwired: 12 in, 1 out]
          }
          frame "Ch3" {
            n605 = local read "Task"() -> (w1311:enum32{"iRFAndGain", "Alignment"})
            n606 = case shown="\"Alignment\"" w1311 {
              tunnel: [w1318 w1319] -> w1314
              tunnel: w1313 -> [w1317 w1323]
              tunnel: w1312 -> [w1315 _]
              frame "iRFAndGain", Default {
                n607 = Unbundle By Name(w1315) -> ("niTClk sessions"=w1316:refnum<k20>[])
                n608 = call <instrlib>:"niTClk Initiate.vi"("error in (no error)"=w1317, "sessions"=w1316) -> ("error out"=w1318:errorcluster)  [unwired: 8 in, 1 out]
              }
              frame "Alignment" {
                n609 = call "Digitizer1_FGV.vi"("error in (no error)"=w1323) -> ("error out"=w1324:errorcluster, "Read data"=w1325:refnum<k15>)  [unwired: 9 in]
                n610 = call <instrlib>:"niScope Initiate Acquisition.vi"("instrument handle"=w1325, "error in"=w1324) -> ("error out"=w1322:errorcluster)  [unwired: 12 in, 1 out]
                n611 = call "Digitizer2_FGV.vi"("error in (no error)"=w1322) -> ("error out"=w1321:errorcluster, "Read data"=w1320:refnum<k15>)  [unwired: 9 in]
                n612 = call <instrlib>:"niScope Initiate Acquisition.vi"("instrument handle"=w1320, "error in"=w1321) -> ("error out"=w1319:errorcluster)  [unwired: 12 in, 1 out]
              }
            }
          }
          frame "Ch4" {
            n613 = local read "Task"() -> (w1326:enum32{"iRFAndGain", "Alignment"})
            n614 = case shown="\"iRFAndGain\", Default" w1326 {
              tunnel: [w1333 w1334] -> w1329
              tunnel: w1328 -> [w1332 w1338]
              tunnel: w1327 -> [w1330 _]
              frame "iRFAndGain", Default {
                n615 = Unbundle By Name(w1330) -> ("niTClk sessions"=w1331:refnum<k20>[])
                n616 = call <instrlib>:"niTClk Initiate.vi"("error in (no error)"=w1332, "sessions"=w1331) -> ("error out"=w1333:errorcluster)  [unwired: 8 in, 1 out]
              }
              frame "Alignment" {
                n617 = call "Digitizer1_FGV.vi"("error in (no error)"=w1338) -> ("error out"=w1339:errorcluster, "Read data"=w1340:refnum<k15>)  [unwired: 9 in]
                n618 = call <instrlib>:"niScope Initiate Acquisition.vi"("instrument handle"=w1340, "error in"=w1339) -> ("error out"=w1337:errorcluster)  [unwired: 12 in, 1 out]
                n619 = call "Digitizer2_FGV.vi"("error in (no error)"=w1337) -> ("error out"=w1336:errorcluster, "Read data"=w1335:refnum<k15>)  [unwired: 9 in]
                n620 = call <instrlib>:"niScope Initiate Acquisition.vi"("instrument handle"=w1335, "error in"=w1336) -> ("error out"=w1334:errorcluster)  [unwired: 12 in, 1 out]
              }
            }
          }
        }
        n621 = Generate User Event(priority (normal)=usereventprio."high priority", user event=w1299, event data cluster=TRUE ("event data"), error in=w1298) -> (error out=w1297:errorcluster)  [unwired: 1 out]
        n622 = call <vilib>:"Add State(s) to Queue__JKI_lib_State_Machine.vi"("State(s) in (\"\")"=w1305) -> ("States Out"=w1304:string)  [unwired: 14 in]
      }
      frame "Digitizer: Abort" {
        # "Template Separator\n(You can make a copy of, or modify, this frame)"
        n623 = call "Digitizer1_FGV.vi"("error in (no error)"=w1342, "Operation (Read)"=enum16{"Write", "Read"}."Read" ("Operation")) -> ("error out"=w1349:errorcluster, "Read data"=w1346:refnum<k15>)  [unwired: 8 in]
        n624 = call "Digitizer2_FGV.vi"("error in (no error)"=w1342, "Operation (Read)"=enum16{"Write", "Read"}."Read" ("Operation")) -> ("error out"=w1345:errorcluster, "Read data"=w1347:refnum<k15>)  [unwired: 8 in]
        n625 = call <instrlib>:"niScope Abort.vi"("instrument handle"=w1346, "error in"=w1349) -> ("error out"=w1351:errorcluster)  [unwired: 12 in, 1 out]
        n626 = call <instrlib>:"niScope Abort.vi"("instrument handle"=w1347, "error in"=w1345) -> ("error out"=w1350:errorcluster)  [unwired: 12 in, 1 out]
        n627 = Merge Errors(w1351, w1350) -> (w1343:errorcluster)
        n628 = call <vilib>:"Add State(s) to Queue__JKI_lib_State_Machine.vi"("State(s) in (\"\")"=w1354) -> ("States Out"=w1353:string)  [unwired: 14 in]
      }
      frame "Digitizer: checkTemp" {
        w1362 = enum16{"Write", "Read"}."Read" ("Operation")
        # "Template Separator\n(You can make a copy of, or modify, this frame)"
        n629 = call "Digitizer1_FGV.vi"("error in (no error)"=w1358, "Operation (Read)"=w1362) -> ("error out"=w1364:errorcluster, "Read data"=w1365:refnum<k15>)  [unwired: 8 in]
        n630 = call "Digitizer2_FGV.vi"("error in (no error)"=w1358, "Operation (Read)"=w1362) -> ("error out"=w1360:errorcluster, "Read data"=w1361:refnum<k15>)  [unwired: 8 in]
        n631 = property on="Property Node" class="niScope"(reference=w1365, error in=w1364) -> (error out=w1356:errorcluster, "Device Temperature"=→"Dig1 Temp":dbl)  [unwired: 1 out]
        n632 = property on="Property Node" class="niScope"(reference=w1361, error in=w1360) -> (error out=w1355:errorcluster, "Device Temperature"=→"Dig2 Temp":dbl)  [unwired: 1 out]
        n633 = Merge Errors(w1356, w1355) -> (w1357:errorcluster)
        n634 = call <vilib>:"Add State(s) to Queue__JKI_lib_State_Machine.vi"("State(s) in (\"\")"=w1369) -> ("States Out"=w1368:string)  [unwired: 14 in]
      }
      frame "Digitizer: Close" {
        # "Close Digitizer"
        n635 = call "Digitizer1_FGV.vi"("error in (no error)"=w1377, "Operation (Read)"=enum16{"Write", "Read"}."Read" ("Operation")) -> ("error out"=w1379:errorcluster, "Read data"=w1383:refnum<k15>)  [unwired: 8 in]
        n636 = call "Digitizer2_FGV.vi"("error in (no error)"=w1377, "Operation (Read)"=enum16{"Write", "Read"}."Read" ("Operation")) -> ("error out"=w1378:errorcluster, "Read data"=w1381:refnum<k15>)  [unwired: 8 in]
        n637 = call <instrlib>:"niScope Close.vi"("instrument handle"=w1383, "error in"=w1379) -> ("error out"=w1376:errorcluster)  [unwired: 13 in]
        n638 = call <instrlib>:"niScope Close.vi"("instrument handle"=w1381, "error in"=w1378) -> ("error out"=w1375:errorcluster)  [unwired: 13 in]
        n639 = Merge Errors(w1376, w1375) -> (w1374:errorcluster)
        n640 = Unbundle By Name(w1374) -> ("status"=w1373:bool)
        n641 = Bundle By Name(cluster=w1371, "System Status.Digitizer"=w1373) -> (w1370:T22)
        n642 = call <vilib>:"Add State(s) to Queue__JKI_lib_State_Machine.vi"("State(s) in (\"\")"=w1385) -> ("States Out"=w1384:string)  [unwired: 14 in]
      }
      frame "---------- LabJack ----------" {
        # "Template Separator\n(You can make a copy of, or modify, this frame)"
        n643 = call <vilib>:"Add State(s) to Queue__JKI_lib_State_Machine.vi"("State(s) in (\"\")"=w1390) -> ("States Out"=w1389:string)  [unwired: 14 in]
      }
      frame "LabJack: AB_DC_Start" {
        # "Template Separator\n(You can make a copy of, or modify, this frame)"
        n644 = Unbundle By Name(w1394) -> ("LJ Pinout.AimingBeam PWM"=w1393:string)
        n645 = call "LabJack_FGV.vi"("Operation(Read)"=enum16{"Write", "Read"}."Read", "error in (no error)"=w1397) -> ("error out"=w1395:errorcluster, "Read data"=w1396:i32)  [unwired: 8 in]
        n646 = call "LJM_eWriteName.vi"("Handle In"=w1396, "Name"=w1393, "Value"=1.0, "error in"=w1395) -> ("error out"=w1391:errorcluster)  [unwired: 10 in, 1 out]
        n647 = call <vilib>:"Add State(s) to Queue__JKI_lib_State_Machine.vi"("State(s) in (\"\")"=w1401) -> ("States Out"=w1400:string)  [unwired: 14 in]
      }
      frame "LabJack: AB_DC_Stop" {
        # "Template Separator\n(You can make a copy of, or modify, this frame)"
        n648 = Unbundle By Name(w1405) -> ("LJ Pinout.AimingBeam PWM"=w1404:string)
        n649 = call "LabJack_FGV.vi"("Operation(Read)"=enum16{"Write", "Read"}."Read", "error in (no error)"=w1408) -> ("error out"=w1406:errorcluster, "Read data"=w1407:i32)  [unwired: 8 in]
        n650 = call "LJM_eWriteName.vi"("Handle In"=w1407, "Name"=w1404, "Value"=0.0, "error in"=w1406) -> ("error out"=w1402:errorcluster)  [unwired: 10 in, 1 out]
        n651 = call <vilib>:"Add State(s) to Queue__JKI_lib_State_Machine.vi"("State(s) in (\"\")"=w1412) -> ("States Out"=w1411:string)  [unwired: 14 in]
      }
      frame "LabJack: checkPedal" {
        # "Template Separator\n(You can make a copy of, or modify, this frame)"
        n652 = Unbundle By Name(w1417) -> ("LJ Pinout.Foot Pedal"=w1419:string)
        n653 = local read "Tab Control"() -> (w1416:T2)
        n654 = call "LabJack_FGV.vi"("Operation(Read)"=enum16{"Write", "Read"}."Read" ("Operation"), "error in (no error)"=w1421) -> ("error out"=w1423:errorcluster, "Read data"=w1424:i32)  [unwired: 8 in]
        n655 = Equal?(x=w1416, y=T17."IO Ststus" ("Tab Control")) -> (x = y?=w1414:bool)
        n656 = call "LJM_eReadName.vi"("Handle In"=w1424, "Name"=w1419, "error in"=w1423) -> ("Value"=w1413:dbl, "error out"=w1422:errorcluster)  [unwired: 10 in, 1 out]
        n657 = case shown="True" w1414 {
          tunnel: w1413 -> [_ w1433]
          frame False {
          }
          frame True {
            # "[Covers: REQ14]"
            # "If on IO tab, show foot pedal status"
            n658 = Equal To 0?(x=w1433) -> (x = 0?=w1432:bool)
            n659 = Select(t=FALSE, s=w1432, f=TRUE) -> (s? t:f=w1431:bool)
            n660 = local write "Foot Pedal"(w1431) -> ()
          }
        }
        n661 = case shown="1" w1413 {
          tunnel: [w1434 w1439] -> w1418
          tunnel: ["" ("State(s) in Front (\"\")") w1438] -> w1420
          tunnel: w1417 -> [w1434 w1437]
          frame 0, Default {
          }
          frame 1 {
            # "If Pedal pressed"
            n662 = Unbundle By Name(w1437) -> ("Last Trigger"=w1436:u32)
            n663 = Tick Count (ms)() -> (millisecond timer value=w1443:u32)
            n664 = Subtract(x=w1443, y=w1436) -> (x-y=w1442:u32)
            n665 = Greater Or Equal?(x=w1442, y=u32 2000) -> (x >= y?=w1440:bool)
            n666 = case shown="True" w1440 {
              tunnel: [w1444 w1449] -> w1439
              tunnel: ["" ("State(s) in Front (\"\")") w1448] -> w1438
              tunnel: w1437 -> [w1444 w1446]
              frame False {
              }
              frame True {
                n667 = Tick Count (ms)() -> (millisecond timer value=w1450:u32)
                n668 = Unbundle By Name(w1446) -> ("SysRunning?"=w1447:bool)
                n669 = case shown="True" w1447 {
                  tunnel: ["Macro: StartRun" ("State(s) in Front (\"\")") "Macro: StopRun" ("State(s) in Front (\"\")")] -> w1448
                  frame False {
                  }
                  frame True {
                  }
                }
                n670 = Bundle By Name(cluster=w1446, "Last Trigger"=w1450) -> (w1449:T22)
              }
            }
          }
        }
        n671 = call <vilib>:"Add State(s) to Queue__JKI_lib_State_Machine.vi"("State(s) in Front (\"\")"=w1420, "State(s) in (\"\")"=w1428) -> ("States Out"=w1427:string)  [unwired: 13 in]
      }
      frame "LabJack: ZeroV" {
        # "Just Zero V\nDO not update FGV and front panel\nWIll resume from last V"
        # "set bias to 0"
        # "Zero APD bias\n(You can make a copy of, or modify, this frame)"
        n672 = Unbundle By Name(w1454) -> ("LJ Pinout.Ch1 Bias"=w1460:string, "LJ Pinout.Ch2 Bias"=w1459:string, "LJ Pinout.Ch3 Bias"=w1458:string)
        n673 = Build Array(w1460, w1459, w1458) -> (w1453:string[])
        n674 = call "LabJack_FGV.vi"("Operation(Read)"=enum16{"Write", "Read"}."Read" ("Operation"), "error in (no error)"=w1456) -> ("error out"=w1461:errorcluster, "Read data"=w1462:i32)  [unwired: 8 in]
        n675 = call "LJM_eWriteNames.vi"("Handle In"=w1462, "aNames"=w1453, "aValuesIn"=dbl[] [0.0, 0.0, 0.0], "error in"=w1461) -> ("error out"=w1455:errorcluster)  [unwired: 9 in, 2 out]
        n676 = call <vilib>:"Add State(s) to Queue__JKI_lib_State_Machine.vi"("State(s) in (\"\")"=w1466) -> ("States Out"=w1465:string)  [unwired: 14 in]
      }
      frame "LabJack: SetV" {
        # "set bias to user specifid"
        # "Zero APD bias\n(You can make a copy of, or modify, this frame)"
        n677 = Unbundle By Name(w1470) -> ("LJ Pinout.Ch1 Bias"=w1474:string, "LJ Pinout.Ch2 Bias"=w1472:string, "LJ Pinout.Ch3 Bias"=w1471:string)
        n678 = local read "Channel"() -> (w1475:enum32{"Ch1", "Ch2", "Ch3", "Ch4"})
        n679 = call "V1FGV.vi"("Error In"=w1478, "action (write)"=enum16{"write", "read"}."read" ("action")) -> ("Error Out"=w1467:errorcluster, "V1 out"=w1473:dbl)  [unwired: 8 in]
        n680 = local write "Ctrl V"(w1473) -> ()
        n681 = case shown="\"Ch1\", Default" w1475 {
          tunnel: w1474 -> [w1484 _ _]
          tunnel: [w1484 w1485 w1486] -> w1469
          tunnel: w1472 -> [_ w1485 _]
          tunnel: w1471 -> [_ _ w1486]
          frame "Ch1", Default {
          }
          frame "Ch2" {
          }
          frame "Ch3" {
          }
        }
        n682 = call "LabJack_FGV.vi"("error in (no error)"=w1478) -> ("error out"=w1479:errorcluster, "Read data"=w1480:i32)  [unwired: 9 in]
        n683 = call "LJM_eWriteName.vi"("Handle In"=w1480, "Name"=w1469, "Value"=w1473, "error in"=w1479) -> ("error out"=w1476:errorcluster)  [unwired: 10 in, 1 out]
        n684 = Merge Errors(w1467, w1476) -> (w1477:errorcluster)
        n685 = call <vilib>:"Add State(s) to Queue__JKI_lib_State_Machine.vi"("State(s) in (\"\")"=w1483) -> ("States Out"=w1482:string)  [unwired: 14 in]
      }
      frame "LabJack: Open" {
        # "Initialize LabJack T7\nEstablish connection and initialize pins"
        n686 = call "LJ_Open.vi"("error in"=w1495) -> ("error out"=w1493:errorcluster, "Success?"=w1494:bool, "Handle Out"=w1491:i32)  [unwired: 8 in]
        n687 = call "LabJack_FGV.vi"("Operation(Read)"=enum16{"Write", "Read"}."Write" ("Operation"), "error in (no error)"=w1493, "Write data"=w1491) -> ("error out"=w1490:errorcluster)  [unwired: 7 in, 1 out]
        n688 = Bundle By Name(cluster=w1487, "System Status.Labjack"=w1494) -> (w1488:T22)
        n689 = call <vilib>:"Add State(s) to Queue__JKI_lib_State_Machine.vi"("State(s) in (\"\")"=w1497) -> ("States Out"=w1496:string)  [unwired: 14 in]
      }
      frame "LabJack: SetDefaultSub" {
        w1508 = enum16{"write", "read"}."write" ("action")
        w1521 = "_EF_ENABLE" ("string")
        # "1. Disable PWM\n2. Set all V to 0\n3. Set 355 relay to open\n4. Set LED to off"
        # "read once to set DIO to input"
        # "set all initila V to 0. Set footpedal to input. Set PWM to low. Set laser relay to open. Set LEDs to yellow."
        # "Set Labjack to correct input and output state and initial values"
        n690 = Unbundle By Name(w1507) -> ("LJ Pinout.355 PWM"=w1499:string, "LJ Pinout.AimingBeam PWM"=w1498:string, "LJ Pinout.Ch1 Bias"=w1505:string, "LJ Pinout.Ch2 Bias"=w1504:string, "LJ Pinout.Ch3 Bias"=w1503:string, "LJ Pinout.Laser Start/Stop"=w1502:string, "LJ Pinout.Red LED"=w1501:string, "LJ Pinout.Green LED"=w1500:string)
        n691 = call "V1FGV.vi"("Error In"=w1515, "action (write)"=w1508, "V1 in"=0.0) -> ("Error Out"=w1516:errorcluster, "V1 out"=w1509:dbl)  [unwired: 7 in]
        n692 = call "LabJack_FGV.vi"("Operation(Read)"=enum16{"Write", "Read"}."Read" ("Operation"), "error in (no error)"=w1515) -> ("error out"=w1524:errorcluster, "Read data"=w1525:i32)  [unwired: 8 in]
        n693 = local write "Ctrl V"(w1509) -> ()
        n694 = call "V2FGV.vi"("Error In"=w1516, "action(write)"=w1508, "V2 in"=0.0) -> ("Error Out"=w1513:errorcluster)  [unwired: 7 in, 1 out]
        n695 = Concatenate Strings(w1499, w1521) -> (w1520:string)
        n696 = Concatenate Strings(w1498, w1521) -> (w1519:string)
        n697 = call "V3FGV.vi"("Error In"=w1513, "action(write)"=w1508, "V3 in"=0.0) -> ("Error Out"=w1510:errorcluster)  [unwired: 7 in, 1 out]
        n698 = Build Array(w1499, w1498, w1520, w1519, w1505, w1504, w1503, w1502, w1501, w1500) -> (w1528:string[])
        n699 = Unbundle By Name(w1507) -> ("LJ Pinout.Foot Pedal"=w1506:string)
        n700 = call "LJM_eWriteNames.vi"("Handle In"=w1525, "aNames"=w1528, "aValuesIn"=dbl[] [0.0, 0.0, 0.0, 0.0, 0.0, 0.0, 0.0, 0.0, 0.0, 0.0], "error in"=w1524) -> ("Handle Out"=w1523:i32, "error out"=w1522:errorcluster)  [unwired: 9 in, 1 out]
        n701 = call "LJM_eReadName.vi"("Handle In"=w1523, "Name"=w1506, "error in"=w1522) -> ("error out"=w1512:errorcluster)  [unwired: 10 in, 2 out]
        n702 = Merge Errors(w1512, w1510) -> (w1511:errorcluster)
        n703 = call <vilib>:"Add State(s) to Queue__JKI_lib_State_Machine.vi"("State(s) in (\"\")"=w1531) -> ("States Out"=w1530:string)  [unwired: 14 in]
      }
      frame "LabJack: FootPedalConfig" {
        # "Setup footPedal\n(You can make a copy of, or modify, this frame)"
        n704 = call "LabJack_FGV.vi"("Operation(Read)"=enum16{"Write", "Read"}."Read" ("Operation"), "error in (no error)"=w1533) -> ("error out"=w1537:errorcluster, "Read data"=w1538:i32)  [unwired: 8 in]
        n705 = call "LJM_eWriteName.vi"("Handle In"=w1538, "Name"="DIO15", "Value"=1.0, "error in"=w1537) -> ("error out"=w1534:errorcluster)  [unwired: 10 in, 1 out]
        n706 = call <vilib>:"Add State(s) to Queue__JKI_lib_State_Machine.vi"("State(s) in (\"\")"=w1542) -> ("States Out"=w1541:string)  [unwired: 14 in]
      }
      frame "LabJack: SetDefaultAndClose" {
        # "Template Separator\n(You can make a copy of, or modify, this frame)"
        n707 = call <vilib>:"Add State(s) to Queue__JKI_lib_State_Machine.vi"("State(s) in Front (\"\")"="LabJack: SetDefaultSub\nLabJack: Close" ("State(s) in Front (\"\")"), "State(s) in (\"\")"=w1548) -> ("States Out"=w1547:string)  [unwired: 13 in]
      }
      frame "LabJack: Close" {
        # "Close LabJack Refnum"
        n708 = call "LabJack_FGV.vi"("Operation(Read)"=enum16{"Write", "Read"}."Read" ("Operation"), "error in (no error)"=w1555) -> ("error out"=w1551:errorcluster, "Read data"=w1552:i32)  [unwired: 8 in]
        n709 = Bundle By Name(cluster=w1549, "System Status.Labjack"=FALSE ("System Status.Gain Control")) -> (w1550:T22)
        n710 = call "LJM_Close.vi"("error in"=w1551, "Handle"=w1552) -> ("error out"=w1557:errorcluster)  [unwired: 9 in]
        n711 = call <vilib>:"Add State(s) to Queue__JKI_lib_State_Machine.vi"("State(s) in (\"\")"=w1559) -> ("States Out"=w1558:string)  [unwired: 14 in]
      }
      frame "LabJack: Interlock enable/disable" {
        w1568 = i8 0  # int8
        # "Interlock enable/disable\n(Usage: \"LabJack: Interlock enable/disable >> 1|0\")"
        n712 = Fract/Exp String To Number(string=w1569, default (0 dbl)=w1568) -> (number=w1567:i8)  [unwired: 2 in, 1 out]
        n713 = Unbundle By Name(w1561) -> ("LJ Pinout.Interlock"=w1560:string)
        n714 = call "LabJack_FGV.vi"("Operation(Read)"=enum16{"Write", "Read"}."Read" ("Operation")) -> ("Read data"=w1565:i32)  [unwired: 9 in, 1 out]
        n715 = call "LJM_eWriteName.vi"("Handle In"=w1565, "Name"=w1560, "Value"=w1567, "error in"=w1566) -> ("error out"=w1563:errorcluster)  [unwired: 10 in, 1 out]
        n716 = call <vilib>:"Add State(s) to Queue__JKI_lib_State_Machine.vi"("State(s) in (\"\")"=w1571) -> ("States Out"=w1570:string)  [unwired: 14 in]
      }
      frame "LabJack: 355_PWM_Config" {
        w1581 = 0.0 ("element")
        w1594 = "DIO_EF_CLOCK1_ENABLE"
        # "Config PWM frequency"
        n717 = Unbundle By Name(w1579) -> ("LJ Pinout.355 PWM"=w1573:string)
        n718 = Unbundle By Name(w1579) -> ("355 PWM setting.DIO_EF_CLOCK1_DIVISOR"=w1578:i16, "355 PWM setting.DIO_EF_CLOCK1_ROLL_VALUE"=w1577:i32, "355 PWM setting.DIO#_EF_INDEX"=w1576:i16, "355 PWM setting.DIO#_EF_OPTIONS"=w1575:i16, "355 PWM setting.DIO#_EF_CONFIG_A"=w1574:i32)
        n719 = Concatenate Strings(w1573, "_EF_ENABLE" ("string")) -> (w1590:string)
        n720 = Concatenate Strings(w1573, "_EF_INDEX") -> (w1593:string)
        n721 = Concatenate Strings(w1573, "_EF_OPTIONS") -> (w1592:string)
        n722 = Concatenate Strings(w1573, "_EF_CONFIG_A") -> (w1591:string)
        n723 = call "LabJack_FGV.vi"("Operation(Read)"=enum16{"Write", "Read"}."Read" ("Operation")) -> ("Read data"=w1588:i32)  [unwired: 9 in, 1 out]
        n724 = Build Array(w1581, w1581, w1578, w1577, 1.0 ("element"), 0.0 ("element"), w1576, w1575, w1574) -> (w1585:dbl[])
        n725 = Build Array("DIO_EF_CLOCK0_ENABLE", w1594, "DIO_EF_CLOCK1_DIVISOR", "DIO_EF_CLOCK1_ROLL_VALUE", w1594, w1590, w1593, w1592, w1591) -> (w1589:string[])
        n726 = call "LJM_eWriteNames.vi"("Handle In"=w1588, "aNames"=w1589, "aValuesIn"=w1585, "error in"=w1583) -> ("error out"=w1584:errorcluster)  [unwired: 9 in, 2 out]
        n727 = call <vilib>:"Add State(s) to Queue__JKI_lib_State_Machine.vi"("State(s) in (\"\")"=w1602) -> ("States Out"=w1601:string)  [unwired: 14 in]
      }
      frame "LabJack: AB_PWM_Config" {
        w1614 = 0.0 ("element")
        w1625 = "DIO_EF_CLOCK2_ENABLE"
        # "Set PWM to ground so AB is disabled"
        # "Config PWM frequency"
        n728 = Unbundle By Name(w1612) -> ("LJ Pinout.AimingBeam PWM"=w1603:string)
        n729 = Unbundle By Name(w1612) -> ("AB PWM setting.DIO_EF_CLOCK1_DIVISOR"=w1611:i16, "AB PWM setting.DIO_EF_CLOCK1_ROLL_VALUE"=w1610:i32, "AB PWM setting.DIO#_EF_INDEX"=w1609:i16, "AB PWM setting.DIO#_EF_OPTIONS"=w1608:i16, "AB PWM setting.DIO#_EF_CONFIG_A"=w1607:i32)
        n730 = Concatenate Strings(w1603, "_EF_ENABLE" ("string")) -> (w1621:string)
        n731 = Concatenate Strings(w1603, "_EF_INDEX") -> (w1624:string)
        n732 = Concatenate Strings(w1603, "_EF_OPTIONS") -> (w1623:string)
        n733 = Concatenate Strings(w1603, "_EF_CONFIG_A") -> (w1622:string)
        n734 = Build Array(w1614, w1614, w1611, w1610, 1.0 ("element"), 0.0 ("element"), w1609, w1608, w1607) -> (w1617:dbl[])
        n735 = call "LabJack_FGV.vi"("Operation(Read)"=enum16{"Write", "Read"}."Read" ("Operation"), "error in (no error)"=w1604) -> ("error out"=w1605:errorcluster, "Read data"=w1606:i32)  [unwired: 8 in]
        n736 = Build Array("DIO_EF_CLOCK0_ENABLE", w1625, "DIO_EF_CLOCK2_DIVISOR", "DIO_EF_CLOCK2_ROLL_VALUE", w1625, w1621, w1624, w1623, w1622) -> (w1620:string[])
        n737 = call "LJM_eWriteNames.vi"("Handle In"=w1606, "aNames"=w1620, "aValuesIn"=w1617, "error in"=w1605) -> ("error out"=w1616:errorcluster)  [unwired: 9 in, 2 out]
        n738 = call <vilib>:"Add State(s) to Queue__JKI_lib_State_Machine.vi"("State(s) in (\"\")"=w1634) -> ("States Out"=w1633:string)  [unwired: 14 in]
      }
      frame "LabJack: 355_PWM_Start" {
        # "Template Separator\n(You can make a copy of, or modify, this frame)"
        n739 = Unbundle By Name(w1636) -> ("LJ Pinout.355 PWM"=w1635:string)
        n740 = call "LabJack_FGV.vi"("Operation(Read)"=enum16{"Write", "Read"}."Read" ("Operation"), "error in (no error)"=w1638) -> ("error out"=w1643:errorcluster, "Read data"=w1644:i32)  [unwired: 8 in]
        n741 = Concatenate Strings(w1635, "_EF_ENABLE" ("string")) -> (w1641:string)
        n742 = call "LJM_eWriteName.vi"("Handle In"=w1644, "Name"=w1641, "Value"=1.0, "error in"=w1643) -> ("error out"=w1639:errorcluster)  [unwired: 10 in, 1 out]
        n743 = call <vilib>:"Add State(s) to Queue__JKI_lib_State_Machine.vi"("State(s) in (\"\")"=w1647) -> ("States Out"=w1646:string)  [unwired: 14 in]
      }
      frame "LabJack: AB_PWM_Start" {
        # "Template Separator\n(You can make a copy of, or modify, this frame)"
        n744 = Unbundle By Name(w1649) -> ("LJ Pinout.AimingBeam PWM"=w1648:string)
        n745 = call "LabJack_FGV.vi"("Operation(Read)"=enum16{"Write", "Read"}."Read" ("Operation"), "error in (no error)"=w1651) -> ("error out"=w1656:errorcluster, "Read data"=w1657:i32)  [unwired: 8 in]
        n746 = Concatenate Strings(w1648, "_EF_ENABLE" ("string")) -> (w1654:string)
        n747 = call "LJM_eWriteName.vi"("Handle In"=w1657, "Name"=w1654, "Value"=1.0, "error in"=w1656) -> ("error out"=w1652:errorcluster)  [unwired: 10 in, 1 out]
        n748 = call <vilib>:"Add State(s) to Queue__JKI_lib_State_Machine.vi"("State(s) in (\"\")"=w1660) -> ("States Out"=w1659:string)  [unwired: 14 in]
      }
      frame "LabJack: 355_PWM_Stop" {
        # "Template Separator\n(You can make a copy of, or modify, this frame)"
        n749 = Unbundle By Name(w1663) -> ("LJ Pinout.355 PWM"=w1662:string)
        n750 = call "LabJack_FGV.vi"("Operation(Read)"=enum16{"Write", "Read"}."Read" ("Operation"), "error in (no error)"=w1668) -> ("error out"=w1671:errorcluster, "Read data"=w1666:i32)  [unwired: 8 in]
        n751 = Concatenate Strings(w1662, "_EF_ENABLE" ("string")) -> (w1669:string)
        n752 = call "LJM_eWriteName.vi"("Handle In"=w1666, "Name"=w1669, "Value"=0.0, "error in"=w1671) -> ("error out"=w1664:errorcluster)  [unwired: 10 in, 1 out]
        n753 = local write "355nm Laser toggle"(FALSE ("355nm Laser toggle")) -> ()
        n754 = call <vilib>:"Add State(s) to Queue__JKI_lib_State_Machine.vi"("State(s) in (\"\")"=w1674) -> ("States Out"=w1673:string)  [unwired: 14 in]
      }
      frame "LabJack: AB_PWM_Stop" {
        # "Template Separator\n(You can make a copy of, or modify, this frame)"
        n755 = Unbundle By Name(w1676) -> ("LJ Pinout.AimingBeam PWM"=w1675:string)
        n756 = call "LabJack_FGV.vi"("Operation(Read)"=enum16{"Write", "Read"}."Read" ("Operation"), "error in (no error)"=w1679) -> ("error out"=w1684:errorcluster, "Read data"=w1685:i32)  [unwired: 8 in]
        n757 = Concatenate Strings(w1675, "_EF_ENABLE" ("string")) -> (w1682:string)
        n758 = call "LJM_eWriteName.vi"("Handle In"=w1685, "Name"=w1682, "Value"=0.0, "error in"=w1684) -> ("error out"=w1680:errorcluster)  [unwired: 10 in, 1 out]
        n759 = local write "Aiming beam toggle"(FALSE ("Aiming beam toggle")) -> ()
        n760 = call <vilib>:"Add State(s) to Queue__JKI_lib_State_Machine.vi"("State(s) in (\"\")"=w1688) -> ("States Out"=w1687:string)  [unwired: 14 in]
      }
      frame "---------- LED ----------" {
        # "Template Separator\n(You can make a copy of, or modify, this frame)"
        n761 = call <vilib>:"Add State(s) to Queue__JKI_lib_State_Machine.vi"("State(s) in (\"\")"=w1693) -> ("States Out"=w1692:string)  [unwired: 14 in]
      }
      frame "LED: BreathGreen" {
        w1696 = FALSE ("Wait Until Done")
        # "breath LED Green\n(Run VI in background using VI server to breath LED green )"
        n762 = Unbundle By Name(w1702) -> ("LED vi reference"=w1701:refnum<vi>)
        n763 = invoke class="VI" method="Ctrl Val.Set"(reference=w1701, error in=w1694, "Control Name"="Color", "Value"=0) -> (reference out=w1698:refnum<vi>, error out=w1697:errorcluster)  [unwired: 1 in, 3 out]
        n764 = invoke class="VI" method="Run VI"(reference=w1698, error in=w1697, "Wait until done"=w1696, "Auto Dispose Ref"=w1696) -> (error out=w1695:errorcluster)  [unwired: 1 in, 4 out]
        n765 = call <vilib>:"Add State(s) to Queue__JKI_lib_State_Machine.vi"("State(s) in (\"\")"=w1705) -> ("States Out"=w1704:string)  [unwired: 14 in]
      }
      frame "LED: BreathOrange" {
        w1708 = FALSE ("Wait Until Done")
        # "breath LED Green\n(Run VI in background using VI server to breath LED green )"
        n766 = Unbundle By Name(w1714) -> ("LED vi reference"=w1713:refnum<vi>)
        n767 = invoke class="VI" method="Ctrl Val.Set"(reference=w1713, error in=w1706, "Control Name"="Color", "Value"=1) -> (reference out=w1710:refnum<vi>, error out=w1709:errorcluster)  [unwired: 1 in, 3 out]
        n768 = invoke class="VI" method="Run VI"(reference=w1710, error in=w1709, "Wait until done"=w1708, "Auto Dispose Ref"=w1708) -> (error out=w1707:errorcluster)  [unwired: 1 in, 4 out]
        n769 = call <vilib>:"Add State(s) to Queue__JKI_lib_State_Machine.vi"("State(s) in (\"\")"=w1717) -> ("States Out"=w1716:string)  [unwired: 14 in]
      }
      frame "LED: OpenVIRef" {
        # "Open LED vi ref\n(You can make a copy of, or modify, this frame)"
        n770 = call <vilib>:"Application Directory.vi"() -> ("Application Directory"=w1722:path)
        n771 = Build Path(base path=w1722, name or relative path="SubVI") -> (appended path=w1720:path)
        n772 = Build Path(base path=w1720, name or relative path="LEDBreath.vi") -> (appended path=w1718:path)
        n773 = Open VI Reference(vi path=w1718, error in (no error)=w1727) -> (vi reference=w1724:refnum<vi>, error out=w1726:errorcluster)  [unwired: 4 in]
        n774 = case shown="No Error" w1726 {
          tunnel: w1725 -> [w1731 w1735]
          tunnel: w1724 -> [w1734 _]
          tunnel: [w1732 w1735] -> w1723
          frame No Error {
            n775 = Bundle By Name(cluster=w1731, "LED vi reference"=w1734, "LedViRefOpen"=TRUE) -> (w1732:T22)
          }
          frame Error {
          }
        }
        n776 = call <vilib>:"Add State(s) to Queue__JKI_lib_State_Machine.vi"("State(s) in (\"\")"=w1730) -> ("States Out"=w1729:string)  [unwired: 14 in]
      }
      frame "LED: CloseVIRef" {
        # "Template Separator\n(You can make a copy of, or modify, this frame)"
        n777 = Unbundle By Name(w1737) -> ("LedViRefOpen"=w1736:bool, "LED vi reference"=w1739:refnum<vi>)
        n778 = case shown="True" w1736 {
          tunnel: w1740 -> [w1744 w1747]
          tunnel: w1739 -> [_ w1745]
          tunnel: [w1744 w1746] -> w1738
          frame False {
          }
          frame True {
            n779 = Close Reference(reference=w1745, error in (no error)=w1747) -> (error out=w1746:errorcluster)
          }
        }
        n780 = call <vilib>:"Add State(s) to Queue__JKI_lib_State_Machine.vi"("State(s) in (\"\")"=w1743) -> ("States Out"=w1742:string)  [unwired: 14 in]
      }
      frame "LED: BreathOff" {
        # "System LED Breath Off\n(LED breath off"
        n781 = Unbundle By Name(w1754) -> ("LED vi reference"=w1756:refnum<vi>)
        n782 = invoke on="Invoke Node" class="VI" method="Ctrl Val.Set"(reference=w1756, error in=w1755, "Control Name"="Stop", "Value"=TRUE) -> (reference out=w1750:refnum<vi>, error out=w1751:errorcluster)  [unwired: 1 in, 3 out]
        n783 = case shown="No Error" w1751 {
          selector: w1751 -> [w1761 _]
          tunnel: [w1760 errorcluster {"status"=FALSE, "code"=0, "source"=""} ("error IO")] -> w1748
          tunnel: ["" ("State(s) in Front (\"\")") "LED: BreathOff" ("State(s) in Front (\"\")")] -> w1749
          tunnel: w1750 -> [w1762 _]
          frame No Error {
            # "No error, wait for VI to stop"
            n784 = while {
              tunnel: w1762 -> [w1770]
              shift-right: [w1764] -> w1760
              shift-left: w1761 -> [w1769]
              stop <- w1766 stop-if-true
              # "continue check whether vi is running"
              n785 = property class="VI"(reference=w1770, error in=w1769) -> (error out=w1764:errorcluster, "Exec.State"=w1768:T18)  [unwired: 1 out]
              n786 = Wait (ms)(milliseconds to wait=u32 50) -> ()  [unwired: 1 out]
              n787 = Equal?(x=w1768, y=T18."Idle") -> (x = y?=w1766:bool)
            }
          }
          frame Error {
            # "try again when error"
          }
        }
        n788 = call <vilib>:"Add State(s) to Queue__JKI_lib_State_Machine.vi"("State(s) in Front (\"\")"=w1749, "State(s) in (\"\")"=w1759) -> ("States Out"=w1758:string)  [unwired: 13 in]
      }
      frame "LED: Off" {
        # "set LED to red"
        # "Template Separator\n(You can make a copy of, or modify, this frame)"
        n789 = Unbundle By Name(w1775) -> ("LJ Pinout.Red LED"=w1774:string, "LJ Pinout.Green LED"=w1773:string)
        n790 = call "LabJack_FGV.vi"("Operation(Read)"=enum16{"Write", "Read"}."Read" ("Operation"), "error in (no error)"=w1776) -> ("error out"=w1783:errorcluster, "Read data"=w1782:i32)  [unwired: 8 in]
        n791 = call "LJM_eWriteName.vi"("Handle In"=w1782, "Name"=w1774, "Value"=0.0, "error in"=w1783) -> ("Handle Out"=w1780:i32, "error out"=w1779:errorcluster)  [unwired: 10 in]
        n792 = call "LJM_eWriteName.vi"("Handle In"=w1780, "Name"=w1773, "Value"=0.0, "error in"=w1779) -> ("error out"=w1777:errorcluster)  [unwired: 10 in, 1 out]
        n793 = call <vilib>:"Add State(s) to Queue__JKI_lib_State_Machine.vi"("State(s) in (\"\")"=w1787) -> ("States Out"=w1786:string)  [unwired: 14 in]
      }
      frame "LED: Green" {
        # "set LED to green"
        # "Template Separator\n(You can make a copy of, or modify, this frame)"
        n794 = Unbundle By Name(w1790) -> ("LJ Pinout.Red LED"=w1789:string, "LJ Pinout.Green LED"=w1788:string)
        n795 = call "LabJack_FGV.vi"("Operation(Read)"=enum16{"Write", "Read"}."Read" ("Operation"), "error in (no error)"=w1793) -> ("error out"=w1799:errorcluster, "Read data"=w1798:i32)  [unwired: 8 in]
        n796 = call "LJM_eWriteName.vi"("Handle In"=w1798, "Name"=w1789, "Value"=0.0, "error in"=w1799) -> ("Handle Out"=w1796:i32, "error out"=w1795:errorcluster)  [unwired: 10 in]
        n797 = call "LJM_eWriteName.vi"("Handle In"=w1796, "Name"=w1788, "Value"=9.0, "error in"=w1795) -> ("error out"=w1792:errorcluster)  [unwired: 10 in, 1 out]
        n798 = call <vilib>:"Add State(s) to Queue__JKI_lib_State_Machine.vi"("State(s) in (\"\")"=w1802) -> ("States Out"=w1801:string)  [unwired: 14 in]
      }
      frame "---------- Queue ----------" {
        # "Template Separator\n(You can make a copy of, or modify, this frame)"
        n799 = call <vilib>:"Add State(s) to Queue__JKI_lib_State_Machine.vi"("State(s) in (\"\")"=w1807) -> ("States Out"=w1806:string)  [unwired: 14 in]
      }
      frame "Queue: CheckCtrlVQ" {
        # "Check control V queue\n(if contorl V queue is not empty, aquire data)"
        n800 = Unbundle By Name(w1812) -> ("SysRunning?"=w1811:bool)
        n801 = case shown="False" w1811 {
          tunnel: w1808 -> [w1824 w1841]
          tunnel: w1813 -> [w1823 _]
          tunnel: [w1819 "" ("State with Arguments")] -> w1810
          tunnel: [w1817 w1841] -> w1809
          frame False {
            # "system idle"
            n802 = Get Queue Status(queue=w1823, error in (no error)=w1824) -> (queue out=w1821:refnum<queue>, error out=w1820:errorcluster, # elements in queue=w1818:i32)  [unwired: 1 in, 5 out]
            n803 = Greater Than 0?(x=w1818) -> (x > 0?=w1822:bool)
            n804 = case shown="True" w1822 {
              tunnel: w1821 -> [_ w1838]
              tunnel: w1820 -> [w1825 w1837]
              tunnel: ["" ("State with Arguments") w1829] -> w1819
              tunnel: w1818 -> [_ w1833]
              tunnel: [w1825 w1827] -> w1817
              frame False {
              }
              frame True {
                n805 = Dequeue Element(queue=w1838, error in (no error)=w1837) -> (element=w1834:dbl, error out=w1827:errorcluster)  [unwired: 1 in, 2 out]
                n806 = Equal?(x=w1833, y=1) -> (x = y?=w1831:bool)
                n807 = Number To Fractional String(number=w1834) -> (F-format string=w1835:string)  [unwired: 3 in]
                n808 = case shown="True" w1831 {
                  tunnel: ["" ("Empty String Constant") "Data: parseDataAllGainMacro\nMacro: AskOverWrite"] -> w1828
                  frame False {
                  }
                  frame True {
                    # "if last control V, parse all data and ask whether to over-write"
                  }
                }
                n809 = call <vilib>:"Build State String with Arguments__JKI_lib_State_Machine.vi"("Arguments (\"\")"=w1835, "State"="Aquisition: RecordData") -> ("State with Arguments"=w1830:string)  [unwired: 4 in]
                n810 = call <vilib>:"Add State(s) to Queue__JKI_lib_State_Machine.vi"("State(s) in Front (\"\")"=w1830, "State(s) in (\"\")"=w1828) -> ("States Out"=w1829:string)  [unwired: 13 in]
              }
            }
          }
          frame True {
            # "System running"
          }
        }
        n811 = call <vilib>:"Add State(s) to Queue__JKI_lib_State_Machine.vi"("State(s) in Front (\"\")"=w1810, "State(s) in (\"\")"=w1816) -> ("States Out"=w1815:string)  [unwired: 13 in]
      }
      frame "Queue: FlashDataAllQueue" {
        # "Flash control V queue and DataAll queue\n(You can make a copy of, or modify, this frame)"
        n812 = Flush Queue(queue=w1848, error in (no error)=w1845) -> (error out=w1846:errorcluster)  [unwired: 2 out]
        n813 = Flush Queue(queue=w1850, error in (no error)=w1845) -> (error out=w1849:errorcluster)  [unwired: 2 out]
        n814 = Flush Queue(queue=w1844, error in (no error)=w1845) -> (error out=w1843:errorcluster)  [unwired: 2 out]
        n815 = Merge Errors(w1846, w1849, w1843) -> (w1847:errorcluster)
        n816 = call <vilib>:"Add State(s) to Queue__JKI_lib_State_Machine.vi"("State(s) in (\"\")"=w1854) -> ("States Out"=w1853:string)  [unwired: 14 in]
      }
      frame "Queue: CheckNumOfWF" {
        # "Template Separator\n(You can make a copy of, or modify, this frame)"
        n817 = call "FLImDAQ_FGV.vi"() -> ("Read data"=w1857:T4)  [unwired: 10 in, 1 out]
        n818 = Unbundle By Name(w1857) -> ("Waveform to Avg"=w1856:i16)
        n819 = Get Queue Status(queue=w1859) -> (# elements in queue=w1858:i32)  [unwired: 2 in, 7 out]
        n820 = Multiply(x=w1858, y=w1856) -> (x*y=w1855:i32)
        "numWFInQ" <- w1855
        n821 = Greater Or Equal?(x=w1855, y="Num WF to acquire") -> (x >= y?=w1861:bool)
        n822 = case shown="False" w1861 {
          tunnel: ["Queue: CheckNumOfWF" ("State(s) in Front (\"\")") "" ("State(s) in Front (\"\")")] -> w1860
          frame False {
            n823 = Wait (ms)(milliseconds to wait=u32 5) -> ()  [unwired: 1 out]
          }
          frame True {
          }
        }
        n824 = call <vilib>:"Add State(s) to Queue__JKI_lib_State_Machine.vi"("State(s) in Front (\"\")"=w1860, "State(s) in (\"\")"=w1867) -> ("States Out"=w1866:string)  [unwired: 13 in]
      }
      frame "Queue: Create" {
        # "Template Separator\n(You can make a copy of, or modify, this frame)"
        n825 = call <vilib>:"Add State(s) to Queue__JKI_lib_State_Machine.vi"("State(s) in (\"\")"=w1875) -> ("States Out"=w1874:string)  [unwired: 14 in]
      }
      frame "Queue: Flash" {
        # "Clear queue contnet\n(clear queue content by flash it)"
        n826 = Flush Queue(queue=w1879, error in (no error)=w1876) -> (error out=w1878:errorcluster)  [unwired: 2 out]
        n827 = local write "numWFInQ"(0 ("numWFInQ")) -> ()
        n828 = call <vilib>:"Add State(s) to Queue__JKI_lib_State_Machine.vi"("State(s) in (\"\")"=w1883) -> ("States Out"=w1882:string)  [unwired: 14 in]
      }
      frame "Queue: Destory" {
        # "Destory Data Queue\nDistory data queue ref so the aquisition loop stop"
        n829 = Release Queue(queue=w1891, error in (no error)=w1886) -> (error out=w1894:errorcluster)  [unwired: 1 in, 2 out]
        n830 = Release Queue(queue=w1890, error in (no error)=w1886) -> (error out=w1893:errorcluster)  [unwired: 1 in, 2 out]
        n831 = Release Queue(queue=w1888, error in (no error)=w1886) -> (error out=w1887:errorcluster)  [unwired: 1 in, 2 out]
        n832 = Release Queue(queue=w1885, error in (no error)=w1886) -> (error out=w1884:errorcluster)  [unwired: 1 in, 2 out]
        n833 = Merge Errors(w1894, w1893, w1887, w1884) -> (w1892:errorcluster)
        n834 = call <vilib>:"Add State(s) to Queue__JKI_lib_State_Machine.vi"("State(s) in (\"\")"=w1897) -> ("States Out"=w1896:string)  [unwired: 14 in]
      }
      frame "---------- SysConfig ----------" {
        # "Template Separator\n(You can make a copy of, or modify, this frame)"
        n835 = call <vilib>:"Add State(s) to Queue__JKI_lib_State_Machine.vi"("State(s) in (\"\")"=w1902) -> ("States Out"=w1901:string)  [unwired: 14 in]
      }
      frame "SysConfig: Load APD Info" {
        # "Macro to load APD data\n(load from serial number -> load all data -> get gain limit)"
        n836 = call <vilib>:"Add State(s) to Queue__JKI_lib_State_Machine.vi"("State(s) in Front (\"\")"="APD: LoadFromSerialNoRawData\nAPD: UpdateIndicatorMacro\nAPD: GetGainLimits" ("State(s) in Front (\"\")"), "State(s) in (\"\")"=w1908) -> ("States Out"=w1907:string)  [unwired: 13 in]
      }
      frame "SysConfig: Load Digitizer Setting" {
        w1911 = enum16{"Write", "Read"}."Write" ("Operation")
        # "Digitizers in FLImDAQ is not used\nLoad DAQ config\nSave to FGV"
        # "Template Separator\n(You can make a copy of, or modify, this frame)"
        n837 = call <userlib>:"Current VIs Parent Directory__ogtk.vi"() -> ("Parent Directory (+ Relative)"=w1922:path)  [unwired: 5 in]
        n838 = Build Path(base path=w1922, name or relative path="SubVI\\DigitizerConfiguration\\V6_Scope_iRFNew.config") -> (appended path=w1923:path)
        n839 = call "ReadDigitizerConfig(SubVI).vi"("error in (no error)"=w1920, "appended path"=w1923) -> ("error out"=w1915:errorcluster, "FLImDAQ"=w1913:T4)  [unwired: 8 in]
        n840 = call "FLImDAQ_FGV.vi"("error in (no error)"=w1915, "Operation (Read)"=w1911, "Write data"=w1913) -> ("error out"=w1918:errorcluster)  [unwired: 7 in, 1 out]
        n841 = Bundle By Name(cluster=w1909, "FLImDAQ"=w1913) -> (w1910:T22)
        n842 = Unbundle By Name(w1913) -> ("Digitizer 1"=w1916:refnum<k15>, "Digitizer 2"=w1917:refnum<k15>)
        n843 = call "Digitizer1_FGV.vi"("error in (no error)"=w1918, "Operation (Read)"=w1911, "Write data"=w1916) -> ("error out"=w1919:errorcluster)  [unwired: 7 in, 1 out]
        n844 = call "Digitizer2_FGV.vi"("error in (no error)"=w1919, "Operation (Read)"=w1911, "Write data"=w1917) -> ("error out"=w1914:errorcluster)  [unwired: 7 in, 1 out]
        n845 = call <vilib>:"Add State(s) to Queue__JKI_lib_State_Machine.vi"("State(s) in (\"\")"=w1925) -> ("States Out"=w1924:string)  [unwired: 14 in]
      }
      frame "SysConfig: Load Digitizer Setting Gain" {
        w1928 = enum16{"Write", "Read"}."Write" ("Operation")
        # "Digitizers in FLImDAQ is not used\nLoad DAQ config\nSave to FGV"
        # "Template Separator\n(You can make a copy of, or modify, this frame)"
        n846 = call <userlib>:"Current VIs Parent Directory__ogtk.vi"() -> ("Parent Directory (+ Relative)"=w1939:path)  [unwired: 5 in]
        n847 = Build Path(base path=w1939, name or relative path="SubVI\\DigitizerConfiguration\\V6_Scope_Gain.config") -> (appended path=w1940:path)
        n848 = call "ReadDigitizerConfig(SubVI).vi"("error in (no error)"=w1937, "appended path"=w1940) -> ("error out"=w1932:errorcluster, "FLImDAQ"=w1930:T4)  [unwired: 8 in]
        n849 = call "FLImDAQ_FGV.vi"("error in (no error)"=w1932, "Operation (Read)"=w1928, "Write data"=w1930) -> ("error out"=w1935:errorcluster)  [unwired: 7 in, 1 out]
        n850 = Bundle By Name(cluster=w1926, "FLImDAQ"=w1930) -> (w1927:T22)
        n851 = Unbundle By Name(w1930) -> ("Digitizer 1"=w1933:refnum<k15>, "Digitizer 2"=w1934:refnum<k15>)
        n852 = call "Digitizer1_FGV.vi"("error in (no error)"=w1935, "Operation (Read)"=w1928, "Write data"=w1933) -> ("error out"=w1936:errorcluster)  [unwired: 7 in, 1 out]
        n853 = call "Digitizer2_FGV.vi"("error in (no error)"=w1936, "Operation (Read)"=w1928, "Write data"=w1934) -> ("error out"=w1931:errorcluster)  [unwired: 7 in, 1 out]
        n854 = call <vilib>:"Add State(s) to Queue__JKI_lib_State_Machine.vi"("State(s) in (\"\")"=w1942) -> ("States Out"=w1941:string)  [unwired: 14 in]
      }
      frame "SysConfig: Load LJ Pinout" {
        # "Template Separator\n(You can make a copy of, or modify, this frame)"
        n855 = call <userlib>:"Current VIs Parent Directory__ogtk.vi"() -> ("Parent Directory (+ Relative)"=w1957:path)  [unwired: 5 in]
        n856 = Build Path(base path=w1957, name or relative path="SubVI\\LabJack\\LJ_pin_setting.config") -> (appended path=w1955:path)
        n857 = call "ReadLabjackConfig(SubVI).vi"("error in (no error)"=w1953, "appended path"=w1955) -> ("error out"=w1954:errorcluster, "Utility"=w1952:T3)  [unwired: 8 in]
        n858 = Unbundle By Name(w1952) -> ("Ch1 Bias"=w1951:string, "Ch2 Bias"=w1950:string, "Ch3 Bias"=w1949:string, "Ch4 Bias"=w1943:string, "Red LED"=w1947:string, "Green LED"=w1946:string)
        n859 = global write "GlobalVariables.vi" "LED Green pin"(w1946) -> ()
        n860 = global write "GlobalVariables.vi" "LED Red pin"(w1947) -> ()
        n861 = global write "GlobalVariables.vi" "Ch1 LJ pin"(w1951) -> ()
        n862 = global write "GlobalVariables.vi" "Ch2 LJ pin"(w1950) -> ()
        n863 = global write "GlobalVariables.vi" "Ch3 LJ pin"(w1949) -> ()
        n864 = global write "GlobalVariables.vi" "Ch4 LJ pin"(w1943) -> ()
        n865 = Bundle By Name(cluster=w1944, "LJ Pinout"=w1952) -> (w1945:T22)
        n866 = call <vilib>:"Add State(s) to Queue__JKI_lib_State_Machine.vi"("State(s) in (\"\")"=w1959) -> ("States Out"=w1958:string)  [unwired: 14 in]
      }
      frame "SysConfig: Load 355 PWM" {
        # "Template Separator\n(You can make a copy of, or modify, this frame)"
        n867 = call <userlib>:"Current VIs Parent Directory__ogtk.vi"() -> ("Parent Directory (+ Relative)"=w1977:path)  [unwired: 5 in]
        n868 = Build Path(base path=w1977, name or relative path="SubVI\\LabJack\\PWM_setting_355.config") -> (appended path=w1975:path)
        n869 = call "ReadPWMConfig(SubVI).vi"("error in (no error)"=w1973, "appended path"=w1975) -> ("error out"=w1974:errorcluster, "PWM Setting"=w1972:T32)  [unwired: 8 in]
        n870 = Unbundle By Name(w1972) -> ("DIO_EF_CLOCK1_DIVISOR"=w1969:i16, "DIO_EF_CLOCK1_ROLL_VALUE"=w1968:i32)
        n871 = Multiply(x=w1969, y=w1968) -> (x*y=w1970:i32)
        n872 = Bundle By Name(cluster=w1960, "355 PWM setting"=w1972) -> (w1961:T22)
        n873 = Divide(x=80000000.0, y=w1970) -> (x/y=w1962:dbl)
        n874 = Number To Decimal String(number=w1962) -> (decimal integer string=w1967:string)  [unwired: 1 in]
        n875 = Concatenate Strings("355nm " ("string"), w1967, "Hz" ("string")) -> (w1965:string)
        n876 = local write "Laser Rep Rate"(w1962) -> ()
        n877 = property on="355nm Laser toggle" class="Bool (strict)"("Caption.Text"=w1965) -> ()  [unwired: 2 in, 2 out]
        n878 = call <vilib>:"Add State(s) to Queue__JKI_lib_State_Machine.vi"("State(s) in (\"\")"=w1979) -> ("States Out"=w1978:string)  [unwired: 14 in]
      }
      frame "SysConfig: Load AB PWM" {
        # "Load AB PWM setting\n(load setting, update AB toggle text)"
        n879 = call <userlib>:"Current VIs Parent Directory__ogtk.vi"() -> ("Parent Directory (+ Relative)"=w2002:path)  [unwired: 5 in]
        n880 = Build Path(base path=w2002, name or relative path="SubVI\\LabJack\\PWM_setting_AB.config") -> (appended path=w2000:path)
        n881 = call "ReadPWMConfig(SubVI).vi"("error in (no error)"=w1998, "appended path"=w2000) -> ("error out"=w1999:errorcluster, "PWM Setting"=w1997:T32)  [unwired: 8 in]
        n882 = Unbundle By Name(w1997) -> ("DIO_EF_CLOCK1_DIVISOR"=w1994:i16, "DIO_EF_CLOCK1_ROLL_VALUE"=w1983:i32, "DIO#_EF_CONFIG_A"=w1984:i32)
        n883 = Divide(x=w1984, y=w1983) -> (x/y=w1982:dbl)
        n884 = Multiply(x=w1994, y=w1983) -> (x*y=w1995:i32)
        n885 = Multiply(x=w1982, y=100.0) -> (x*y=w1980:dbl)
        n886 = Bundle By Name(cluster=w1985, "AB PWM setting"=w1997) -> (w1986:T22)
        n887 = Divide(x=80000000.0, y=w1995) -> (x/y=w1987:dbl)
        n888 = Number To Decimal String(number=w1987, width (-)=i16 2) -> (decimal integer string=w1993:string)
        n889 = local write "Duty Cycle (%)"(w1980) -> ()
        n890 = local write "AB Rep Rate"(w1987) -> ()
        n891 = Concatenate Strings("445nm " ("string"), w1993, "Hz " ("string")) -> (w1991:string)
        n892 = property on="Aiming beam toggle" class="Bool (strict)"("Caption.Text"=w1991) -> ()  [unwired: 2 in, 2 out]
        n893 = call <vilib>:"Add State(s) to Queue__JKI_lib_State_Machine.vi"("State(s) in (\"\")"=w2004) -> ("States Out"=w2003:string)  [unwired: 14 in]
      }
      frame "SysConfig: Load AB setting" {
        # "Template Separator\n(You can make a copy of, or modify, this frame)"
        n894 = call "readAimingBeamSetting.vi"("error in (no error)"=w2006) -> ("error out"=w2005:errorcluster, "Aiming Beam Setting"=w2007:T33)  [unwired: 9 in]
        n895 = Bundle By Name(cluster=w2008, "AB Cluster"=w2007) -> (w2009:T22)
        n896 = call <vilib>:"Add State(s) to Queue__JKI_lib_State_Machine.vi"("State(s) in (\"\")"=w2012) -> ("States Out"=w2011:string)  [unwired: 14 in]
      }
      frame "---------- SystemStatus ----------" {
        # "Template Separator\n(You can make a copy of, or modify, this frame)"
        n897 = call <vilib>:"Add State(s) to Queue__JKI_lib_State_Machine.vi"("State(s) in (\"\")"=w2017) -> ("States Out"=w2016:string)  [unwired: 14 in]
      }
      frame "SystemStatus: SlowSysStatusMacro" {
        # "store system check time"
        # "Template Separator\n(You can make a copy of, or modify, this frame)"
        n898 = Tick Count (ms)() -> (millisecond timer value=w2020:u32)
        n899 = Bundle By Name(cluster=w2018, "SlowTimer"=w2020) -> (w2019:T22)
        n900 = call <vilib>:"Add State(s) to Queue__JKI_lib_State_Machine.vi"("State(s) in Front (\"\")"="/*Digitizer: checkTemp" ("State(s) in Front (\"\")"), "State(s) in (\"\")"=w2025) -> ("States Out"=w2024:string)  [unwired: 13 in]
      }
      frame "SystemStatus: FastSysStatusMacro" {
        # "store system check time"
        # "Template Separator\n(You can make a copy of, or modify, this frame)"
        n901 = Tick Count (ms)() -> (millisecond timer value=w2028:u32)
        n902 = Bundle By Name(cluster=w2026, "FastTimer"=w2028) -> (w2027:T22)
        n903 = call <vilib>:"Add State(s) to Queue__JKI_lib_State_Machine.vi"("State(s) in Front (\"\")"="355 Laser: CheckPWMStatus\nAimingBeam: GetPWMStatus" ("State(s) in Front (\"\")"), "State(s) in (\"\")"=w2033) -> ("States Out"=w2032:string)  [unwired: 13 in]
      }
      frame "---------- UI ----------" {
        # "Do not put any code in this frame.\n(It is a separator no-op. You can make a copy of this frame to create a new UI frame)"
        n904 = call <vilib>:"Add State(s) to Queue__JKI_lib_State_Machine.vi"("State(s) in (\"\")"=w2038) -> ("States Out"=w2037:string)  [unwired: 14 in]
      }
      frame "UI: InitIRFDataTable" {
        # "Initial iRF table setup\n(Setup the table for iRF measurement, set the active cell to 1st roll)"
        n905 = while {
          tunnel: [w2063] -> w2042 mode=indexing
          shift-right: [w2063] -> _
          shift-left: 0.03 -> [w2069]
          stop <- w2064 continue-if-true
          # "Generate Gain less than 3"
          n906 = Greater Or Equal?(x=w2069, y=3.0) -> (x >= y?=w2072:bool)
          n907 = Select(t=0.1, s=w2072, f=0.3) -> (s? t:f=w2068:dbl)
          n908 = Add(x=w2068, y=w2069) -> (x+y=w2067:dbl)
          n909 = In Range and Coerce(upper limit=4.6, x=w2067, lower limit=0.05) -> (coerced(x)=w2063:dbl, In Range?=w2064:bool)
        }
        "iRFCtrlV" <- w2042
        n910 = for {
          tunnel: w2042 -> [w2062] mode=indexing
          tunnel: [w2058] -> w2041 mode=indexing
          tunnel: T19 {"Row"=0, "Column"=0} ("Active Cell:Active Cell") -> [w2053]
          i -> [w2052]
          n911 = Bundle By Name(cluster=w2053, "Row"=w2052, "Column"=0) -> (w2056:T19)
          n912 = Number To Fractional String(number=w2062, precision (6)=i16 2) -> (F-format string=w2060:string)  [unwired: 2 in]
          n913 = Equal To 0?(x=w2052) -> (x = 0?=w2051:bool)
          n914 = Select(t=u32 16773632 ("Active Cell:Cell Background Color"), s=w2051, f=u32 16448250 ("Active Cell:Cell Background Color")) -> (s? t:f=w2048:u32)
          n915 = property on="iRFDataTable" class="Tbl (strict)"("Active Cell"=w2056, "Cell BG Color"=w2048) -> ()  [unwired: 2 in, 2 out]
          n916 = Build Array(w2060, "No" ("element")) -> (w2058:string[])
          n917 = Bundle By Name(cluster=w2053, "Row"=w2052, "Column"=1) -> (w2054:T19)
          n918 = property on="iRFDataTable" class="Tbl (strict)"("Active Cell"=w2054, "Cell BG Color"=w2048) -> ()  [unwired: 2 in, 2 out]
        }
        "iRFDataTable" <- w2041
        n919 = call <vilib>:"Add State(s) to Queue__JKI_lib_State_Machine.vi"("State(s) in (\"\")"=w2047) -> ("States Out"=w2046:string)  [unwired: 14 in]
      }
      frame "UI: UpdateIRFDataTable" {
        w2076 = i32[] [0, 1]
        w2075 = T19 {"Row"=0, "Column"=0} ("Active Cell:Active Cell")
        # "Update iRF data table.\n(Change Status to yes, update table color)"
        n920 = local read "iRFDataTable"() -> (w2082:string[][])
        n921 = Unbundle By Name(w2081) -> ("iRFIdx"=w2074:i32)
        n922 = Decrement(x=w2074) -> (x-1=w2077:i32)
        n923 = Replace Array Subset(array=w2082, new element="Yes" ("new element/subarray"), index (row)=w2077, index (col)=1 ("disabled index (col)")) -> (w2078:string[][])
        n924 = for {
          tunnel: w2076 -> [w2094] mode=indexing
          tunnel: w2075 -> [w2096]
          tunnel: w2077 -> [w2095]
          # "Update cell BG color"
          n925 = Bundle By Name(cluster=w2096, "Row"=w2095, "Column"=w2094) -> (w2093:T19)
          n926 = property on="iRFDataTable" class="Tbl (strict)"("Active Cell"=w2093, "Cell BG Color"=u32 6618880 ("Active Cell:Cell Background Color")) -> ()  [unwired: 2 in, 2 out]
        }
        n927 = for {
          tunnel: w2076 -> [w2089] mode=indexing
          tunnel: w2075 -> [w2091]
          tunnel: w2074 -> [w2090]
          n928 = Bundle By Name(cluster=w2091, "Row"=w2090, "Column"=w2089) -> (w2088:T19)
          n929 = property on="iRFDataTable" class="Tbl (strict)"("Active Cell"=w2088, "Cell BG Color"=u32 16773632 ("Active Cell:Cell Background Color")) -> ()  [unwired: 2 in, 2 out]
        }
        n930 = local write "iRFDataTable"(w2078) -> ()
        n931 = call <vilib>:"Add State(s) to Queue__JKI_lib_State_Machine.vi"("State(s) in (\"\")"=w2086) -> ("States Out"=w2085:string)  [unwired: 14 in]
      }
      frame "UI: UpdateGainDataIndicators" {
        # "Update indicator for Gain data.\n(Update Arrays and tables)"
        n932 = Unbundle By Name(w2107) -> ("GainDataTemp.CtrlV"=w2098:dbl, "GainDataTemp.AUC"=w2097:dbl, "GainDataTemp.AUC Std"=w2106:dbl, "GainDataTemp.IntFactor"=w2105:dbl, "GainDataTemp.IntCorrAUC"=w2104:dbl)
        n933 = local read "Int Corr AUC"() -> (w2110:dbl[])
        n934 = Build Array(w2098, w2097, w2106, w2105, w2104) -> (w2103:dbl[])
        n935 = local read "Intensity Factor"() -> (w2113:dbl[])
        n936 = for {
          tunnel: w2103 -> [w2129] mode=indexing
          tunnel: [w2127] -> w2101 mode=indexing
          n937 = Number To Fractional String(number=w2129, precision (6)=i16 3) -> (F-format string=w2127:string)  [unwired: 2 in]
        }
        n938 = local read "AUC Std"() -> (w2116:dbl[])
        n939 = local read "AUC"() -> (w2122:dbl[])
        n940 = local read "Ctrl V"() -> (w2119:dbl[])
        n941 = Insert Into Array(array=w2122, index=0, new element=w2097) -> (→"AUC":dbl[])
        n942 = Insert Into Array(array=w2119, index=0, new element=w2098) -> (→"Ctrl V":dbl[])
        n943 = Insert Into Array(array=w2113, index=0, new element=w2105) -> (→"Intensity Factor":dbl[])
        n944 = Insert Into Array(array=w2110, index=0, new element=w2104) -> (→"Int Corr AUC":dbl[])
        n945 = Insert Into Array(array=w2116, index=0, new element=w2106) -> (→"AUC Std":dbl[])
        n946 = local read "GainDataTable"() -> (w2099:string[][])
        n947 = Insert Into Array(array=w2099, index (row)=0, new element=w2101) -> (→"GainDataTable":string[][])  [unwired: 1 in]
        n948 = call <vilib>:"Add State(s) to Queue__JKI_lib_State_Machine.vi"("State(s) in (\"\")"=w2126) -> ("States Out"=w2125:string)  [unwired: 14 in]
      }
      frame "UI: ShowDialog" {
        # "Show dialog ask user to adjust signal level\n(If OK aquire data, if abort stop auqisition)"
        n949 = local read "Task"() -> (w2130:enum32{"iRFAndGain", "Alignment"})
        n950 = case shown="\"Alignment\"" w2130 {
          tunnel: ["Please adjsut max signal level to around 1V." ("message") "Click OK to confirm data!" ("message")] -> w2136
          frame "iRFAndGain", Default {
          }
          frame "Alignment" {
          }
        }
        n951 = Two Button Dialog(message=w2136, 1:"Abort" ("F button name (\"Cancel\")"), 2:"OK" ("T button name (\"OK\")")) -> (T button?=w2133:bool)
        n952 = case shown="False" w2133 {
          tunnel: ["Macro: StopRun\nQueue: FlashDataAllQueue" ("State(s) in Front (\"\")") w2144] -> w2132
          tunnel: w2131 -> [_ w2144]
          frame False {
            # "Stop if abort"
          }
          frame True {
            # "Continue if OK"
          }
        }
        n953 = call <vilib>:"Add State(s) to Queue__JKI_lib_State_Machine.vi"("State(s) in Front (\"\")"=w2132) -> ("States Out"=w2140:string)  [unwired: 14 in]
      }
      frame "UI: WFAutoScale" {
        # "Set graph auto scale.\n(UI: WFAutoScale >> T/F)"
        n954 = Equal?(x=w2145, y="F") -> (x = y?=w2146:bool)
        n955 = Equal?(x=w2145, y="T") -> (x = y?=w2148:bool)
        n956 = case shown="True" w2148 {
          frame False {
          }
          frame True {
            n957 = property on="Waveform (no average)" class="WFGraph (strict)"("YScale.ScaleFit"=u8 2 ("Y Scale.Scale Fit")) -> ()  [unwired: 2 in, 2 out]
          }
        }
        n958 = case shown="True" w2146 {
          frame False {
          }
          frame True {
            n959 = property on="Waveform (no average)" class="WFGraph (strict)"("YScale.ScaleFit"=u8 0 ("Y Scale.Scale Fit")) -> (error out=w2156:errorcluster)  [unwired: 2 in, 1 out]
            n960 = property on="Waveform (no average)" class="WFGraph (strict)"(error in=w2156, "YScale.Maximum"=2.0 ("Y Scale.Range:Maximum")) -> (error out=w2155:errorcluster)  [unwired: 1 in, 1 out]
            n961 = property on="Waveform (no average)" class="WFGraph (strict)"(error in=w2155, "YScale.Minimum"=0.0 ("Y Scale.Range:Maximum")) -> ()  [unwired: 1 in, 2 out]
          }
        }
        n962 = call <vilib>:"Add State(s) to Queue__JKI_lib_State_Machine.vi"("State(s) in (\"\")"=w2154) -> ("States Out"=w2153:string)  [unwired: 14 in]
      }
      frame "UI: Initialize" {
        w2162 = T11."Disabled and Grayed Out" ("Disabled")
        # "Disable all button on startup"
        # "Initialize the User Interface, here.\n(this is called automatically, by the Macro: Init)"
        n963 = property on="Ctrl V" class="DigNum (strict)"("DisabledEnum"=w2162) -> ()  [unwired: 2 in, 2 out]
        n964 = property on="StopButton" class="Bool"("DisabledEnum"=w2162) -> ()  [unwired: 2 in, 2 out]
        n965 = property on="Sys Reconfig" class="Bool"("DisabledEnum"=w2162) -> ()  [unwired: 2 in, 2 out]
        n966 = property on="StartButton" class="Bool"("DisabledEnum"=w2162) -> ()  [unwired: 2 in, 2 out]
        n967 = property on="355nm Laser toggle" class="Bool (strict)"("DisabledEnum"=w2162) -> ()  [unwired: 2 in, 2 out]
        n968 = property on="Aiming beam toggle" class="Bool (strict)"("DisabledEnum"=w2162) -> ()  [unwired: 2 in, 2 out]
        n969 = property on="Ctrl V" class="DigNum (strict)"("Data Range"=T20 {"Minimum"=0.0, "Maximum"=5.5, "Increment"=0.1} ("Data Entry Limits")) -> ()  [unwired: 2 in, 2 out]
        n970 = call <vilib>:"Add State(s) to Queue__JKI_lib_State_Machine.vi"("State(s) in (\"\")"=w2167) -> ("States Out"=w2166:string)  [unwired: 14 in]
      }
      frame "UI: showDisclaimer" {
        # "Show disclamer window.\n(It is a separator no-op. You can make a copy of this frame to create a new UI frame)"
        n971 = call <vilib>:"Application Directory.vi"() -> ("Application Directory"=w2180:path)
        n972 = Build Path(base path=w2180, name or relative path="Disclamer.png") -> (appended path=w2178:path)
        n973 = property on="Disclamer" class="Pict"() -> ("Draw Area Size"=w2176:T34)  [unwired: 2 in, 2 out]
        n974 = call <vilib>:"Read PNG File.vi"("path to PNG file"=w2178) -> ("image data"=w2175:T35)  [unwired: 8 in, 2 out]
        n975 = disable-structure "Diagram Disable Structure" shown="Disabled" {
          frame Disabled {
            n976 = flat-sequence {
              frame #0 {
                n977 = call "disclaimer.vi"() -> ()  [unwired: 12 in]
              }
              frame #1 {
                n978 = Wait (ms)(milliseconds to wait=u32 250) -> ()  [unwired: 1 out]
              }
              frame #2 {
                n979 = call "SoftwareNote.vi"() -> ()  [unwired: 12 in]
              }
            }
          }
          frame Enabled {
          }
        }
        n980 = Unbundle By Name(w2175) -> ("Rectangle.right"=w2173:i16, "Rectangle.bottom"=w2171:i16)
        n981 = Unbundle By Name(w2176) -> ("Width"=w2174:u32, "Height"=w2172:u32)
        n982 = call <vilib>:"Draw Flattened Pixmap.vi"("image data"=w2175) -> ("new picture"=→"Disclamer":picture)  [unwired: 8 in]
        n983 = Divide(x=w2174, y=w2173) -> (x/y=w2170:dbl)
        n984 = Divide(x=w2172, y=w2171) -> (x/y=w2169:dbl)
        n985 = Max & Min(x=w2170, y=w2169) -> (min(x,y)=w2168:dbl)  [unwired: 1 out]
        n986 = property on="Disclamer" class="Pict"("ZoomFactor"=w2168) -> ()  [unwired: 2 in, 2 out]
        n987 = call <vilib>:"Add State(s) to Queue__JKI_lib_State_Machine.vi"("State(s) in (\"\")"=w2185) -> ("States Out"=w2184:string)  [unwired: 14 in]
      }
      frame "UI: SetButtonText" {
        # "Set button text of 355nm laser and aiming beam."
        n988 = call <vilib>:"Add State(s) to Queue__JKI_lib_State_Machine.vi"("State(s) in (\"\")"=w2191) -> ("States Out"=w2190:string)  [unwired: 14 in]
      }
      frame "UI: DuringAquisition" {
        w2192 = T11."Enabled" ("Disabled")
        w2197 = T11."Disabled and Grayed Out" ("Disabled")
        # "Do not put any code in this frame.\n(It is a separator no-op. You can make a copy of this frame to create a new UI frame)"
        n989 = property on="StopButton" class="Bool"("DisabledEnum"=w2192) -> ()  [unwired: 2 in, 2 out]
        n990 = property on="iRFSigInRange" class="Bool (strict)"("DisabledEnum"=w2192) -> ()  [unwired: 2 in, 2 out]
        n991 = property on="AcquireGain" class="Bool"("DisabledEnum"=w2192) -> ()  [unwired: 2 in, 2 out]
        n992 = property on="GainSigInRange" class="Bool (strict)"("DisabledEnum"=w2192) -> ()  [unwired: 2 in, 2 out]
        n993 = property on="AcquireIRF" class="Bool"("DisabledEnum"=w2192) -> ()  [unwired: 2 in, 2 out]
        n994 = Bundle By Name(cluster=w2195, "SysRunning?"=TRUE) -> (w2196:T22)
        n995 = property on="StartButton" class="Bool"("DisabledEnum"=w2197) -> ()  [unwired: 2 in, 2 out]
        n996 = property on="Sys Reconfig" class="Bool"("DisabledEnum"=w2197) -> ()  [unwired: 2 in, 2 out]
        n997 = property on="355nm Laser toggle" class="Bool (strict)"("DisabledEnum"=w2197) -> ()  [unwired: 2 in, 2 out]
        n998 = property on="Aiming beam toggle" class="Bool (strict)"("DisabledEnum"=w2197) -> ()  [unwired: 2 in, 2 out]
        n999 = local write "GainInstSting"("Please set control voltage and make sure data is in range.\nClick 'Acquire' button to record data." ("GainInstSting")) -> ()
        n1000 = property on="Quit" class="Bool"("DisabledEnum"=w2197) -> ()  [unwired: 2 in, 2 out]
        n1001 = local write "iRFInstSting"("1. Click 'Set CtrlV' to set APD bias voltage\n2. Click 'Acquire' button to record data." ("iRFInstSting")) -> ()
        n1002 = property on="Laser Rep Rate" class="DigNum (strict)"("DisabledEnum"=w2197) -> ()  [unwired: 2 in, 2 out]
        n1003 = property on="Channel" class="RadioBtnsControl (strict)"("DisabledEnum"=w2197) -> ()  [unwired: 2 in, 2 out]
        n1004 = property on="Task" class="RadioBtnsControl (strict)"("DisabledEnum"=w2197) -> ()  [unwired: 2 in, 2 out]
        n1005 = call <vilib>:"Add State(s) to Queue__JKI_lib_State_Machine.vi"("State(s) in (\"\")"=w2202) -> ("States Out"=w2201:string)  [unwired: 14 in]
      }
      frame "UI: ReadyForAquisition" {
        w2203 = T11."Disabled and Grayed Out" ("Disabled")
        w2209 = T11."Enabled" ("Disabled")
        # "Do not put any code in this frame.\n(It is a separator no-op. You can make a copy of this frame to create a new UI frame)"
        n1006 = local read "Channel"() -> (w2205:enum32{"Ch1", "Ch2", "Ch3", "Ch4"})
        n1007 = property on="StopButton" class="Bool"("DisabledEnum"=w2203) -> ()  [unwired: 2 in, 2 out]
        n1008 = property on="AcquireGain" class="Bool"("DisabledEnum"=w2203) -> ()  [unwired: 2 in, 2 out]
        n1009 = property on="iRFSigInRange" class="Bool (strict)"("DisabledEnum"=w2203) -> ()  [unwired: 2 in, 2 out]
        n1010 = property on="GainSigInRange" class="Bool (strict)"("DisabledEnum"=w2203) -> ()  [unwired: 2 in, 2 out]
        n1011 = property on="AcquireIRF" class="Bool"("DisabledEnum"=w2203) -> ()  [unwired: 2 in, 2 out]
        n1012 = Bundle By Name(cluster=w2207, "SysRunning?"=FALSE) -> (w2208:T22)
        n1013 = case shown="\"Ch2\"" w2205 {
          tunnel: ["To aquire gain data:\n1. Place blue Chroma slide as close as possible to the fiber port! \n2. Start data aquisition." ("GainInstSting") "To aquire gain data:\n1. Place blue Chroma slide as close as possible to the fiber port! \n2. Start data aquisition." ("GainInstSting") "To aquire gain data:\n1. Place green Chroma slide as close as possible to the fiber port! \n2. Remove Channel 3 bandpass filter!\n3. Start data aquisition." ("GainInstSting")] -> w2206
          tunnel: ["To aquire gain data:\n1. Install Thorlabs fiber stop! \n2. Start data aquisition." ("GainInstSting") "To aquire gain data:\n1. Install Thorlabs fiber stop! \n2. Start data aquisition." ("GainInstSting") "To aquire gain data:\n1. Install fiber probe!\n2. Place DASPI solution as close as possible to fiber probe.\n3. Remove Channel 3 bandpass filter. \n4. Start data aquisition." ("GainInstSting")] -> w2204
          frame "Ch1", Default {
          }
          frame "Ch2" {
          }
          frame "Ch3" {
          }
        }
        "GainInstSting" <- w2206
        "iRFInstSting" <- w2204
        n1014 = property on="StartButton" class="Bool"("DisabledEnum"=w2209) -> ()  [unwired: 2 in, 2 out]
        n1015 = property on="Sys Reconfig" class="Bool"("DisabledEnum"=w2209) -> ()  [unwired: 2 in, 2 out]
        n1016 = property on="355nm Laser toggle" class="Bool (strict)"("DisabledEnum"=w2209) -> ()  [unwired: 2 in, 2 out]
        n1017 = property on="Aiming beam toggle" class="Bool (strict)"("DisabledEnum"=w2209) -> ()  [unwired: 2 in, 2 out]
        n1018 = property on="Quit" class="Bool"("DisabledEnum"=w2209) -> ()  [unwired: 2 in, 2 out]
        n1019 = property on="Channel" class="RadioBtnsControl (strict)"("DisabledEnum"=w2209) -> ()  [unwired: 2 in, 2 out]
        n1020 = property on="Laser Rep Rate" class="DigNum (strict)"("DisabledEnum"=w2209) -> ()  [unwired: 2 in, 2 out]
        n1021 = property on="Task" class="RadioBtnsControl (strict)"("DisabledEnum"=w2209) -> ()  [unwired: 2 in, 2 out]
        n1022 = call <vilib>:"Add State(s) to Queue__JKI_lib_State_Machine.vi"("State(s) in Front (\"\")"="LED: Green" ("State(s) in Front (\"\")"), "State(s) in (\"\")"=w2215) -> ("States Out"=w2214:string)  [unwired: 13 in]
      }
      frame "UI: Update" {
        # "Do not put any code in this frame.\n(It is a separator no-op. You can make a copy of this frame to create a new UI frame)"
        n1023 = Unbundle By Name(w2229) -> ("System Status"=→"System Hardware Connection Status":T1, "IDs.RunID"=→"Run #":i8, "FLImDAQ"=→"FLImDAQ":T27, "SysRunning?"=→"System Status:":bool, "LJ Pinout"=→"LJ Pinout":T3, "IDs.BG ID"=→"BG #":i8, "IDs.Cali ID"=→"Calibration #":i8)
        n1024 = call <vilib>:"Add State(s) to Queue__JKI_lib_State_Machine.vi"("State(s) in (\"\")"=w2233) -> ("States Out"=w2232:string)  [unwired: 14 in]
      }
      frame "UI: Cursor Set" {
        # "Argument"
        # "Set and Unset Cursor Busy.\n(Usage: \"UI: Cursor Set >> Busy|Idle\")"
        n1025 = case shown="\"Idle\", Default" w2235 {
          tunnel: w2237 -> [w2242 w2244]
          tunnel: [w2241 w2243] -> w2236
          frame "Idle", Default {
            n1026 = call <vilib>:"Unset Busy.vi"("error in (no error)"=w2242) -> ("error out"=w2241:errorcluster)  [unwired: 10 in]
          }
          frame "Busy" {
            n1027 = call <vilib>:"Set Busy.vi"("error in (no error)"=w2244) -> ("error out"=w2243:errorcluster)  [unwired: 9 in, 1 out]
          }
        }
        n1028 = call <vilib>:"Add State(s) to Queue__JKI_lib_State_Machine.vi"("State(s) in (\"\")"=w2240) -> ("States Out"=w2239:string)  [unwired: 14 in]
      }
      frame "UI: Front Panel State" {
        # "Argument"
        # "Set Front Panel Open or Closed\n(Usage: \"UI: Front Panel State >> Open|Close\")"
        n1029 = Unbundle By Name(w2245) -> ("Core.Current VI Reference"=w2248:refnum<vi>)
        n1030 = case shown="\"Open\", \"Standard\", Default" w2247 {
          tunnel: w2250 -> [w2258 w2271 w2282 w2294 w2306]
          tunnel: [w2259 w2272 w2283 w2295 w2307] -> w2249
          tunnel: w2248 -> [_ _ _ _ _]
          frame "Open", "Standard", Default {
            w2253 = T14."Standard" ("State")
            n1031 = property on="Property Node" class="VI"(error in=w2258) -> (reference out=w2256:refnum<vi>, error out=w2257:errorcluster, "FP.State"=w2255:T14)  [unwired: 1 in]
            n1032 = Not Equal?(x=w2255, y=w2253) -> (x != y?=w2254:bool)
            n1033 = case shown="True" w2254 {
              tunnel: [w2263 w2265] -> w2259
              tunnel: w2257 -> [w2262 w2265]
              tunnel: w2256 -> [w2261 _]
              tunnel: w2253 -> [w2260 _]
              frame True {
                n1034 = invoke on="Invoke Node" class="VI" method="FP.Open"(reference=w2261, error in=w2262, "Activate"=TRUE, "State"=w2260) -> (error out=w2263:errorcluster)  [unwired: 1 in, 4 out]
              }
              frame False {
              }
            }
          }
          frame "Close", "Closed" {
            n1035 = property on="Property Node" class="VI"(error in=w2271) -> (reference out=w2269:refnum<vi>, error out=w2270:errorcluster, "FP.State"=w2267:T14)  [unwired: 1 in]
            n1036 = Not Equal?(x=w2267, y=T14."Closed" ("Front Panel Window:State")) -> (x != y?=w2266:bool)
            n1037 = case shown="True" w2266 {
              tunnel: [w2273 w2276] -> w2272
              tunnel: w2270 -> [w2273 w2275]
              tunnel: w2269 -> [_ w2274]
              frame False {
              }
              frame True {
                n1038 = invoke on="Invoke Node" class="VI" method="FP.Close"(reference=w2274, error in=w2275) -> (error out=w2276:errorcluster)  [unwired: 1 in, 2 out]
              }
            }
          }
          frame "Hidden", "Hide" {
            w2277 = T14."Hidden" ("State")
            n1039 = property on="Property Node" class="VI"(error in=w2282) -> (reference out=w2280:refnum<vi>, error out=w2281:errorcluster, "FP.State"=w2279:T14)  [unwired: 1 in]
            n1040 = Not Equal?(x=w2279, y=w2277) -> (x != y?=w2278:bool)
            n1041 = case shown="True" w2278 {
              tunnel: [w2287 w2288] -> w2283
              tunnel: w2281 -> [w2286 w2288]
              tunnel: w2280 -> [w2285 _]
              tunnel: w2277 -> [w2284 _]
              frame True {
                n1042 = invoke on="Invoke Node" class="VI" method="FP.Open"(reference=w2285, error in=w2286, "State"=w2284) -> (error out=w2287:errorcluster)  [unwired: 2 in, 4 out]
              }
              frame False {
              }
            }
          }
          frame "Minimize", "Minimized" {
            w2289 = T14."Minimized" ("State")
            n1043 = property on="Property Node" class="VI"(error in=w2294) -> (reference out=w2292:refnum<vi>, error out=w2293:errorcluster, "FP.State"=w2291:T14)  [unwired: 1 in]
            n1044 = Not Equal?(x=w2291, y=w2289) -> (x != y?=w2290:bool)
            n1045 = case shown="True" w2290 {
              tunnel: [w2299 w2300] -> w2295
              tunnel: w2293 -> [w2298 w2300]
              tunnel: w2292 -> [w2297 _]
              tunnel: w2289 -> [w2296 _]
              frame True {
                n1046 = invoke on="Invoke Node" class="VI" method="FP.Open"(reference=w2297, error in=w2298, "State"=w2296) -> (error out=w2299:errorcluster)  [unwired: 2 in, 4 out]
              }
              frame False {
              }
            }
          }
          frame "Maximize", "Maximized" {
            w2301 = T14."Maximized" ("State")
            n1047 = property on="Property Node" class="VI"(error in=w2306) -> (reference out=w2304:refnum<vi>, error out=w2305:errorcluster, "FP.State"=w2303:T14)  [unwired: 1 in]
            n1048 = Not Equal?(x=w2303, y=w2301) -> (x != y?=w2302:bool)
            n1049 = case shown="True" w2302 {
              tunnel: [w2311 w2312] -> w2307
              tunnel: w2305 -> [w2310 w2312]
              tunnel: w2304 -> [w2309 _]
              tunnel: w2301 -> [w2308 _]
              frame True {
                n1050 = invoke on="Invoke Node" class="VI" method="FP.Open"(reference=w2309, error in=w2310, "State"=w2308) -> (error out=w2311:errorcluster)  [unwired: 2 in, 4 out]
              }
              frame False {
              }
            }
          }
        }
        n1051 = call <vilib>:"Add State(s) to Queue__JKI_lib_State_Machine.vi"("State(s) in (\"\")"=w2252) -> ("States Out"=w2251:string)  [unwired: 14 in]
      }
      frame "---------- 355 Laser ----------" {
        # "Template Separator\n(You can make a copy of, or modify, this frame)"
        n1052 = call <vilib>:"Add State(s) to Queue__JKI_lib_State_Machine.vi"("State(s) in (\"\")"=w2317) -> ("States Out"=w2316:string)  [unwired: 14 in]
      }
      frame "355 Laser: Check Dewelling" {
        # "if time laser start time is less than 7.5s before, wait 250ms then check again."
        # "Check laser timer\n(Check laser timer, make sure enough time lapsed after laser enable)"
        n1053 = Unbundle By Name(w2319) -> ("Laser start tic"=w2318:u32)
        n1054 = Tick Count (ms)() -> (millisecond timer value=w2324:u32)
        n1055 = Subtract(x=w2324, y=w2318) -> (x-y=w2323:u32)
        n1056 = Greater?(x=w2323, y=u32 5000) -> (0:w2321:bool)
        n1057 = case shown="False" w2321 {
          tunnel: ["355 Laser: Check Dewelling" ""] -> w2320
          frame False {
            n1058 = Wait (ms)(milliseconds to wait=u32 500) -> ()  [unwired: 1 out]
          }
          frame True {
          }
        }
        n1059 = call <vilib>:"Add State(s) to Queue__JKI_lib_State_Machine.vi"("State(s) in Front (\"\")"=w2320, "State(s) in (\"\")"=w2328) -> ("States Out"=w2327:string)  [unwired: 13 in]
      }
      frame "355 Laser: Laser enable" {
        # "Laser enable/disable\n(Usage: \"LabJack: Laser enable/disable >> 1|0\")"
        n1060 = Unbundle By Name(w2333) -> ("LJ Pinout.Laser Start/Stop"=w2339:string, "System Status.355 Laser"=w2332:bool)
        n1061 = case shown="False" w2332 {
          tunnel: w2335 -> [w2354 w2355]
          tunnel: w2339 -> [w2342 _]
          tunnel: [w2344 w2355] -> w2337
          tunnel: [w2343 u32 0 ("millisecond timer value")] -> w2336
          frame False {
            n1062 = call "LabJack_FGV.vi"("Operation(Read)"=enum16{"Write", "Read"}."Read" ("Operation")) -> ("Read data"=w2350:i32)  [unwired: 9 in, 1 out]
            n1063 = call "LJM_eWriteName.vi"("Handle In"=w2350, "Name"=w2342, "Value"=1.0, "error in"=w2354) -> ("Handle Out"=w2349:i32, "error out"=w2348:errorcluster)  [unwired: 10 in]
            n1064 = call <userlib>:"Wait (ms)__ogtk.vi"("error in (no error)"=w2348, "milliseconds to wait"=u32 250) -> ("error out"=w2347:errorcluster)  [unwired: 8 in, 1 out]
            n1065 = call "LJM_eWriteName.vi"("Handle In"=w2349, "Name"=w2342, "Value"=0.0, "error in"=w2347) -> ("error out"=w2345:errorcluster)  [unwired: 10 in, 1 out]
            n1066 = call <userlib>:"Tick Count (ms)__ogtk.vi"("error in (no error)"=w2345) -> ("error out"=w2344:errorcluster, "millisecond timer value"=w2343:u32)  [unwired: 9 in]
          }
          frame True {
          }
        }
        n1067 = Bundle By Name(cluster=w2333, "Laser start tic"=w2336) -> (w2334:T22)
        n1068 = call <vilib>:"Add State(s) to Queue__JKI_lib_State_Machine.vi"("State(s) in (\"\")"=w2341) -> ("States Out"=w2340:string)  [unwired: 14 in]
      }
      frame "355 Laser: Laser disable" {
        # "Laser enable/disable\n(Usage: \"LabJack: Laser enable/disable >> 1|0\")"
        n1069 = Unbundle By Name(w2358) -> ("LJ Pinout.Laser Start/Stop"=w2363:string, "System Status.355 Laser"=w2357:bool)
        n1070 = case shown="True" w2357 {
          tunnel: w2364 -> [w2367 w2381]
          tunnel: w2363 -> [_ w2369]
          tunnel: [w2367 w2371] -> w2361
          tunnel: [u32 0 ("millisecond timer value") w2370] -> w2360
          frame False {
          }
          frame True {
            n1071 = call "LabJack_FGV.vi"("Operation(Read)"=enum16{"Write", "Read"}."Read" ("Operation")) -> ("Read data"=w2377:i32)  [unwired: 9 in, 1 out]
            n1072 = call "LJM_eWriteName.vi"("Handle In"=w2377, "Name"=w2369, "Value"=1.0, "error in"=w2381) -> ("Handle Out"=w2376:i32, "error out"=w2375:errorcluster)  [unwired: 10 in]
            n1073 = call <userlib>:"Wait (ms)__ogtk.vi"("error in (no error)"=w2375, "milliseconds to wait"=u32 250) -> ("error out"=w2374:errorcluster)  [unwired: 8 in, 1 out]
            n1074 = call "LJM_eWriteName.vi"("Handle In"=w2376, "Name"=w2369, "Value"=0.0, "error in"=w2374) -> ("error out"=w2372:errorcluster)  [unwired: 10 in, 1 out]
            n1075 = call <userlib>:"Tick Count (ms)__ogtk.vi"("error in (no error)"=w2372) -> ("error out"=w2371:errorcluster, "millisecond timer value"=w2370:u32)  [unwired: 9 in]
          }
        }
        n1076 = Bundle By Name(cluster=w2358, "Laser start tic"=w2360) -> (w2359:T22)
        n1077 = call <vilib>:"Add State(s) to Queue__JKI_lib_State_Machine.vi"("State(s) in (\"\")"=w2366) -> ("States Out"=w2365:string)  [unwired: 14 in]
      }
      frame "355 Laser: Dewelling" {
        # "Wait some time (ms)\n(355 Laser: Dewelling >> #)"
        n1078 = Fract/Exp String To Number(string=w2385, default (0 dbl)=0) -> (number=w2383:i32)  [unwired: 2 in, 1 out]
        n1079 = Wait (ms)(milliseconds to wait=w2383) -> ()  [unwired: 1 out]
        n1080 = call <vilib>:"Add State(s) to Queue__JKI_lib_State_Machine.vi"("State(s) in (\"\")"=w2389) -> ("States Out"=w2388:string)  [unwired: 14 in]
      }
      frame "355 Laser: Init" {
        # "Initilize 355nm laser\n(Start laser, enable interlock)"
        n1081 = call <vilib>:"Add State(s) to Queue__JKI_lib_State_Machine.vi"("State(s) in Front (\"\")"="355 Laser: CheckControllerStatus", "State(s) in (\"\")"=w2395) -> ("States Out"=w2394:string)  [unwired: 13 in]
      }
      frame "355 Laser: Close" {
        # "Template Separator\n(You can make a copy of, or modify, this frame)"
        n1082 = call <vilib>:"Add State(s) to Queue__JKI_lib_State_Machine.vi"("State(s) in Front (\"\")"="355 Laser: CheckControllerStatus\n355 Laser: Laser disable\n355 Laser: Dewelling >>1000", "State(s) in (\"\")"=w2401) -> ("States Out"=w2400:string)  [unwired: 13 in]
      }
      frame "355 Laser: CheckControllerStatus" {
        # "if average < 1, laser on\nif average > 9, laser off\nif 1<average<9, interlock open, blink indicator"
        # "take 10 measuremt and look at average"
        # "Check 355 laser controller status\nBy probing Emisison Lamp negative terminal voltage"
        n1083 = Unbundle By Name(w2402) -> ("LJ Pinout.Laser Ready"=w2412:string)
        n1084 = call "LabJack_FGV.vi"("Operation(Read)"=enum16{"Write", "Read"}."Read" ("Operation")) -> ("Read data"=w2413:i32)  [unwired: 9 in, 1 out]
        n1085 = for {
          N: 10 -> [_]
          tunnel: w2413 -> [w2447]
          tunnel: w2412 -> [w2442]
          shift-right: [w2446] -> w2406
          shift-left: w2411 -> [w2445]
          tunnel: [w2443] -> w2404 mode=indexing
          n1086 = call "LJM_eReadName.vi"("Handle In"=w2447, "Name"=w2442, "error in"=w2445) -> ("Value"=w2443:dbl, "error out"=w2446:errorcluster)  [unwired: 10 in, 1 out]
          n1087 = Wait (ms)(milliseconds to wait=u32 50) -> ()  [unwired: 1 out]
        }
        n1088 = case shown="No Error" w2406 {
          selector: w2406 -> [w2421 w2440]
          tunnel: [w2423 FALSE] -> w2408
          tunnel: [w2422 w2440] -> w2407
          tunnel: [w2417 nan] -> w2405
          tunnel: w2404 -> [w2419 _]
          frame No Error {
            n1089 = call-poly <vilib>:"Mean.vi"("X"=w2419) -> ("mean"=w2417:dbl)  [unwired: 1 out]
            n1090 = Less?(x=w2417, y=9.3) -> (x < y?=w2418:bool)
            n1091 = case shown="False" w2418 {
              tunnel: [w2426 TRUE] -> w2423
              tunnel: w2417 -> [w2429 _]
              tunnel: w2421 -> [w2425 w2436]
              tunnel: [w2424 w2436] -> w2422
              frame False {
                n1092 = Greater?(x=w2429, y=10.0) -> (0:w2427:bool)
                n1093 = case shown="True" w2427 {
                  tunnel: [FALSE FALSE] -> w2426
                  tunnel: w2425 -> [_ w2433]
                  tunnel: [errorcluster {"status"=TRUE, "code"=5002, "source"="355 Laser"} ("error out") w2433] -> w2424
                  frame False {
                    n1094 = property on="355 Laser" class="Bool (strict)"("Blinking"=FALSE) -> ()  [unwired: 2 in, 2 out]
                  }
                  frame True {
                    n1095 = property on="355 Laser" class="Bool (strict)"("Blinking"=FALSE) -> ()  [unwired: 2 in, 2 out]
                  }
                }
              }
              frame True {
                n1096 = property on="355 Laser" class="Bool (strict)"("Blinking"=FALSE) -> ()  [unwired: 2 in, 2 out]
              }
            }
          }
          frame Error {
          }
        }
        "laser EM lamp V" <- w2405
        n1097 = Bundle By Name(cluster=w2402, "System Status.355 Laser"=w2408) -> (w2403:T22)
        n1098 = call <vilib>:"Add State(s) to Queue__JKI_lib_State_Machine.vi"("State(s) in (\"\")"=w2416) -> ("States Out"=w2415:string)  [unwired: 14 in]
      }
      frame "355 Laser: CheckPWMStatus" {
        # "Check 355 laser PWM status\n(Read LJ DIO#EF_ENABLE register to determine PWM status)"
        n1099 = Unbundle By Name(w2448) -> ("LJ Pinout.355 PWM"=w2449:string)
        n1100 = call "LabJack_FGV.vi"("Operation(Read)"=enum16{"Write", "Read"}."Read" ("Operation"), "error in (no error)"=w2452) -> ("error out"=w2455:errorcluster, "Read data"=w2456:i32)  [unwired: 8 in]
        n1101 = Concatenate Strings(w2449, "_EF_ENABLE" ("string")) -> (w2454:string)
        n1102 = call "LJM_eReadName.vi"("Handle In"=w2456, "Name"=w2454, "error in"=w2455) -> ("Value"=w2451:dbl, "error out"=w2453:errorcluster)  [unwired: 10 in, 1 out]
        n1103 = Greater Than 0?(x=w2451) -> (x > 0?=w2450:bool)
        n1104 = case shown="False" w2450 {
          frame False {
            # "PWM is off\nset color to gray"
            n1105 = local write "355nm Laser toggle"(FALSE ("355nm Laser")) -> ()
          }
          frame True {
            # "PWM is on\nset color to light green"
            n1106 = local write "355nm Laser toggle"(TRUE ("355nm Laser")) -> ()
          }
        }
        n1107 = call <vilib>:"Add State(s) to Queue__JKI_lib_State_Machine.vi"("State(s) in (\"\")"=w2461) -> ("States Out"=w2460:string)  [unwired: 14 in]
      }
      frame "355 Laser: Start" {
        # "Template Separator\n(You can make a copy of, or modify, this frame)"
        n1108 = call <vilib>:"Add State(s) to Queue__JKI_lib_State_Machine.vi"("State(s) in Front (\"\")"="LabJack: 355_PWM_Start", "State(s) in (\"\")"=w2469) -> ("States Out"=w2468:string)  [unwired: 13 in]
      }
      frame "355 Laser: Stop" {
        # "Template Separator\n(You can make a copy of, or modify, this frame)"
        n1109 = call <vilib>:"Add State(s) to Queue__JKI_lib_State_Machine.vi"("State(s) in Front (\"\")"="LabJack: 355_PWM_Stop", "State(s) in (\"\")"=w2475) -> ("States Out"=w2474:string)  [unwired: 13 in]
      }
      frame "---------- Utility ----------" {
        # "Template Separator\n(You can make a copy of, or modify, this frame)"
        n1110 = call <vilib>:"Add State(s) to Queue__JKI_lib_State_Machine.vi"("State(s) in (\"\")"=w2480) -> ("States Out"=w2479:string)  [unwired: 14 in]
      }
      frame "Utility: EnableGain?" {
        # "Enable or disable control V numeric control\n(Utility: EnableGain? >> True|False)"
        n1111 = case shown="\"True\", Default" w2481 {
          frame "False" {
            n1112 = property on="Ctrl V" class="DigNum (strict)"("DisabledEnum"=T11."Disabled and Grayed Out" ("Disabled")) -> ()  [unwired: 2 in, 2 out]
          }
          frame "True", Default {
            n1113 = property on="Ctrl V" class="DigNum (strict)"("DisabledEnum"=T11."Enabled" ("Disabled")) -> ()  [unwired: 2 in, 2 out]
          }
        }
        n1114 = call <vilib>:"Add State(s) to Queue__JKI_lib_State_Machine.vi"("State(s) in (\"\")"=w2486) -> ("States Out"=w2485:string)  [unwired: 14 in]
      }
      frame "Utility: SetDefaultMaxV" {
        # "Template Separator\n(You can make a copy of, or modify, this frame)"
        n1115 = local read "Ch1 Max CtrlV"() -> (w2489:dbl)
        n1116 = local write "Gain High"(w2489) -> ()
        n1117 = call <vilib>:"Add State(s) to Queue__JKI_lib_State_Machine.vi"("State(s) in (\"\")"=w2494) -> ("States Out"=w2493:string)  [unwired: 14 in]
      }
      frame "Utility: setSaveFlag" {
        # "Template Separator\n(You can make a copy of, or modify, this frame)"
        n1118 = Fract/Exp String To Number(string=w2495, default (0 dbl)=u8 0) -> (number=w2497:u8)  [unwired: 2 in, 1 out]
        n1119 = case shown="0, Default" w2497 {
          tunnel: [FALSE TRUE] -> w2496
          frame 0, Default {
          }
          frame 1 {
          }
        }
        n1120 = local write "SaveData?"(w2496) -> ()
        n1121 = call <vilib>:"Add State(s) to Queue__JKI_lib_State_Machine.vi"("State(s) in (\"\")"=w2503) -> ("States Out"=w2502:string)  [unwired: 14 in]
      }
      frame "Utility: Dewelling" {
        # "Main loop dewell\n(Dewelling >> #)"
        n1122 = Fract/Exp String To Number(string=w2508, default (0 dbl)=0) -> (number=w2506:i32)  [unwired: 2 in, 1 out]
        n1123 = Wait (ms)(milliseconds to wait=w2506) -> ()  [unwired: 1 out]
        n1124 = call <vilib>:"Add State(s) to Queue__JKI_lib_State_Machine.vi"("State(s) in (\"\")"=w2513) -> ("States Out"=w2512:string)  [unwired: 14 in]
      }
      frame "Utility: SetAllChanManualGain" {
        # "Template Separator\n(You can make a copy of, or modify, this frame)"
        n1125 = property on="Auto gain" class="Bool (strict)"("Val(Sgnl)"=FALSE ("Value (Signaling)")) -> ()  [unwired: 2 in, 2 out]
        n1126 = call <vilib>:"Add State(s) to Queue__JKI_lib_State_Machine.vi"("State(s) in (\"\")"=w2519) -> ("States Out"=w2518:string)  [unwired: 14 in]
      }
      frame "Utility: SetAllChanAutoGain" {
        # "Template Separator\n(You can make a copy of, or modify, this frame)"
        n1127 = property on="Auto gain" class="Bool (strict)"("Val(Sgnl)"=TRUE ("Value (Signaling)")) -> ()  [unwired: 2 in, 2 out]
        n1128 = call <vilib>:"Add State(s) to Queue__JKI_lib_State_Machine.vi"("State(s) in (\"\")"=w2525) -> ("States Out"=w2524:string)  [unwired: 14 in]
      }
      frame "---------- Graph ----------" {
        # "Template Separator\n(You can make a copy of, or modify, this frame)"
        n1129 = call <vilib>:"Add State(s) to Queue__JKI_lib_State_Machine.vi"("State(s) in (\"\")"=w2530) -> ("States Out"=w2529:string)  [unwired: 14 in]
      }
      frame "Graph: ClearHistory" {
        # "Clear intensity trace history\n(You can make a copy of, or modify, this frame)"
        n1130 = property on="Waveform Chart" class="WFChart (strict)"("History Data"=dbl[] []) -> ()  [unwired: 2 in, 2 out]
        n1131 = call <vilib>:"Add State(s) to Queue__JKI_lib_State_Machine.vi"("State(s) in (\"\")"=w2536) -> ("States Out"=w2535:string)  [unwired: 14 in]
      }
      frame "Graph: SetXScale" {
        # "Set X scale multiplier\n(Check digitizer aquisition speed and update x scale)"
        n1132 = local read "Channel"() -> (w2541:enum32{"Ch1", "Ch2", "Ch3", "Ch4"})
        n1133 = case shown="\"Ch1\", \"Ch2\", Default" w2541 {
          tunnel: w2540 -> [w2552 w2555]
          tunnel: [w2551 w2553] -> w2539
          tunnel: [w2550 w2554] -> w2538
          frame "Ch1", "Ch2", Default {
            n1134 = call "Digitizer1_FGV.vi"("error in (no error)"=w2552) -> ("error out"=w2551:errorcluster, "Read data"=w2550:refnum<k15>)  [unwired: 9 in]
          }
          frame "Ch3" {
            n1135 = call "Digitizer2_FGV.vi"("error in (no error)"=w2555) -> ("error out"=w2553:errorcluster, "Read data"=w2554:refnum<k15>)  [unwired: 9 in]
          }
        }
        n1136 = property on="Property Node" class="niScope"(reference=w2538, error in=w2539) -> (error out=w2543:errorcluster, "Min Sample Rate"=w2545:dbl)  [unwired: 1 out]
        n1137 = Divide(x=1.0, y=w2545) -> (x/y=w2544:dbl)
        "dt (s)" <- w2544
        n1138 = property on="Waveform (no average)" class="WFGraph (strict)"(error in=w2543, "XScale.Multiplier"=w2544) -> (error out=w2542:errorcluster)  [unwired: 1 in, 1 out]
        n1139 = call <vilib>:"Add State(s) to Queue__JKI_lib_State_Machine.vi"("State(s) in (\"\")"=w2549) -> ("States Out"=w2548:string)  [unwired: 14 in]
      }
      frame "Graph: AddCursors" {
        # "Add BG and DC cursor to all graphs\n(You can make a copy of, or modify, this frame)"
        n1140 = property on="Waveform (no average)" class="WFGraph (strict)"(error in=w2577) -> ("CrsrList"=w2563:T36, "XScale.Maximum"=w2571:dbl)  [unwired: 1 in, 2 out]
        n1141 = Multiply(x=w2571, y=0.05) -> (x*y=w2574:dbl)
        n1142 = Multiply(x=w2571, y=0.4) -> (x*y=w2567:dbl)
        n1143 = Multiply(x=w2571, y=0.2) -> (x*y=w2569:dbl)
        n1144 = Multiply(x=w2571, y=0.65) -> (x*y=w2566:dbl)
        n1145 = Build Array(w2574, w2569, w2567, w2566) -> (w2568:dbl[])
        n1146 = Index Array(array=w2563, index=4) -> (element=w2561:T37)
        n1147 = for {
          N: 4 -> [_]
          tunnel: w2563 -> [w2587] mode=indexing
          tunnel: w2568 -> [w2585] mode=indexing
          tunnel: [w2586] -> w2558 mode=indexing
          tunnel: u32[] [6618880, 6618880, 16711680, 16711680] -> [w2584] mode=indexing
          n1148 = Bundle By Name(cluster=w2587, "Position.X"=w2585, "Color"=w2584) -> (w2586:T37)
        }
        n1149 = Bundle By Name(cluster=w2561, "Position.Y"=0.0, "Color"=u32 6618880) -> (w2557:T37)
        n1150 = Build Array (concatenate)(w2558, w2557) -> (w2556:T38)
        n1151 = control-ref of="Waveform (no average)"() -> (w2565:refnum<vi>)
        n1152 = property on="Waveform (no average)" class="WFGraph (strict)"("CrsrList"=w2556) -> (error out=w2576:errorcluster)  [unwired: 2 in, 1 out]
        n1153 = call "UpdateCurserIdx(SubVI).vi"("error in (no error)"=w2576, "WaveformGraph in"=w2565) -> ("error out"=w2578:errorcluster)  [unwired: 9 in]
        n1154 = call <vilib>:"Add State(s) to Queue__JKI_lib_State_Machine.vi"("State(s) in (\"\")"=w2583) -> ("States Out"=w2582:string)  [unwired: 14 in]
      }
      frame "---------- APD ----------" {
        # "Template Separator\n(You can make a copy of, or modify, this frame)"
        n1155 = call <vilib>:"Add State(s) to Queue__JKI_lib_State_Machine.vi"("State(s) in (\"\")"=w2592) -> ("States Out"=w2591:string)  [unwired: 14 in]
      }
      frame "APD: Initialize" {
        w2593 = enum16{"Read", "Write"}."Write" ("Operation (Read)")
        w2596 = refnum<class "APDClass.lvclass"> refnum  # APDClass.lvclass
        # "Initialize APD FVG\n(You can make a copy of, or modify, this frame)"
        n1156 = call "APD2FGV.vi"("Error In"=w2595, "Operation (Read)"=w2593, "APDClass in"=w2596) -> ("Error Out"=w2597:errorcluster)  [unwired: 7 in, 1 out]
        n1157 = call "APD1FGV.vi"("Error In"=w2595, "Operation (Read)"=w2593, "APDClass in"=w2596) -> ("Error Out"=w2598:errorcluster)  [unwired: 7 in, 1 out]
        n1158 = call "APD4FGV.vi"("Error In"=w2595, "Operation (Read)"=w2593, "APDClass in"=w2596) -> ("Error Out"=w2594:errorcluster)  [unwired: 7 in, 1 out]
        n1159 = call "APD3FGV.vi"("Error In"=w2595, "Operation (Read)"=w2593, "APDClass in"=w2596) -> ("Error Out"=w2600:errorcluster)  [unwired: 7 in, 1 out]
        n1160 = Merge Errors(w2598, w2597, w2600, w2594) -> (w2599:errorcluster)
        n1161 = call <vilib>:"Add State(s) to Queue__JKI_lib_State_Machine.vi"("State(s) in (\"\")"=w2604) -> ("States Out"=w2603:string)  [unwired: 14 in]
      }
      frame "APD: LoadFromSerial" {
        w2606 = enum16{"Read", "Write"}."Write" ("Operation (Read)")
        # "Load APD info based on serial numbers\n(update FGV)"
        n1162 = call "readAPDSerial.vi"("Error In"=w2611) -> ("Error Out"=w2609:errorcluster, "output cluster"=w2612:T39)  [unwired: 9 in]
        n1163 = Unbundle By Name(w2612) -> ("Ch1APDSerial#"=w2624:string, "Ch2APDSerial#"=w2622:string, "Ch3APDSerial#"=w2619:string, "Ch4APDSerial#"=w2610:string)
        n1164 = call "CreatFromSerialNum.vi"("error in (no error)"=w2609, "APD Serial #"=w2624) -> ("error out"=w2613:errorcluster, "APDClass out"=w2623:refnum<class "APDClass.lvclass">)  [unwired: 8 in]
        n1165 = call "CreatFromSerialNum.vi"("error in (no error)"=w2609, "APD Serial #"=w2622) -> ("error out"=w2621:errorcluster, "APDClass out"=w2617:refnum<class "APDClass.lvclass">)  [unwired: 8 in]
        n1166 = call "CreatFromSerialNum.vi"("error in (no error)"=w2609, "APD Serial #"=w2619) -> ("error out"=w2620:errorcluster, "APDClass out"=w2618:refnum<class "APDClass.lvclass">)  [unwired: 8 in]
        n1167 = call "CreatFromSerialNum.vi"("error in (no error)"=w2609, "APD Serial #"=w2610) -> ("error out"=w2607:errorcluster, "APDClass out"=w2608:refnum<class "APDClass.lvclass">)  [unwired: 8 in]
        n1168 = call "APD1FGV.vi"("Error In"=w2613, "Operation (Read)"=w2606, "APDClass in"=w2623) -> ("Error Out"=w2625:errorcluster)  [unwired: 7 in, 1 out]
        n1169 = call "APD2FGV.vi"("Error In"=w2621, "Operation (Read)"=w2606, "APDClass in"=w2617) -> ("Error Out"=w2626:errorcluster)  [unwired: 7 in, 1 out]
        n1170 = call "APD3FGV.vi"("Error In"=w2620, "Operation (Read)"=w2606, "APDClass in"=w2618) -> ("Error Out"=w2627:errorcluster)  [unwired: 7 in, 1 out]
        n1171 = call "APD4FGV.vi"("Error In"=w2607, "Operation (Read)"=w2606, "APDClass in"=w2608) -> ("Error Out"=w2605:errorcluster)  [unwired: 7 in, 1 out]
        n1172 = Merge Errors(w2625, w2626, w2627, w2605) -> (w2614:errorcluster)
        n1173 = Bundle By Name(cluster=w2615, "APDSerials"=w2612) -> (w2616:T22)
        n1174 = call <vilib>:"Add State(s) to Queue__JKI_lib_State_Machine.vi"("State(s) in (\"\")"=w2630) -> ("States Out"=w2629:string)  [unwired: 14 in]
      }
      frame "APD: LoadFromSerialNoRawData" {
        w2634 = enum16{"Read", "Write"}."Write" ("Operation (Read)")
        # "Load APD info based on serial numbers\n(update FGV)"
        n1175 = call "readAPDSerial.vi"("Error In"=w2638) -> ("Error Out"=w2636:errorcluster, "output cluster"=w2639:T39)  [unwired: 9 in]
        n1176 = Unbundle By Name(w2639) -> ("Ch1APDSerial#"=w2650:string, "Ch2APDSerial#"=w2648:string, "Ch3APDSerial#"=w2637:string, "Ch4APDSerial#"=w2631:string)
        n1177 = call "CreatFromSerialNumNoRaw.vi"("error in (no error)"=w2636, "APD Serial #"=w2650) -> ("error out"=w2640:errorcluster, "APDClass out"=w2649:refnum<class "APDClass.lvclass">)  [unwired: 8 in]
        n1178 = call "CreatFromSerialNumNoRaw.vi"("error in (no error)"=w2636, "APD Serial #"=w2648) -> ("error out"=w2647:errorcluster, "APDClass out"=w2644:refnum<class "APDClass.lvclass">)  [unwired: 8 in]
        n1179 = call "CreatFromSerialNumNoRaw.vi"("error in (no error)"=w2636, "APD Serial #"=w2637) -> ("error out"=w2646:errorcluster, "APDClass out"=w2645:refnum<class "APDClass.lvclass">)  [unwired: 8 in]
        n1180 = call "CreatFromSerialNumNoRaw.vi"("error in (no error)"=w2636, "APD Serial #"=w2631) -> ("error out"=w2633:errorcluster, "APDClass out"=w2635:refnum<class "APDClass.lvclass">)  [unwired: 8 in]
        n1181 = call "APD1FGV.vi"("Error In"=w2640, "Operation (Read)"=w2634, "APDClass in"=w2649) -> ("Error Out"=w2651:errorcluster)  [unwired: 7 in, 1 out]
        n1182 = call "APD2FGV.vi"("Error In"=w2647, "Operation (Read)"=w2634, "APDClass in"=w2644) -> ("Error Out"=w2652:errorcluster)  [unwired: 7 in, 1 out]
        n1183 = call "APD3FGV.vi"("Error In"=w2646, "Operation (Read)"=w2634, "APDClass in"=w2645) -> ("Error Out"=w2653:errorcluster)  [unwired: 7 in, 1 out]
        n1184 = call "APD4FGV.vi"("Error In"=w2633, "Operation (Read)"=w2634, "APDClass in"=w2635) -> ("Error Out"=w2632:errorcluster)  [unwired: 7 in, 1 out]
        n1185 = Merge Errors(w2651, w2652, w2653, w2632) -> (w2641:errorcluster)
        n1186 = Bundle By Name(cluster=w2642, "APDSerials"=w2639) -> (w2643:T22)
        n1187 = call <vilib>:"Add State(s) to Queue__JKI_lib_State_Machine.vi"("State(s) in (\"\")"=w2656) -> ("States Out"=w2655:string)  [unwired: 14 in]
      }
      frame "APD: GetGainLimits" {
        w2661 = enum16{"Read", "Write"}."Read" ("Operation (Read)")
        # "Template Separator\n(You can make a copy of, or modify, this frame)"
        n1188 = call "APD1FGV.vi"("Error In"=w2660, "Operation (Read)"=w2661) -> ("Error Out"=w2673:errorcluster, "APDClass out"=w2674:refnum<class "APDClass.lvclass">)  [unwired: 8 in]
        n1189 = call "APD2FGV.vi"("Error In"=w2660, "Operation (Read)"=w2661) -> ("Error Out"=w2670:errorcluster, "APDClass out"=w2671:refnum<class "APDClass.lvclass">)  [unwired: 8 in]
        n1190 = call "APD3FGV.vi"("Error In"=w2660, "Operation (Read)"=w2661) -> ("Error Out"=w2668:errorcluster, "APDClass out"=w2669:refnum<class "APDClass.lvclass">)  [unwired: 8 in]
        n1191 = call "APD4FGV.vi"("Error In"=w2660, "Operation (Read)"=w2661) -> ("Error Out"=w2659:errorcluster, "APDClass out"=w2658:refnum<class "APDClass.lvclass">)  [unwired: 8 in]
        n1192 = call-dynamic "Read Gain Limits(Log).vi"("error in (no error)"=w2659, "APDClass in"=w2658) -> ("GainLimits(Log)"=w2657:cluster{"GainMax":dbl, "GainMin":dbl})  [unwired: 7 in, 2 out]
        n1193 = call-dynamic "Read Gain Limits(Log).vi"("error in (no error)"=w2673, "APDClass in"=w2674) -> ("error out"=w2665:errorcluster, "GainLimits(Log)"=w2672:cluster{"GainMax":dbl, "GainMin":dbl})  [unwired: 7 in, 1 out]
        n1194 = call-dynamic "Read Gain Limits(Log).vi"("error in (no error)"=w2670, "APDClass in"=w2671) -> ("error out"=w2664:errorcluster, "GainLimits(Log)"=w2667:cluster{"GainMax":dbl, "GainMin":dbl})  [unwired: 7 in, 1 out]
        n1195 = call-dynamic "Read Gain Limits(Log).vi"("error in (no error)"=w2668, "APDClass in"=w2669) -> ("error out"=w2663:errorcluster, "GainLimits(Log)"=w2666:cluster{"GainMax":dbl, "GainMin":dbl})  [unwired: 7 in, 1 out]
        n1196 = global write "GlobalVariables.vi" "Ch1GainLim(Log)"(w2672) -> ()
        n1197 = global write "GlobalVariables.vi" "Ch2GainLim(Log)"(w2667) -> ()
        n1198 = global write "GlobalVariables.vi" "Ch3GainLim(Log)"(w2666) -> ()
        n1199 = global write "GlobalVariables.vi" "Ch4GainLim(Log)"(w2657) -> ()
        n1200 = Merge Errors(w2665, w2664, w2663) -> (w2662:errorcluster)
        n1201 = call <vilib>:"Add State(s) to Queue__JKI_lib_State_Machine.vi"("State(s) in (\"\")"=w2678) -> ("States Out"=w2677:string)  [unwired: 14 in]
      }
      frame "APD: UpdateIndicatorMacro" {
        # "update indicator for all channel\n(You can make a copy of, or modify, this frame)"
        n1202 = call <vilib>:"Add State(s) to Queue__JKI_lib_State_Machine.vi"("State(s) in Front (\"\")"="APD: UpdateIndicatorCh1\nAPD: UpdateIndicatorCh2\nAPD: UpdateIndicatorCh3\nAPD: UpdateIndicatorCh4" ("State(s) in Front (\"\")"), "State(s) in (\"\")"=w2684) -> ("States Out"=w2683:string)  [unwired: 13 in]
      }
      frame "APD: UpdateIndicatorCh1" {
        # "Update APD module front panel indicators\n(Read data, update FGV, update plot)"
        n1203 = call "APD1FGV.vi"("Error In"=w2685) -> ("Error Out"=w2704:errorcluster, "APDClass out"=w2705:refnum<class "APDClass.lvclass">)  [unwired: 9 in]
        n1204 = call-dynamic "Read APD Serial.vi"("error in (no error)"=w2704, "APDClass in"=w2705) -> ("error out"=w2692:errorcluster, "APD Serial #"=w2701:string, "APDClass out"=w2694:refnum<class "APDClass.lvclass">)  [unwired: 7 in]
        n1205 = call-dynamic "Read DateTime.vi"("error in (no error)"=w2692, "APDClass in"=w2694) -> ("error out"=w2691:errorcluster, "DateTime"=→"DateTimeCh1":string, "APDClass out"=w2693:refnum<class "APDClass.lvclass">)  [unwired: 7 in]
        n1206 = local write "Serial Number Ch1"(w2701) -> ()
        n1207 = call-dynamic "Read GainData.vi"("error in (no error)"=w2691, "APDClass in"=w2693) -> ("error out"=w2702:errorcluster, "GainData"=w2695:T40, "APDClass out"=w2703:refnum<class "APDClass.lvclass">)  [unwired: 7 in]
        n1208 = Unbundle By Name(w2695) -> ("CtrlV"=w2690:dbl[], "Gain"=w2689:dbl[])
        n1209 = call-dynamic "Read iRFData.vi"("error in (no error)"=w2702, "APDClass in"=w2703) -> ("error out"=w2697:errorcluster, "iRFData"=w2700:T41)  [unwired: 7 in, 1 out]
        n1210 = Array Max & Min(array=w2690) -> (max value=→"Ch1 Max CtrlV":dbl)  [unwired: 3 out]
        n1211 = Bundle("CtrlV"=w2690, "Gain"=w2689) -> (→"Ch1 Gain":cluster{"CtrlV":dbl[], "Gain":dbl[]})  [unwired: 1 in]
        n1212 = Unbundle By Name(w2700) -> ("iRFWFsAvg"=→"Ch1 iRF Graph":dbl[][], "dt"=w2698:dbl)
        n1213 = property on="Ch1 iRF Graph" class="WFGraph (strict)"(error in=w2697, "XScale.Multiplier"=w2698) -> (error out=w2696:errorcluster)  [unwired: 1 in, 1 out]
        n1214 = call <vilib>:"Add State(s) to Queue__JKI_lib_State_Machine.vi"("State(s) in (\"\")"=w2709) -> ("States Out"=w2708:string)  [unwired: 14 in]
      }
      frame "APD: UpdateIndicatorCh2" {
        # "Update Channel 2 indicators\n(You can make a copy of, or modify, this frame)"
        n1215 = call "APD2FGV.vi"("Error In"=w2711) -> ("Error Out"=w2727:errorcluster, "APDClass out"=w2728:refnum<class "APDClass.lvclass">)  [unwired: 9 in]
        n1216 = call-dynamic "Read APD Serial.vi"("error in (no error)"=w2727, "APDClass in"=w2728) -> ("error out"=w2717:errorcluster, "APD Serial #"=w2726:string, "APDClass out"=w2719:refnum<class "APDClass.lvclass">)  [unwired: 7 in]
        n1217 = call-dynamic "Read DateTime.vi"("error in (no error)"=w2717, "APDClass in"=w2719) -> ("error out"=w2716:errorcluster, "DateTime"=→"DateTimeCh2":string, "APDClass out"=w2718:refnum<class "APDClass.lvclass">)  [unwired: 7 in]
        n1218 = local write "Serial Number Ch2"(w2726) -> ()
        n1219 = call-dynamic "Read GainData.vi"("error in (no error)"=w2716, "APDClass in"=w2718) -> ("error out"=w2729:errorcluster, "GainData"=w2721:T40, "APDClass out"=w2730:refnum<class "APDClass.lvclass">)  [unwired: 7 in]
        n1220 = Unbundle By Name(w2721) -> ("CtrlV"=w2714:dbl[], "Gain"=w2713:dbl[])
        n1221 = call-dynamic "Read iRFData.vi"("error in (no error)"=w2729, "APDClass in"=w2730) -> ("error out"=w2722:errorcluster, "iRFData"=w2725:T41)  [unwired: 7 in, 1 out]
        n1222 = Array Max & Min(array=w2714) -> (max value=→"Ch2 Max CtrlV":dbl)  [unwired: 3 out]
        n1223 = Bundle("CtrlV"=w2714, "Gain"=w2713) -> (→"Ch2 Gain":cluster{"CtrlV":dbl[], "Gain":dbl[]})  [unwired: 1 in]
        n1224 = Unbundle By Name(w2725) -> ("iRFWFsAvg"=→"Ch2 iRF Graph":dbl[][], "dt"=w2723:dbl)
        n1225 = property on="Ch2 iRF Graph" class="WFGraph (strict)"(error in=w2722, "XScale.Multiplier"=w2723) -> (error out=w2710:errorcluster)  [unwired: 1 in, 1 out]
        n1226 = call <vilib>:"Add State(s) to Queue__JKI_lib_State_Machine.vi"("State(s) in (\"\")"=w2734) -> ("States Out"=w2733:string)  [unwired: 14 in]
      }
      frame "APD: UpdateIndicatorCh3" {
        # "update ch3 indicator\n(You can make a copy of, or modify, this frame)"
        n1227 = call "APD3FGV.vi"("Error In"=w2735) -> ("Error Out"=w2753:errorcluster, "APDClass out"=w2754:refnum<class "APDClass.lvclass">)  [unwired: 9 in]
        n1228 = call-dynamic "Read APD Serial.vi"("error in (no error)"=w2753, "APDClass in"=w2754) -> ("error out"=w2745:errorcluster, "APD Serial #"=w2747:string, "APDClass out"=w2746:refnum<class "APDClass.lvclass">)  [unwired: 7 in]
        n1229 = call-dynamic "Read DateTime.vi"("error in (no error)"=w2745, "APDClass in"=w2746) -> ("error out"=w2743:errorcluster, "DateTime"=→"DateTimeCh3":string, "APDClass out"=w2744:refnum<class "APDClass.lvclass">)  [unwired: 7 in]
        n1230 = local write "Serial Number Ch3"(w2747) -> ()
        n1231 = call-dynamic "Read GainData.vi"("error in (no error)"=w2743, "APDClass in"=w2744) -> ("error out"=w2752:errorcluster, "GainData"=w2742:T40, "APDClass out"=w2755:refnum<class "APDClass.lvclass">)  [unwired: 7 in]
        n1232 = Unbundle By Name(w2742) -> ("CtrlV"=w2741:dbl[], "Gain"=w2740:dbl[])
        n1233 = call-dynamic "Read iRFData.vi"("error in (no error)"=w2752, "APDClass in"=w2755) -> ("error out"=w2751:errorcluster, "iRFData"=w2748:T41)  [unwired: 7 in, 1 out]
        n1234 = Array Max & Min(array=w2741) -> (max value=→"Ch3 Max CtrlV":dbl)  [unwired: 3 out]
        n1235 = Bundle("CtrlV"=w2741, "Gain"=w2740) -> (→"Ch3 Gain":cluster{"CtrlV":dbl[], "Gain":dbl[]})  [unwired: 1 in]
        n1236 = Unbundle By Name(w2748) -> ("iRFWFsAvg"=→"Ch3 iRF Graph":dbl[][], "dt"=w2750:dbl)
        n1237 = property on="Ch3 iRF Graph" class="WFGraph (strict)"(error in=w2751, "XScale.Multiplier"=w2750) -> (error out=w2736:errorcluster)  [unwired: 1 in, 1 out]
        n1238 = call <vilib>:"Add State(s) to Queue__JKI_lib_State_Machine.vi"("State(s) in (\"\")"=w2759) -> ("States Out"=w2758:string)  [unwired: 14 in]
      }
      frame "APD: UpdateIndicatorCh4" {
        # "update ch4 indicators\n(You can make a copy of, or modify, this frame)"
        n1239 = call "APD4FGV.vi"("Error In"=w2776) -> ("Error Out"=w2780:errorcluster, "APDClass out"=w2775:refnum<class "APDClass.lvclass">)  [unwired: 9 in]
        n1240 = call-dynamic "Read APD Serial.vi"("error in (no error)"=w2780, "APDClass in"=w2775) -> ("error out"=w2779:errorcluster, "APD Serial #"=→"Serial Number Ch4":string, "APDClass out"=w2774:refnum<class "APDClass.lvclass">)  [unwired: 7 in]
        n1241 = call-dynamic "Read DateTime.vi"("error in (no error)"=w2779, "APDClass in"=w2774) -> ("error out"=w2778:errorcluster, "DateTime"=→"DateTimeCh4":string, "APDClass out"=w2773:refnum<class "APDClass.lvclass">)  [unwired: 7 in]
        n1242 = call-dynamic "Read GainData.vi"("error in (no error)"=w2778, "APDClass in"=w2773) -> ("error out"=w2777:errorcluster, "GainData"=w2769:T40, "APDClass out"=w2772:refnum<class "APDClass.lvclass">)  [unwired: 7 in]
        n1243 = Unbundle By Name(w2769) -> ("CtrlV"=w2767:dbl[], "Gain"=w2766:dbl[])
        n1244 = call-dynamic "Read iRFData.vi"("error in (no error)"=w2777, "APDClass in"=w2772) -> ("error out"=w2761:errorcluster, "iRFData"=w2764:T41)  [unwired: 7 in, 1 out]
        n1245 = Array Max & Min(array=w2767) -> (max value=→"Ch4 Max CtrlV":dbl)  [unwired: 3 out]
        n1246 = Bundle("CtrlV"=w2767, "Gain"=w2766) -> (→"Ch4 Gain":cluster{"CtrlV":dbl[], "Gain":dbl[]})  [unwired: 1 in]
        n1247 = Unbundle By Name(w2764) -> ("iRFWFsAvg"=→"Ch4 iRF Graph":dbl[][], "dt"=w2762:dbl)
        n1248 = property on="Ch4 iRF Graph" class="WFGraph (strict)"(error in=w2761, "XScale.Multiplier"=w2762) -> (error out=w2760:errorcluster)  [unwired: 1 in, 1 out]
        n1249 = call <vilib>:"Add State(s) to Queue__JKI_lib_State_Machine.vi"("State(s) in (\"\")"=w2784) -> ("States Out"=w2783:string)  [unwired: 14 in]
      }
      frame "APD: writeGain" {
        w2785 = T40 {"CtrlV"=[], "NumOfWFs"=0, "WF length"=0, "Gain"=[], "GainRaw"=[], "GainBGRaw"=[]}  # GainData
        # "Parse all data for all gain\n(parse data all gain)"
        n1250 = Flush Queue(queue=w2797, error in (no error)=w2798) -> (remaining elements=w2794:cluster{"CtrlV":dbl, "WFs":dbl[][]}[], error out=w2792:errorcluster)  [unwired: 1 out]
        n1251 = for {
          tunnel: w2794 -> [w2841] mode=indexing
          tunnel: [w2840] -> w2791 mode=indexing
          tunnel: [w2837] -> w2787
          tunnel: [w2834] -> w2786
          # "Reshape gain WF array to vectors"
          n1252 = Unbundle By Name(w2841) -> ("WFs"=w2839:dbl[][])
          n1253 = Array Size(array=w2839) -> (size(s)=w2838:i32[])
          n1254 = for {
            tunnel: w2839 -> [w2842] mode=indexing
            tunnel: [w2842] -> w2840 mode=concatenating
          }
          n1255 = Index Array(array=w2838, index #1=0 ("index"), index #2=1 ("index")) -> (element #1=w2834:i32, element #2=w2837:i32)
        }
        n1256 = local read "Ctrl V"() -> (w2789:dbl[])
        n1257 = local read "Gain"() -> (w2788:dbl[])
        n1258 = Bundle By Name(cluster=w2785, "CtrlV"=w2789, "Gain"=w2788, "WF length"=w2787, "NumOfWFs"=w2786, "GainRaw"=w2791) -> (w2790:T40)
        n1259 = local read "Channel"() -> (w2793:enum32{"Ch1", "Ch2", "Ch3", "Ch4"})
        n1260 = case shown="\"Ch4\"" w2793 {
          tunnel: [w2803 w2810 w2818 w2826] -> w2796
          tunnel: w2792 -> [w2809 w2817 w2825 w2833]
          tunnel: w2790 -> [w2807 w2814 w2822 w2830]
          frame "Ch1", Default {
            n1261 = call "APD1FGV.vi"("Error In"=w2809) -> ("Error Out"=w2808:errorcluster, "APDClass out"=w2806:refnum<class "APDClass.lvclass">)  [unwired: 9 in]
            n1262 = call-dynamic "Write GainData.vi"("error in (no error)"=w2808, "GainData"=w2807, "APDClass in"=w2806) -> ("error out"=w2804:errorcluster, "APDClass out"=w2805:refnum<class "APDClass.lvclass">)  [unwired: 7 in]
            n1263 = call "APD1FGV.vi"("Error In"=w2804, "Operation (Read)"=enum16{"Read", "Write"}."Write", "APDClass in"=w2805) -> ("Error Out"=w2803:errorcluster)  [unwired: 7 in, 1 out]
          }
          frame "Ch2" {
            n1264 = call "APD2FGV.vi"("Error In"=w2817) -> ("Error Out"=w2815:errorcluster, "APDClass out"=w2816:refnum<class "APDClass.lvclass">)  [unwired: 9 in]
            n1265 = call-dynamic "Write GainData.vi"("error in (no error)"=w2815, "GainData"=w2814, "APDClass in"=w2816) -> ("error out"=w2811:errorcluster, "APDClass out"=w2813:refnum<class "APDClass.lvclass">)  [unwired: 7 in]
            n1266 = call "APD2FGV.vi"("Error In"=w2811, "Operation (Read)"=enum16{"Read", "Write"}."Write", "APDClass in"=w2813) -> ("Error Out"=w2810:errorcluster)  [unwired: 7 in, 1 out]
          }
          frame "Ch3" {
            n1267 = call "APD3FGV.vi"("Error In"=w2825) -> ("Error Out"=w2823:errorcluster, "APDClass out"=w2824:refnum<class "APDClass.lvclass">)  [unwired: 9 in]
            n1268 = call-dynamic "Write GainData.vi"("error in (no error)"=w2823, "GainData"=w2822, "APDClass in"=w2824) -> ("error out"=w2819:errorcluster, "APDClass out"=w2821:refnum<class "APDClass.lvclass">)  [unwired: 7 in]
            n1269 = call "APD3FGV.vi"("Error In"=w2819, "Operation (Read)"=enum16{"Read", "Write"}."Write", "APDClass in"=w2821) -> ("Error Out"=w2818:errorcluster)  [unwired: 7 in, 1 out]
          }
          frame "Ch4" {
            n1270 = call "APD4FGV.vi"("Error In"=w2833) -> ("Error Out"=w2831:errorcluster, "APDClass out"=w2832:refnum<class "APDClass.lvclass">)  [unwired: 9 in]
            n1271 = call-dynamic "Write GainData.vi"("error in (no error)"=w2831, "GainData"=w2830, "APDClass in"=w2832) -> ("error out"=w2827:errorcluster, "APDClass out"=w2829:refnum<class "APDClass.lvclass">)  [unwired: 7 in]
            n1272 = call "APD4FGV.vi"("Error In"=w2827, "Operation (Read)"=enum16{"Read", "Write"}."Write", "APDClass in"=w2829) -> ("Error Out"=w2826:errorcluster)  [unwired: 7 in, 1 out]
          }
        }
        n1273 = call <vilib>:"Add State(s) to Queue__JKI_lib_State_Machine.vi"("State(s) in (\"\")"=w2801) -> ("States Out"=w2800:string)  [unwired: 14 in]
      }
      frame "APD: writeiRF" {
        w2852 = T41 {"dt"=0.0, "NumOfWFs"=0, "WFLength"=0, "iRFCtrlV"=[], "iRFWFsAvg"=[], "iRFRaw"=[]}  # iRF
        # "Parse all data for all gain\n(parse data all gain)"
        n1274 = Flush Queue(queue=w2861, error in (no error)=w2859) -> (remaining elements=w2857:T42, error out=w2854:errorcluster)  [unwired: 1 out]
        n1275 = for {
          tunnel: w2857 -> [w2909] mode=indexing
          tunnel: [w2907] -> w2850 mode=indexing
          tunnel: [w2908] -> w2849 mode=indexing
          tunnel: [w2906] -> w2851 mode=indexing
          shift-right: [w2902] -> w2848
          shift-left: i32[] [] -> [w2901]
          i -> [w2905]
          n1276 = Equal To 0?(x=w2905) -> (x = 0?=w2904:bool)
          n1277 = Unbundle By Name(w2909) -> ("CtrlV"=w2907:dbl, "WFavg"=w2908:dbl[], "WFs"=w2903:dbl[][])
          n1278 = case shown="False" w2904 {
            tunnel: w2903 -> [_ w2912]
            tunnel: [w2910 w2911] -> w2902
            tunnel: w2901 -> [w2910 _]
            frame False {
            }
            frame True {
              n1279 = Array Size(array=w2912) -> (size(s)=w2911:i32[])
            }
          }
          n1280 = for {
            tunnel: w2903 -> [w2913] mode=indexing
            tunnel: [w2913] -> w2906 mode=concatenating
          }
        }
        n1281 = Index Array(array=w2848, index #1=0 ("index (row)"), index #2=1 ("disabled index (col)")) -> (element #1=w2844:i32, element #2=w2843:i32)
        n1282 = Bundle By Name(cluster=w2852, "dt"=0.2, "NumOfWFs"=w2844, "WFLength"=w2843, "iRFCtrlV"=w2850, "iRFWFsAvg"=w2849, "iRFRaw"=w2851) -> (w2853:T41)
        n1283 = local read "Channel"() -> (w2855:enum32{"Ch1", "Ch2", "Ch3", "Ch4"})
        n1284 = case shown="\"Ch1\", Default" w2855 {
          tunnel: w2854 -> [w2873 w2881 w2890 w2899]
          tunnel: w2849 -> [w2872 w2882 w2891 w2900]
          tunnel: w2853 -> [w2870 w2878 w2885 w2894]
          tunnel: [w2865 w2874 w2883 w2892] -> w2860
          frame "Ch1", Default {
            n1285 = local write "Ch1 iRF Graph"(w2872) -> ()
            n1286 = call "APD1FGV.vi"("Error In"=w2873) -> ("Error Out"=w2871:errorcluster, "APDClass out"=w2869:refnum<class "APDClass.lvclass">)  [unwired: 9 in]
            n1287 = call-dynamic "Write iRFData.vi"("error in (no error)"=w2871, "iRFData"=w2870, "APDClass in"=w2869) -> ("error out"=w2868:errorcluster, "APDClass out"=w2867:refnum<class "APDClass.lvclass">)  [unwired: 7 in]
            n1288 = call "APD1FGV.vi"("Error In"=w2868, "Operation (Read)"=enum16{"Read", "Write"}."Write", "APDClass in"=w2867) -> ("Error Out"=w2865:errorcluster)  [unwired: 7 in, 1 out]
          }
          frame "Ch2" {
            n1289 = local write "Ch2 iRF Graph"(w2882) -> ()
            n1290 = call "APD2FGV.vi"("Error In"=w2881) -> ("Error Out"=w2880:errorcluster, "APDClass out"=w2879:refnum<class "APDClass.lvclass">)  [unwired: 9 in]
            n1291 = call-dynamic "Write iRFData.vi"("error in (no error)"=w2880, "iRFData"=w2878, "APDClass in"=w2879) -> ("error out"=w2876:errorcluster, "APDClass out"=w2877:refnum<class "APDClass.lvclass">)  [unwired: 7 in]
            n1292 = call "APD2FGV.vi"("Error In"=w2876, "Operation (Read)"=enum16{"Read", "Write"}."Write", "APDClass in"=w2877) -> ("Error Out"=w2874:errorcluster)  [unwired: 7 in, 1 out]
          }
          frame "Ch3" {
            n1293 = local write "Ch3 iRF Graph"(w2891) -> ()
            n1294 = call "APD3FGV.vi"("Error In"=w2890) -> ("Error Out"=w2889:errorcluster, "APDClass out"=w2887:refnum<class "APDClass.lvclass">)  [unwired: 9 in]
            n1295 = call-dynamic "Write iRFData.vi"("error in (no error)"=w2889, "iRFData"=w2885, "APDClass in"=w2887) -> ("error out"=w2888:errorcluster, "APDClass out"=w2886:refnum<class "APDClass.lvclass">)  [unwired: 7 in]
            n1296 = call "APD3FGV.vi"("Error In"=w2888, "Operation (Read)"=enum16{"Read", "Write"}."Write", "APDClass in"=w2886) -> ("Error Out"=w2883:errorcluster)  [unwired: 7 in, 1 out]
          }
          frame "Ch4" {
            n1297 = local write "Ch4 iRF Graph"(w2900) -> ()
            n1298 = call "APD4FGV.vi"("Error In"=w2899) -> ("Error Out"=w2898:errorcluster, "APDClass out"=w2896:refnum<class "APDClass.lvclass">)  [unwired: 9 in]
            n1299 = call-dynamic "Write iRFData.vi"("error in (no error)"=w2898, "iRFData"=w2894, "APDClass in"=w2896) -> ("error out"=w2897:errorcluster, "APDClass out"=w2895:refnum<class "APDClass.lvclass">)  [unwired: 7 in]
            n1300 = call "APD4FGV.vi"("Error In"=w2897, "Operation (Read)"=enum16{"Read", "Write"}."Write", "APDClass in"=w2895) -> ("Error Out"=w2892:errorcluster)  [unwired: 7 in, 1 out]
          }
        }
        n1301 = call <vilib>:"Add State(s) to Queue__JKI_lib_State_Machine.vi"("State(s) in (\"\")"=w2864) -> ("States Out"=w2863:string)  [unwired: 14 in]
      }
      frame "APD: SaveNew" {
        # "Save APD info\n(You can make a copy of, or modify, this frame)"
        n1302 = local read "Channel"() -> (w2918:enum32{"Ch1", "Ch2", "Ch3", "Ch4"})
        n1303 = case shown="\"Ch4\"" w2918 {
          tunnel: [w2927 w2930 w2933 w2936] -> w2917
          tunnel: w2916 -> [w2926 w2928 w2931 w2934]
          tunnel: [w2925 w2929 w2932 w2935] -> w2915
          frame "Ch1", Default {
            n1304 = call "APD1FGV.vi"("Error In"=w2926) -> ("Error Out"=w2925:errorcluster, "APDClass out"=w2927:refnum<class "APDClass.lvclass">)  [unwired: 9 in]
          }
          frame "Ch2" {
            n1305 = call "APD2FGV.vi"("Error In"=w2928) -> ("Error Out"=w2929:errorcluster, "APDClass out"=w2930:refnum<class "APDClass.lvclass">)  [unwired: 9 in]
          }
          frame "Ch3" {
            n1306 = call "APD3FGV.vi"("Error In"=w2931) -> ("Error Out"=w2932:errorcluster, "APDClass out"=w2933:refnum<class "APDClass.lvclass">)  [unwired: 9 in]
          }
          frame "Ch4" {
            n1307 = call "APD4FGV.vi"("Error In"=w2934) -> ("Error Out"=w2935:errorcluster, "APDClass out"=w2936:refnum<class "APDClass.lvclass">)  [unwired: 9 in]
          }
        }
        n1308 = call "Write to File.vi"("Error In"=w2915, "APDClass.lvclass"=w2917) -> ("Error Out"=w2914:errorcluster)  [unwired: 9 in]
        n1309 = case shown="Error .." w2914 {
          frame No Error {
            n1310 = One Button Dialog(message="Data saved successfully!") -> ()  [unwired: 1 in, 1 out]
          }
          frame Error {
            n1311 = One Button Dialog(message="Error saving to APD file!") -> ()  [unwired: 1 in, 1 out]
          }
        }
        n1312 = call <vilib>:"Add State(s) to Queue__JKI_lib_State_Machine.vi"("State(s) in (\"\")"=w2922) -> ("States Out"=w2921:string)  [unwired: 14 in]
      }
      frame "---------- Aquisition ----------" {
        # "Template Separator\n(You can make a copy of, or modify, this frame)"
        n1313 = call <vilib>:"Add State(s) to Queue__JKI_lib_State_Machine.vi"("State(s) in (\"\")"=w2941) -> ("States Out"=w2940:string)  [unwired: 14 in]
      }
      frame "Aquisition: EnqueueV" {
        # "Enqueue aquisition V\n(You can make a copy of, or modify, this frame)"
        n1314 = while {
          tunnel: w2946 -> [w2964]
          shift-right: [w2962] -> w2945
          shift-left: w2944 -> [w2963]
          shift-right: [w2956] -> _
          shift-left: "Gain low" -> [w2960]
          tunnel: "Step" -> [w2957]
          tunnel: "Gain High" -> [w2958]
          tunnel: "Gain low" -> [w2961]
          stop <- w2955 stop-if-true
          # "check gain value, stop if out of range"
          n1315 = Add(x=w2958, y=w2957) -> (x+y=w2954:dbl)
          n1316 = In Range and Coerce(upper limit=w2958, x=w2960, lower limit=w2961) -> (coerced(x)=w2959:dbl)  [unwired: 1 out]
          n1317 = Enqueue Element(queue=w2964, element=w2959, error in (no error)=w2963) -> (error out=w2962:errorcluster)  [unwired: 1 in, 2 out]
          n1318 = Subtract(x=w2954, y=0.0001) -> (x-y=w2952:dbl)
          n1319 = Add(x=w2960, y=w2957) -> (x+y=w2956:dbl)
          n1320 = Greater Or Equal?(x=w2956, y=w2952) -> (x >= y?=w2955:bool)
        }
        n1321 = call <vilib>:"Add State(s) to Queue__JKI_lib_State_Machine.vi"("State(s) in (\"\")"=w2951) -> ("States Out"=w2950:string)  [unwired: 14 in]
      }
      frame "Aquisition: RecordData" {
        # "Set gain\nstart aquisition\nask user to adjust signal level\nstop aquisition\nstart aquisition"
        # "Template Separator\n(You can make a copy of, or modify, this frame)"
        n1322 = Fract/Exp String To Number(string=w2965) -> (number=w2970:dbl)  [unwired: 3 in, 1 out]
        n1323 = call "V1FGV.vi"("Error In"=w2969, "action (write)"=enum16{"write", "read"}."write" ("action"), "V1 in"=w2970) -> ("Error Out"=w2968:errorcluster)  [unwired: 7 in, 1 out]
        n1324 = call <vilib>:"Add State(s) to Queue__JKI_lib_State_Machine.vi"("State(s) in Front (\"\")"="Queue: Flash\nUtility: setSaveFlag >> 0\nMacro: StartRun\nUI: ShowDialog\nUtility: setSaveFlag >> 1\nQueue: CheckNumOfWF\nMacro: StopRun\n" ("State(s) in Front (\"\")"), "State(s) in (\"\")"=w2974) -> ("States Out"=w2973:string)  [unwired: 13 in]
      }
      frame "---------- File ----------" {
        # "Template Separator\n(You can make a copy of, or modify, this frame)"
        n1325 = call <vilib>:"Add State(s) to Queue__JKI_lib_State_Machine.vi"("State(s) in (\"\")"=w2979) -> ("States Out"=w2978:string)  [unwired: 14 in]
      }
      frame "File: BackupOld" {
        w2987 = ".tdms" ("string")
        # ".tdms_index file is not required for storage or distribution and automatically regenerates\nno need to copy the index file"
        # "Backup old APD data file\n()"
        n1326 = local read "Channel"() -> (w2997:enum32{"Ch1", "Ch2", "Ch3", "Ch4"})
        n1327 = case shown="\"Ch2\"" w2997 {
          tunnel: [w3002 w3003 w3004 w3005] -> w2988
          frame "Ch1", Default {
            n1328 = local read "Serial Number Ch1"() -> (w3002:string)
          }
          frame "Ch2" {
            n1329 = local read "Serial Number Ch2"() -> (w3003:string)
          }
          frame "Ch3" {
            n1330 = local read "Serial Number Ch3"() -> (w3004:string)
          }
          frame "Ch4" {
            n1331 = local read "Serial Number Ch4"() -> (w3005:string)
          }
        }
        n1332 = call <vilib>:"Application Directory.vi"() -> ("Application Directory"=w2998:path)
        n1333 = Get Date/Time In Seconds() -> (seconds since 1Jan1904=w2992:timestamp)
        n1334 = Format Date/Time String(time format string (%c)="%m-%d-%Y %H-%M", seconds (now)=w2992) -> (date/time string=w2991:string)  [unwired: 1 in]
        n1335 = Build Path(base path=w2998, name or relative path="ConfigFiles") -> (appended path=w2995:path)
        n1336 = Build Path(base path=w2995, name or relative path="Backup") -> (appended path=w2994:path)
        n1337 = Concatenate Strings(w2988, w2987) -> (w2989:string)
        n1338 = Concatenate Strings(w2988, " BK " ("string"), w2991, w2987) -> (w2990:string)
        n1339 = Build Path(base path=w2995, name or relative path=w2989) -> (appended path=w2996:path)
        n1340 = Build Path(base path=w2994, name or relative path=w2990) -> (appended path=w2993:path)
        n1341 = Copy(8:w2982, 10:w2993, 11:w2996) -> (0:w2981:errorcluster)  [unwired: 2 in, 2 out]
        n1342 = call <vilib>:"Add State(s) to Queue__JKI_lib_State_Machine.vi"("State(s) in (\"\")"=w3001) -> ("States Out"=w3000:string)  [unwired: 14 in]
      }
      frame "---------- PID ----------" {
        # "Template Separator\n(You can make a copy of, or modify, this frame)"
        n1343 = call <vilib>:"Add State(s) to Queue__JKI_lib_State_Machine.vi"("State(s) in (\"\")"=w3010) -> ("States Out"=w3009:string)  [unwired: 14 in]
      }
      frame "PID: loadPID" {
        # "Template Separator\n(You can make a copy of, or modify, this frame)"
        n1344 = call "readPIDSetting.vi"("Error In"=w3014) -> ("Error Out"=w3015:errorcluster, "Ch3 PID out"=w3011:T6, "Ch2 PID out"=w3012:T6, "Ch1 PID out"=w3013:T6)  [unwired: 7 in]
        n1345 = local write "Ch1 PID gains"(w3013) -> ()
        n1346 = local write "Ch2 PID gains"(w3012) -> ()
        n1347 = local write "Ch3 PID gains"(w3011) -> ()
        n1348 = call <vilib>:"Add State(s) to Queue__JKI_lib_State_Machine.vi"("State(s) in (\"\")"=w3019) -> ("States Out"=w3018:string)  [unwired: 14 in]
      }
      frame "---------- Template ----------" {
        # "Template Separator\n(You can make a copy of, or modify, this frame)"
        n1349 = call <vilib>:"Add State(s) to Queue__JKI_lib_State_Machine.vi"("State(s) in (\"\")"=w3024) -> ("States Out"=w3023:string)  [unwired: 14 in]
      }
    }
  }
  n1350 = while {
    tunnel: w39 -> [w3057]
    shift-right: [w3039] -> _
    shift-left: w26 -> [w3038]
    tunnel: w36 -> [w3050]
    tunnel: [w3048] -> w35
    shift-right: [w3047] -> _
    shift-left: w23 -> [w3046]
    i -> [w3042]
    stop <- w3041 stop-if-true
    # "stop on error"
    # "Gain adjustment and Data processing"
    n1351 = Wait on Notification(notifier=w3057, ignore previous (F)=TRUE) -> (notification=w3055:cluster{"idx":i32, "CH1&2":dbl[][]}, error out=w3032:errorcluster)  [unwired: 2 in, 2 out]
    n1352 = call <vilib>:"High Resolution Relative Seconds.vi"() -> ("relative seconds"=w3047:dbl)
    n1353 = flat-sequence {
      tunnel: [w3193] -> w3026
      tunnel: w3032 -> [_]
      frame #0 {
        # "make sure it is read after data arrive"
        n1354 = local read "Auto gain"() -> (w3193:bool)
      }
    }
    n1355 = Subtract(x=w3047, y=w3046) -> (x-y=w3045:dbl)
    n1356 = Unbundle(w3055) -> ("CH1&2"=w3037:dbl[][])  [unwired: 1 out]
    n1357 = call "AvgArrayTimeCritical.vi"("2D array"=w3037) -> ("1D Avg"=w3036:dbl[])  [unwired: 10 in]
    n1358 = Multiply(x=w3045, y=1000.0) -> (x*y=→"processing loop timing(ms)":dbl)
    n1359 = Array Max & Min(array=w3036) -> (max value=w3029:dbl)  [unwired: 3 out]
    n1360 = local read "Channel"() -> (w3025:enum32{"Ch1", "Ch2", "Ch3", "Ch4"})
    n1361 = case shown="True" w3026 {
      tunnel: [w3062 w3094] -> w3033
      tunnel: w3032 -> [w3063 w3093]
      tunnel: [w3063 w3092] -> w3031
      tunnel: "V target(1.0)" -> [_ w3091]
      tunnel: w3029 -> [_ w3090]
      tunnel: [w3058 w3088] -> w3028
      tunnel: [w3059 w3087] -> w3027
      tunnel: w3025 -> [w3061 w3086]
      frame False {
        n1362 = case shown="\"Ch4\"" w3061 {
          tunnel: [w3066 w3068 w3070 w3072] -> w3062
          tunnel: [enum16{"Ch1", "Ch2", "Ch3"}."Ch1" ("Channel") enum16{"Ch1", "Ch2", "Ch3"}."Ch2" ("Channel") enum16{"Ch1", "Ch2", "Ch3"}."Ch3" ("Channel") enum16{"Ch1", "Ch2", "Ch3", "Ch4"}."Ch4" ("Channel")] -> w3060
          frame "Ch1", Default {
            n1363 = global read "GlobalVariables.vi" "Ch1 LJ pin"() -> (w3066:string)
          }
          frame "Ch2" {
            n1364 = global read "GlobalVariables.vi" "Ch2 LJ pin"() -> (w3068:string)
          }
          frame "Ch3" {
            n1365 = global read "GlobalVariables.vi" "Ch3 LJ pin"() -> (w3070:string)
          }
          frame "Ch4" {
            n1366 = global read "GlobalVariables.vi" "Ch4 LJ pin"() -> (w3072:string)
          }
        }
        n1367 = call "V1FGV.vi"("action (write)"=enum16{"write", "read"}."read" ("action")) -> ("V1 out"=w3059:dbl)  [unwired: 9 in, 1 out]
        n1368 = call "CtrlVtoGain.vi"("CtrlV(V)"=w3059, "Channel"=w3060) -> ("Gain"=w3058:dbl)  [unwired: 8 in, 1 out]
      }
      frame True {
        n1369 = case shown="\"Ch4\"" w3086 {
          tunnel: [w3119 w3143 w3167 w3191] -> w3094
          tunnel: w3093 -> [w3118 w3142 w3166 w3190]
          tunnel: [w3118 w3142 w3166 w3190] -> w3092
          tunnel: [w3117 w3141 w3165 w3189] -> _
          tunnel: w3091 -> [w3106 w3130 w3154 w3179]
          tunnel: w3090 -> [w3105 w3129 w3153 w3178]
          tunnel: "autotune? (F)" -> [w3112 w3136 w3160 w3185]
          tunnel: [w3116 w3140 w3164 w3188] -> w3088
          tunnel: [w3098 w3121 w3145 w3170] -> w3087
          tunnel: "PID dt (s)" -> [w3108 w3132 w3156 w3181]
          tunnel: "autotuning parameters" -> [w3104 w3128 w3152 w3177]
          tunnel: [w3107 w3131 w3155 w3180] -> w3084
          tunnel: "Accept?" -> [w3103 w3127 w3151 w3176]
          tunnel: "Gain(Log)" -> [w3102 w3126 w3150 w3175]
          tunnel: [w3101 w3125 w3149 w3174] -> w3080
          tunnel: [w3101 w3125 w3149 w3174] -> w3079
          tunnel: [w3100 w3124 w3148 w3173] -> w3078
          tunnel: [w3095 w3123 w3147 w3172] -> w3077
          tunnel: [w3099 w3122 w3146 w3171] -> w3076
          tunnel: [w3098 w3121 w3145 w3170] -> w3075
          tunnel: "gamma" -> [w3097 _ _ _]
          tunnel: "alpha" -> [w3096 _ _ _]
          frame "Ch1", Default {
            w3117 = enum16{"Ch1", "Ch2", "Ch3"}."Ch1" ("Enum")
            n1370 = global read "GlobalVariables.vi" "Ch1GainLim(Log)"() -> (w3110:cluster{"GainMax":dbl, "GainMin":dbl})
            n1371 = call-poly <vilib>:"PID Online Autotuning.vi"("setpoint"=w3106, "manipulated variable"=w3102, "autotuning parameters"=w3104, "process variable"=w3105, "PID gains in"="Ch1 PID gains", "dt (s)"=w3108, "autotune? (F)"=w3112) -> ("setpoint out"=w3114:dbl, "process variable out"=w3113:dbl, "tuning completed?"=w3099:bool, "PID gains out"=w3111:T6, "tuned PID gains"=w3095:T6)  [unwired: 4 in]
            n1372 = case shown="True" w3103 {
              tunnel: w3095 -> [_ w3120]
              frame False {
              }
              frame True {
                n1373 = local write "Ch1 PID gains"(w3120) -> ()
              }
            }
            n1374 = call-poly <vilib>:"PID Advanced.vi"("setpoint"=w3114, "output range"=w3110, "auto? (T)"=TRUE, "process variable"=w3113, "gamma"=w3097, "alpha"=w3096, "PID gains"=w3111, "dt (s)"=w3108) -> ("output"=w3101:dbl, "dt out (s)"=w3107:dbl)  [unwired: 6 in]
            n1375 = Power Of 10(x=w3101) -> (10^x=w3116:dbl)
            n1376 = call "GainToCtrlV.vi"("Gain"=w3116, "Channel"=w3117) -> ("CtrlV"=w3098:dbl)  [unwired: 8 in, 1 out]
            n1377 = global read "GlobalVariables.vi" "Ch1 LJ pin"() -> (w3119:string)
            n1378 = Bundle("V target(1.0)"=w3106, w3105) -> (w3100:cluster{"V target(1.0)":dbl, dbl})  [unwired: 1 in]
          }
          frame "Ch2" {
            w3141 = enum16{"Ch1", "Ch2", "Ch3"}."Ch2" ("Enum")
            n1379 = global read "GlobalVariables.vi" "Ch2GainLim(Log)"() -> (w3134:cluster{"GainMax":dbl, "GainMin":dbl})
            n1380 = call-poly <vilib>:"PID Online Autotuning.vi"("setpoint"=w3130, "manipulated variable"=w3126, "autotuning parameters"=w3128, "process variable"=w3129, "PID gains in"="Ch2 PID gains", "dt (s)"=w3132, "autotune? (F)"=w3136) -> ("setpoint out"=w3138:dbl, "process variable out"=w3137:dbl, "tuning completed?"=w3122:bool, "PID gains out"=w3135:T6, "tuned PID gains"=w3123:T6)  [unwired: 4 in]
            n1381 = case shown="True" w3127 {
              tunnel: w3123 -> [_ w3144]
              frame False {
              }
              frame True {
                n1382 = local write "Ch2 PID gains"(w3144) -> ()
              }
            }
            n1383 = call-poly <vilib>:"PID Advanced.vi"("setpoint"=w3138, "output range"=w3134, "auto? (T)"=TRUE, "process variable"=w3137, "PID gains"=w3135, "dt (s)"=w3132) -> ("output"=w3125:dbl, "dt out (s)"=w3131:dbl)  [unwired: 8 in]
            n1384 = Power Of 10(x=w3125) -> (10^x=w3140:dbl)
            n1385 = call "GainToCtrlV.vi"("Gain"=w3140, "Channel"=w3141) -> ("CtrlV"=w3121:dbl)  [unwired: 8 in, 1 out]
            n1386 = global read "GlobalVariables.vi" "Ch2 LJ pin"() -> (w3143:string)
            n1387 = Bundle("V target(1.0)"=w3130, w3129) -> (w3124:cluster{"V target(1.0)":dbl, dbl})  [unwired: 1 in]
          }
          frame "Ch3" {
            w3165 = enum16{"Ch1", "Ch2", "Ch3"}."Ch3" ("Enum")
            n1388 = global read "GlobalVariables.vi" "Ch3GainLim(Log)"() -> (w3158:cluster{"GainMax":dbl, "GainMin":dbl})
            n1389 = call-poly <vilib>:"PID Online Autotuning.vi"("setpoint"=w3154, "manipulated variable"=w3150, "autotuning parameters"=w3152, "process variable"=w3153, "PID gains in"="Ch3 PID gains", "dt (s)"=w3156, "autotune? (F)"=w3160) -> ("setpoint out"=w3162:dbl, "process variable out"=w3161:dbl, "tuning completed?"=w3146:bool, "PID gains out"=w3159:T6, "tuned PID gains"=w3147:T6)  [unwired: 4 in]
            n1390 = case shown="True" w3151 {
              tunnel: w3147 -> [_ w3168]
              frame False {
              }
              frame True {
                n1391 = local write "Ch3 PID gains"(w3168) -> ()
              }
            }
            n1392 = call-poly <vilib>:"PID Advanced.vi"("setpoint"=w3162, "output range"=w3158, "auto? (T)"=TRUE, "process variable"=w3161, "PID gains"=w3159, "dt (s)"=w3156) -> ("output"=w3149:dbl, "dt out (s)"=w3155:dbl)  [unwired: 8 in]
            n1393 = Power Of 10(x=w3149) -> (10^x=w3164:dbl)
            n1394 = call "GainToCtrlV.vi"("Gain"=w3164, "Channel"=w3165) -> ("CtrlV"=w3145:dbl)  [unwired: 8 in, 1 out]
            n1395 = global read "GlobalVariables.vi" "Ch3 LJ pin"() -> (w3167:string)
            n1396 = Bundle("V target(1.0)"=w3154, w3153) -> (w3148:cluster{"V target(1.0)":dbl, dbl})  [unwired: 1 in]
          }
          frame "Ch4" {
            w3189 = enum16{"Ch1", "Ch2", "Ch3"}."Ch3" ("Enum")
            n1397 = global read "GlobalVariables.vi" "Ch4GainLim(Log)"() -> (w3183:cluster{"GainMax":dbl, "GainMin":dbl})
            n1398 = call-poly <vilib>:"PID Online Autotuning.vi"("setpoint"=w3179, "manipulated variable"=w3175, "autotuning parameters"=w3177, "process variable"=w3178, "PID gains in"="Ch4 PID gains", "dt (s)"=w3181, "autotune? (F)"=w3185) -> ("setpoint out"=w3187:dbl, "process variable out"=w3186:dbl, "tuning completed?"=w3171:bool, "PID gains out"=w3184:T6, "tuned PID gains"=w3172:T6)  [unwired: 4 in]
            n1399 = case shown="True" w3176 {
              tunnel: w3172 -> [_ w3192]
              frame False {
              }
              frame True {
                n1400 = local write "Ch4 PID gains"(w3192) -> ()
              }
            }
            n1401 = call-poly <vilib>:"PID Advanced.vi"("setpoint"=w3187, "output range"=w3183, "auto? (T)"=TRUE, "process variable"=w3186, "PID gains"=w3184, "dt (s)"=w3181) -> ("output"=w3174:dbl, "dt out (s)"=w3180:dbl)  [unwired: 8 in]
            n1402 = Power Of 10(x=w3174) -> (10^x=w3188:dbl)
            n1403 = call "GainToCtrlV.vi"("Gain"=w3188, "Channel"=w3189) -> ("CtrlV"=w3170:dbl)  [unwired: 8 in, 1 out]
            n1404 = global read "GlobalVariables.vi" "Ch4 LJ pin"() -> (w3191:string)
            n1405 = Bundle("V target(1.0)"=w3179, w3178) -> (w3173:cluster{"V target(1.0)":dbl, dbl})  [unwired: 1 in]
          }
        }
        "dt out (s)" <- w3084
        "Gain(Log10)" <- w3079
        "Targer and Max" <- w3078
        "tuned PID gains" <- w3077
        "Completed?" <- w3076
        n1406 = local write "Ctrl V"(w3075) -> ()
        n1407 = local write "Gain(Log)"(w3080) -> ()
        n1408 = call "V1FGV.vi"("V1 in"=w3075) -> ()  [unwired: 9 in, 2 out]
      }
    }
    n1409 = local write "GainIndicator"(w3028) -> ()
    n1410 = call "LabJack_FGV.vi"("Operation(Read)"=enum16{"Write", "Read"}."Read" ("Operation"), "error in (no error)"=w3031) -> ("error out"=w3054:errorcluster, "Read data"=w3053:i32)  [unwired: 8 in]
    n1411 = Not Equal?(x=w3027, y=w3038) -> (x != y?=w3040:bool)
    n1412 = case shown="True" w3040 {
      tunnel: w3054 -> [w3195 w3196]
      tunnel: w3053 -> [_ w3200]
      tunnel: [w3195 w3199] -> w3034
      tunnel: w3027 -> [w3194 w3197]
      tunnel: [w3194 w3197] -> w3039
      tunnel: w3033 -> [_ w3198]
      frame False {
      }
      frame True {
        n1413 = call "LJM_eWriteName.vi"("Handle In"=w3200, "Name"=w3198, "Value"=w3197, "error in"=w3196) -> ("error out"=w3199:errorcluster)  [unwired: 10 in, 1 out]
      }
    }
    n1414 = Build Array(w3036) -> (w3035:dbl[][])
    n1415 = Bundle(w3035) -> (w3051:cluster{dbl[][]})  [unwired: 1 in]
    n1416 = Send Notification(notification=w3051, notifier=w3050) -> (notifier out=w3048:refnum<notifier>, error out=w3049:errorcluster)  [unwired: 1 in]
    n1417 = Merge Errors(w3034, w3049) -> (w3041:errorcluster)
    "processing Error Out" <- w3041
    "processing loop" <- w3042
  }
  n1418 = while {
    tunnel: w54 -> [w3213]
    tunnel: w44 -> [w3212]
    tunnel: [w3211] -> w52
    tunnel: w39 -> [w3210]
    tunnel: [w3209] -> w48
    tunnel: w27 -> [w3207]
    tunnel: w32 -> [w3206]
    tunnel: w24 -> [w3201]
    stop <- w3204 stop-if-true
    # "acquire data and send it to processing loop"
    # "Data Aquisition Loop"
    n1419 = event shown="[1] <Start digitizer>: User Event" {
      selector: w3212 -> [_ _]
      dyn-events: [_ _] -> w3211
      timeout: 20 -> [_ _]
      tunnel: w3213 -> [w3219 w3231]
      tunnel: [w3214 _] -> w3204
      tunnel: w3210 -> [w3218 w3237]
      tunnel: [w3218 w3236] -> w3209
      tunnel: w3207 -> [_ w3235]
      tunnel: w3206 -> [w3217 w3230]
      tunnel: w3201 -> [_ w3228]
      event Timeout {
        # "use queue to stop data loop\nwhen queue ref is released, error will stop this loop"
        n1420 = event-data() -> ()  [unwired: 1 in, 3 out]
        n1421 = Get Queue Status(queue=w3219) -> (error out=w3216:errorcluster)  [unwired: 2 in, 7 out]
        n1422 = Get Queue Status(queue=w3217) -> (error out=w3215:errorcluster)  [unwired: 2 in, 7 out]
        n1423 = Merge Errors(w3216, w3215) -> (w3214:errorcluster)
      }
      event User Event {
        n1424 = event-data() -> ()  [unwired: 1 in, 4 out]
        n1425 = local read "Channel"() -> (w3223:enum32{"Ch1", "Ch2", "Ch3", "Ch4"})
        n1426 = case shown="\"Ch4\"" w3223 {
          tunnel: [w3246 w3254 w3257 w3265] -> w3234
          tunnel: [w3244 w3252 w3259 w3267] -> w3227
          tunnel: [w3243 w3251 w3262 w3270] -> w3226
          tunnel: [w3242 w3250 w3261 w3269] -> w3225
          tunnel: [w3241 w3249 w3260 w3268] -> w3224
          tunnel: [w3240 w3248 w3256 w3264] -> w3222
          frame "Ch1", Default {
            w3240 = "0" ("Active Channel")
            w3247 = enum16{"Write", "Read"}."Read" ("Operation")
            n1427 = call "Digitizer1_FGV.vi"("Operation (Read)"=w3247) -> ("Read data"=w3245:refnum<k15>)  [unwired: 9 in, 1 out]
            n1428 = call "Digitizer2_FGV.vi"("Operation (Read)"=w3247) -> ("Read data"=w3246:refnum<k15>)  [unwired: 9 in, 1 out]
            n1429 = property on="Property Node" class="niScope"(reference=w3245, "Active Channel"=w3240) -> (reference out=w3244:refnum<k15>, error out=w3242:errorcluster, "Vertical Range"=w3241:dbl, "Vertical Offset"=w3243:dbl)  [unwired: 1 in]
          }
          frame "Ch2" {
            w3248 = "1" ("Active Channel")
            w3255 = enum16{"Write", "Read"}."Read" ("Operation")
            n1430 = call "Digitizer1_FGV.vi"("Operation (Read)"=w3255) -> ("Read data"=w3253:refnum<k15>)  [unwired: 9 in, 1 out]
            n1431 = call "Digitizer2_FGV.vi"("Operation (Read)"=w3255) -> ("Read data"=w3254:refnum<k15>)  [unwired: 9 in, 1 out]
            n1432 = property on="Property Node" class="niScope"(reference=w3253, "Active Channel"=w3248) -> (reference out=w3252:refnum<k15>, error out=w3250:errorcluster, "Vertical Range"=w3249:dbl, "Vertical Offset"=w3251:dbl)  [unwired: 1 in]
          }
          frame "Ch3" {
            w3256 = "0" ("Active Channel")
            w3263 = enum16{"Write", "Read"}."Read" ("Operation")
            n1433 = call "Digitizer2_FGV.vi"("Operation (Read)"=w3263) -> ("Read data"=w3258:refnum<k15>)  [unwired: 9 in, 1 out]
            n1434 = call "Digitizer1_FGV.vi"("Operation (Read)"=w3263) -> ("Read data"=w3259:refnum<k15>)  [unwired: 9 in, 1 out]
            n1435 = property on="Property Node" class="niScope"(reference=w3258, "Active Channel"=w3256) -> (reference out=w3257:refnum<k15>, error out=w3261:errorcluster, "Vertical Range"=w3260:dbl, "Vertical Offset"=w3262:dbl)  [unwired: 1 in]
          }
          frame "Ch4" {
            w3264 = "1" ("Active Channel")
            w3271 = enum16{"Write", "Read"}."Read" ("Operation")
            n1436 = call "Digitizer2_FGV.vi"("Operation (Read)"=w3271) -> ("Read data"=w3266:refnum<k15>)  [unwired: 9 in, 1 out]
            n1437 = call "Digitizer1_FGV.vi"("Operation (Read)"=w3271) -> ("Read data"=w3267:refnum<k15>)  [unwired: 9 in, 1 out]
            n1438 = property on="Property Node" class="niScope"(reference=w3266, "Active Channel"=w3264) -> (reference out=w3265:refnum<k15>, error out=w3269:errorcluster, "Vertical Range"=w3268:dbl, "Vertical Offset"=w3270:dbl)  [unwired: 1 in]
          }
        }
        n1439 = local read "Task"() -> (w3220:enum32{"iRFAndGain", "Alignment"})
        n1440 = case shown="\"Alignment\"" w3220 {
          tunnel: [0.25 ("timeout") 0.75 ("timeout")] -> w3221
          frame "iRFAndGain", Default {
          }
          frame "Alignment" {
          }
        }
        n1441 = call "FLImDAQ_FGV.vi"() -> ("Read data"=w3233:T4)  [unwired: 10 in, 1 out]
        n1442 = Unbundle By Name(w3233) -> ("Waveform to Avg"=w3232:i16)
        n1443 = while {
          tunnel: w3237 -> [w3310]
          tunnel: [w3309] -> w3236
          tunnel: w3234 -> [w3307]
          tunnel: w3227 -> [w3306]
          tunnel: w3235 -> [w3305]
          shift-right: [w3289] -> _
          shift-left: u32 0 ("millisecond timer value") -> [w3301]
          tunnel: w3232 -> [w3299]
          tunnel: w3231 -> [_]
          tunnel: w3230 -> [w3297]
          tunnel: w3228 -> [w3294]
          tunnel: w3224 -> [w3290]
          tunnel: w3226 -> [w3291]
          tunnel: w3225 -> [w3284]
          tunnel: w3223 -> [w3283]
          tunnel: w3222 -> [w3282]
          tunnel: w3221 -> [w3273]
          i -> [w3298]
          stop <- w3287 stop-if-true
          # "enqueue data"
          # "send data for processing"
          n1444 = Tick Count (ms)() -> (millisecond timer value=w3289:u32)
          n1445 = Subtract(x=w3289, y=w3301) -> (x-y=→"Aquisition loop timing(ms)":u32)
          n1446 = Multiply(x=w3299, y=w3298) -> (x*y=w3292:i32)
          "Fetch Record #" <- w3292
          n1447 = property on="Property Node" class="niScope"(reference=w3306, error in=w3284, "Fetch Record Number"=w3292) -> (reference out=w3312:refnum<k15>, error out=w3311:errorcluster, "Records Done"=w3276:i32)
          "Fetch:Records Done" <- w3276
          n1448 = Subtract(x=w3276, y=w3292) -> (x-y=→"Record Backlog":i32)
          n1449 = call-poly <instrlib>:"niScope Fetch (poly).vi"("timeout"=w3273, "error in"=w3311, "channels"=w3282, "instrument handle"=w3312) -> ("error out"=w3288:errorcluster, "wfm"=w3281:i16[][])  [unwired: 4 in, 2 out]
          n1450 = case shown="\"Ch3\"" w3283 {
            tunnel: w3307 -> [_ w3328 w3338]
            tunnel: [w3319 w3327 w3337] -> w3302
            tunnel: w3292 -> [_ w3326 w3336]
            tunnel: w3288 -> [w3320 w3325 w3335]
            tunnel: [w3320 w3324 w3334] -> w3278
            tunnel: w3281 -> [w3319 _ _]
            tunnel: w3273 -> [_ w3322 w3332]
            tunnel: [0 ("Records Done") w3321 w3331] -> w3272
            frame "Ch1", "Ch2", Default {
            }
            frame "Ch3" {
              n1451 = property on="Property Node" class="niScope"(reference=w3328, error in=w3325, "Fetch Record Number"=w3326) -> (reference out=w3330:refnum<k15>, error out=w3323:errorcluster, "Records Done"=w3321:i32)
              n1452 = call-poly <instrlib>:"niScope Fetch (poly).vi"("timeout"=w3322, "error in"=w3323, "channels"="0", "instrument handle"=w3330) -> ("error out"=w3324:errorcluster, "wfm"=w3327:i16[][])  [unwired: 4 in, 2 out]
            }
            frame "Ch4" {
              n1453 = property on="Property Node" class="niScope"(reference=w3338, error in=w3335, "Fetch Record Number"=w3336) -> (reference out=w3340:refnum<k15>, error out=w3333:errorcluster, "Records Done"=w3331:i32)
              n1454 = call-poly <instrlib>:"niScope Fetch (poly).vi"("timeout"=w3332, "error in"=w3333, "channels"="1", "instrument handle"=w3340) -> ("error out"=w3334:errorcluster, "wfm"=w3337:i16[][])  [unwired: 4 in, 2 out]
            }
          }
          "Fetch:Records Done 2" <- w3272
          n1455 = call "V1FGV.vi"("action (write)"=enum16{"write", "read"}."read" ("action")) -> ("V1 out"=w3275:dbl)  [unwired: 9 in, 1 out]
          n1456 = Enqueue Element(queue=w3294, element=w3275, error in (no error)=w3278) -> (error out=w3293:errorcluster)  [unwired: 1 in, 2 out]
          n1457 = Divide(x=w3302, y=65536) -> (x/y=w3304:dbl[][])
          n1458 = Multiply(x=w3304, y=w3290) -> (x*y=w3303:dbl[][])
          n1459 = Add(x=w3303, y=w3291) -> (x+y=w3279:dbl[][])
          n1460 = Bundle(w3298, w3279) -> (w3277:cluster{i32, dbl[][]})  [unwired: 1 in]
          n1461 = case shown="True" "SaveData?" {
            tunnel: w3297 -> [_ w3317]
            tunnel: [w3313 w3316] -> w3286
            tunnel: w3279 -> [_ w3315]
            tunnel: w3278 -> [w3313 w3314]
            frame False {
            }
            frame True {
              n1462 = Enqueue Element(queue=w3317, element=w3315, error in (no error)=w3314) -> (error out=w3316:errorcluster)  [unwired: 1 in, 2 out]
            }
          }
          n1463 = Send Notification(notification=w3277, notifier=w3310, error in (no error)=w3286) -> (notifier out=w3309:refnum<notifier>, error out=w3285:errorcluster)
          n1464 = Merge Errors(w3293, w3285) -> (w3296:errorcluster)
          n1465 = case shown="Error .." w3296 {
            selector: w3296 -> [w3341 w3342]
            tunnel: w3305 -> [_ w3345]
            tunnel: [w3341 w3342] -> w3287
            frame No Error {
            }
            frame Error {
              # "Send user event to signal aquisition has stoped"
              n1466 = Generate User Event(priority (normal)=usereventprio."high priority", user event=w3345, event data cluster=TRUE ("event data")) -> ()  [unwired: 1 in, 2 out]
            }
          }
          "aquisition loop Error Out" <- w3287
        }
      }
    }
    n1467 = Unbundle By Name(w3204) -> ("status"=w3203:bool)
    n1468 = Not(x=w3203) -> (.not. x?=w3202:bool)
    n1469 = local write "Aq Loop?"(w3202) -> ()
    "Aq Loop?" <- TRUE ("Aq L?")
  }
  n1470 = Close File(refnum=w10, error in=w11) -> (error out=w7:errorcluster)  [unwired: 1 out]
  n1471 = Release Queue(queue=w6, error in (no error)=w7) -> ()  [unwired: 1 in, 3 out]
  n1472 = Unregister For Events(event registration refnum=w30, error in=w40) -> (error out=w41:errorcluster)
  n1473 = Release Notifier(notifier=w35, error in (no error)=w33) -> (error out=w34:errorcluster)  [unwired: 1 in, 2 out]
  n1474 = call <vilib>:"Simple Error Handler.vi"("error in (no error)"=w34) -> ()  [unwired: 4 in, 5 out]
  n1475 = Destroy User Event(user event=w27, error in=w41) -> ()  [unwired: 1 out]
  n1476 = Release Notifier(notifier=w48, error in (no error)=w47) -> (error out=w46:errorcluster)  [unwired: 1 in, 2 out]
  n1477 = Unregister For Events(event registration refnum=w52, error in=w50) -> (error out=w51:errorcluster)
  n1478 = call <vilib>:"Simple Error Handler.vi"("error in (no error)"=w46) -> ()  [unwired: 4 in, 5 out]
  n1479 = Destroy User Event(user event=w42, error in=w51) -> ()  [unwired: 1 out]
